vi "myRIO_BRig_RT_v0,44__PortC.vi"() -> ()   [LabVIEW 2014]
uses:
  myRIO_BRig_RT__Case_Exp_stateList.ctl
  myRIO_BRig_RT__Case_NonExp_stateList.ctl
  <vilib>/Platform/TimedLoop/XDataNode/timing_clust.ctl
  <vilib>/Platform/TimedLoop/XDataNode/nitl_modes.ctl
  <vilib>/Platform/TimedLoop/XDataNode/wakeup.ctl
  <vilib>/WebDAVClient/Advanced/SessionHandle.ctl
  <vilib>/myRIO/Common/Instrument Driver Framework/myRIO v1.0/UART/vis/myRIO v1.0 Close UART.vi
  <vilib>/FPGAPlugInAG/myRIO-1900/niLvFpga_Open_myRIO-1900.vi
  <vilib>/rvi/interface/common/dynamic/niFpgaDynamicAddResources.vi
  <vilib>/Utility/error.llb/Error Cluster From Error Code.vi
  <vilib>/rvi/errors/niLvFpgaAdjustHostInterfaceError.vi
  <vilib>/FPGAPlugInAG/Dynamic/niLvFpga_Close_Dynamic.vi
  <vilib>/myRIO/Common/Instrument Driver Framework/Utilities/vis/FPGA Ref Manager.vi
  <vilib>/myRIO/Common/Instrument Driver Framework/myRIO v1.0/myRIO v1.0 Reset FPGA.vi
  <vilib>/myRIO/Common/Instrument Driver Framework/myRIO v1.0/IRQ/vis/myRIO v1.0 IRQ Info FGV.vi
  <vilib>/myRIO/Common/Instrument Driver Framework/myRIO v1.0/IRQ/vis/myRIO v1.0 Timer IRQ Info FGV.vi
  <vilib>/myRIO/Common/Instrument Driver Framework/myRIO v1.0/IRQ/vis/myRIO v1.0 ISR Agent.vi
  <vilib>/rvi/interface/nirviOpenFPGA/nirviOpenFPGA.xnode
  myRIO_BRig_FPGA_v3,40__PortC__build.lvbitx
  myRIO_BRig_FPGA_v3,40.vi
  <vilib>/rvi/interface/nirviReadWriteControl/nirviReadWriteControl.xnode
  <vilib>/Platform/TimedLoop/XDataNode/XDataNode.xnode
  <vilib>/rvi/interface/nirviCloseFPGA/nirviCloseFPGA.xnode
  <vilib>/Platform/TimedLoop/XDataNode/XDNodeRunTimeDep.lvlib
  <vilib>/rvi/interface/Simulation/niFpgaSimulationCallBeginRW.vi
  <vilib>/myRIO/Instrument Drivers/Utilities/Utilities.lvlib
  <vilib>/WebDAVClient/NI_WebDAV.lvlib
  NiFpgaLv.dll
panel:
  in  "laser_power":dbl
  in  "f_millisec2count":dbl=109.0
  in  "laser_Tshutter":dbl=2.0
  in  "laser_Freq":dbl=10.0
  in  "laser_Tpeak":dbl=2.0
  in  "laser_duration":u16
  out "error out":errorcluster
  in  "LC_Cue1_All_Count":u16
  in  "LC_Cue1_First_Count":u16
  in  "LC_Cue1_All_delayOpt":bool
  in  "LC_ENL1_All_delayOpt":bool
  in  "LC_ENL1_All_Count":u16
  in  "LC_ENL1_First_Count":u16
  in  "LC_Cue1_First_delayOpt":bool
  in  "LC_ENL1_First_delayOpt":bool
  in  "Tcycle_Cue_max":u16=1000 caption="Max [ms]" min=5 max=5000 step=5
  in  "Tcycle_Cue_min":u16=1000 caption="Min [ms]" min=5 max=5000 step=5
  in  "SendData":bool
  out "cSpout":enum16{"Left", "Right"}(ring) caption="Left or Right Spout"
  out "A4":u32 caption="LickCounter_Right"
  out "A2":u32 caption="LickCounter_Left"
  in  "tDelay_laser_wro":u32
  in  "tCycle_laser_wro":u32=1000
  in  "tDelay_laser_rew":u32
  in  "laserResponse_wrong_LED":bool
  out "error_initTrial":errorcluster
  out "error_Selection_pre":errorcluster
  out "error_Selection":errorcluster
  in  "tCycle_laser_rew":u32=1000
  out "SelectWrong":bool
  out "SelectReward":bool
  in  "Left(F)_or_Right(T)":bool
  in  "ignoreWrong":bool
  in  "SelectionState":bool
  in  "laserResponse_wrong":bool
  in  "laserResponse_reward":bool
  in  "laserResponse_reward_LED":bool
  out "nRewards_Right":u16 caption="# Rewards Total (Right)"
  out "nRewards_Left":u16 caption="# Rewards Total (Left)"
  out "nRewards_cur":u16 caption="# Rewards in Current Block"
  out "TpB_target":u16 caption="Target Trials Per Block"
  out "cState_NonExp":T1 caption="NonExperimental State"
  out "iBlock":u16 caption="Current Block"
  out "cState":T2 caption="Experimental State"
  out "iTrial":u16 caption="Current Trial"
  in  "warmupType":bool
  in  "TestConnection":bool
  in  "warmup":bool caption="WarmUp"
  in  "Host Filename Prefix":string="Exp1_TM2"
  out "Connected To Host?":bool
  in  "Host Password":string="sabalab"
  in  "Host UserName":string="Test2"
  in  "sp_RightSpout":u16(slide)=2 max=2 step=1 scale=0.0..2.0
  in  "sp_LeftSpout":u16(slide)=2 max=2 step=1 scale=0.0..2.0
  in  "BUR_max":u16 caption="Count Reward Structure  (0 = off)"
  in  "LC_Wrong_Probability":u16
  in  "LC_Wrong_Trial":u16(slide) max=2 step=1 scale=0.0..2.0
  in  "LC_Wrong_Block":u16(slide) max=2 step=1 scale=0.0..2.0
  in  "LC_Wrong_OnOff":bool
  in  "LC_Reward_Probability":u16
  in  "LC_Reward_Trial":u16(slide) max=2 step=1 scale=0.0..2.0
  in  "LC_Reward_Block":u16(slide) max=2 step=1 scale=0.0..2.0
  in  "LC_Reward_OnOff":bool
  in  "LC_Cue1_All_Probability":u16
  in  "LC_Cue1_All_Block":u16(slide) max=2 step=1 scale=0.0..2.0
  in  "LC_Cue1_All_OnOff":bool
  in  "LC_Cue1_First_Probability":u16
  in  "LC_Cue1_First_Block":u16(slide) max=2 step=1 scale=0.0..2.0
  in  "LC_Cue1_First_OnOff":bool
  in  "LC_ENL1_All_Probability":u16 max=100 step=1
  in  "LC_ENL1_All_Block":u16(slide) max=2 step=1 scale=0.0..2.0
  in  "LC_ENL1_All_OnOff":bool
  in  "LC_ENL1_First_Probability":u16 max=100 step=1
  in  "LC_ENL1_First_Block":u16(slide) max=2 step=1 scale=0.0..2.0
  in  "A6":bool caption="Activate Recording?\n(Select Prior to\nStarting Experiment)"
  in  "Tcycle_Timeout":u16=1000 caption="Timeout Time [ms]" min=10 max=10000 step=1
  in  "Tcycle_Wrong":u16=1000 caption="Wrong Time [ms]" min=10 max=10000 step=1
  in  "Tcycle_Selection":u16=1000 caption="Answer Time [ms]" min=1 max=10000 step=1
  in  "Tcycle_RewardPost":u16=1000 caption="Consumption Time [ms]" min=250 max=10000 step=250
  in  "Tcycle_Reward_L":u16=500 caption="Reward Time [ms]" min=1 max=1000 step=1
  in  "Tcycle_Reward_R":u16=500 caption="Reward Time [ms]" min=1 max=1000 step=1
  in  "TpB_Max_R":u16=4 caption="Max TrialsPerBlock" min=1 max=12 step=1
  in  "TpB_Min_R":u16=4 caption="Min TrialsPerBlock" min=1 max=12 step=1
  in  "TpB_Max_L":u16=4 caption="Max TrialsPerBlock" min=1 max=12 step=1
  in  "TpB_Min_L":u16=4 caption="Min TrialsPerBlock" min=1 max=12 step=1
  in  "BUR_min":u16 caption="Count Reward Structure  (0 = off)"
  in  "TrialUntilReward":bool caption="Ignore Wrong \nSelection"
  in  "CueCycles":u16=1 caption="Cue Structure" min=1 max=1 step=1
  in  "MTrig_Laser_Tcycle":u16=10 caption="Time [ms]"
  in  "MTrig_Laser_trig":bool
  in  "MTrig_Audio_trig__R":bool caption="Trigger Audio"
  in  "MTrig_Audio_trig__L":bool caption="Trigger Audio"
  in  "RewCalib_Trig_R":bool caption="Calibrate_R"
  in  "RewCalib_Trig_L":bool caption="Calibrate_L"
  in  "MTrig_Solenoid_Tcycle__R":u16=300 caption="Time [ms]"
  in  "MTrig_Solenoid_Tcycle__L":u16=300 caption="Time [ms]"
  in  "MTrig_Solenoid_trig__R":bool caption="Solenoid"
  in  "MTrig_Solenoid_trig__L":bool caption="Solenoid"
  in  "STOP_abort":bool caption="Stop LabView\n(Stops myRio and FPGA)"
  in  "STOP_endBlock":bool caption="Stop Experiment\n@ End of Block"
  in  "STOP_endTrial":bool caption="Stop Experiment\n@ End of Trial"
  in  "START":bool caption="Start Experiment"
  in  "Tcycle_CuePenalty":u16=1000 caption="Penalty [ms]" min=1 max=10000 step=1
  in  "Audio_Amp__R":u16=100 caption="Amp"
  in  "Audio_Freq__R":u16=5 caption="Freq [kHz]" max=14 step=1
  in  "Audio_Amp__L":u16=100 caption="Amp"
  in  "Audio_Freq__L":u16=5 caption="Freq [kHz]" max=14 step=1
  in  "LC_Wrong_Tdelay":u16
  in  "LC_Cue1_All_Tdelay":u16
  in  "LC_ENL1_All_Tdelay":u16
  in  "LC_Reward_Tdelay":u16
  in  "LC_Cue1_First_Tdelay":u16
  in  "LC_ENL1_First_Tdelay":u16
  in  "LC_ENL1_First_OnOff":bool
  in  "Tcycle_ENLPenalty":u16=100 caption="Penalty [ms]" min=10 max=100 step=10
  in  "Tcycle_ENL_max":u16=1000 caption="Max [ms]" min=250 max=10000 step=250
  in  "Tcycle_ENL_min":u16=1000 caption="Min [ms]" min=250 max=10000 step=250
  # "Manual Control"
  # "Task Structure"
  # "Task Timing"
  # "Laser Control\n\n                                                    On/Off      Block        Probability [%]   Delay [ms]                              Count"
  # "Manual Solenoid Trigger\nLeft              Right"
  # "Master Structure"
  # "Enforced NonLick"
  # "Enforced NonLick 1"
  # "from end"
  # "Time = Cue Min"
  # "Min\n \n  \nMax"
  # "First Trial"
  # "from start"
  # "(1) = Switching\n(2) = Two Choice"
  # "from end"
  # "All Trials"
  # "Cue"
  # "from start"
  # "Cue 1"
  # "from end"
  # "from start"
  # "Cue then reward"
  # "Min"
  # "Max"
  # "from end"
  # "Cue with reward"
  # "Trial Per Block Structure\n       Left                    Right"
  # "from start"
  # "Spout Selection Control"
  # "Manual Speaker Trigger\nLeft              Right"
  # "Selection Reward"
  # "Answer Time\n         [ms]\n\n  \nWrong Choice Penalty\n         [ms]\n \n \nChoice Timeout Penalty\n         [ms]"
  # "Selection Wrong"
  # "Cue Control"
  # "Left              Right"
  # "State"
  # "Manual Laser Trigger"
  # "Freq [kHz]\n \n \nAmp\n \n\n \n\nSpeaker\nSetting"
  # "Reward Control\n                 Left              Right"
  # "Min = 1\nMax = 32k"
  # "Reward Time\n         [ms]"
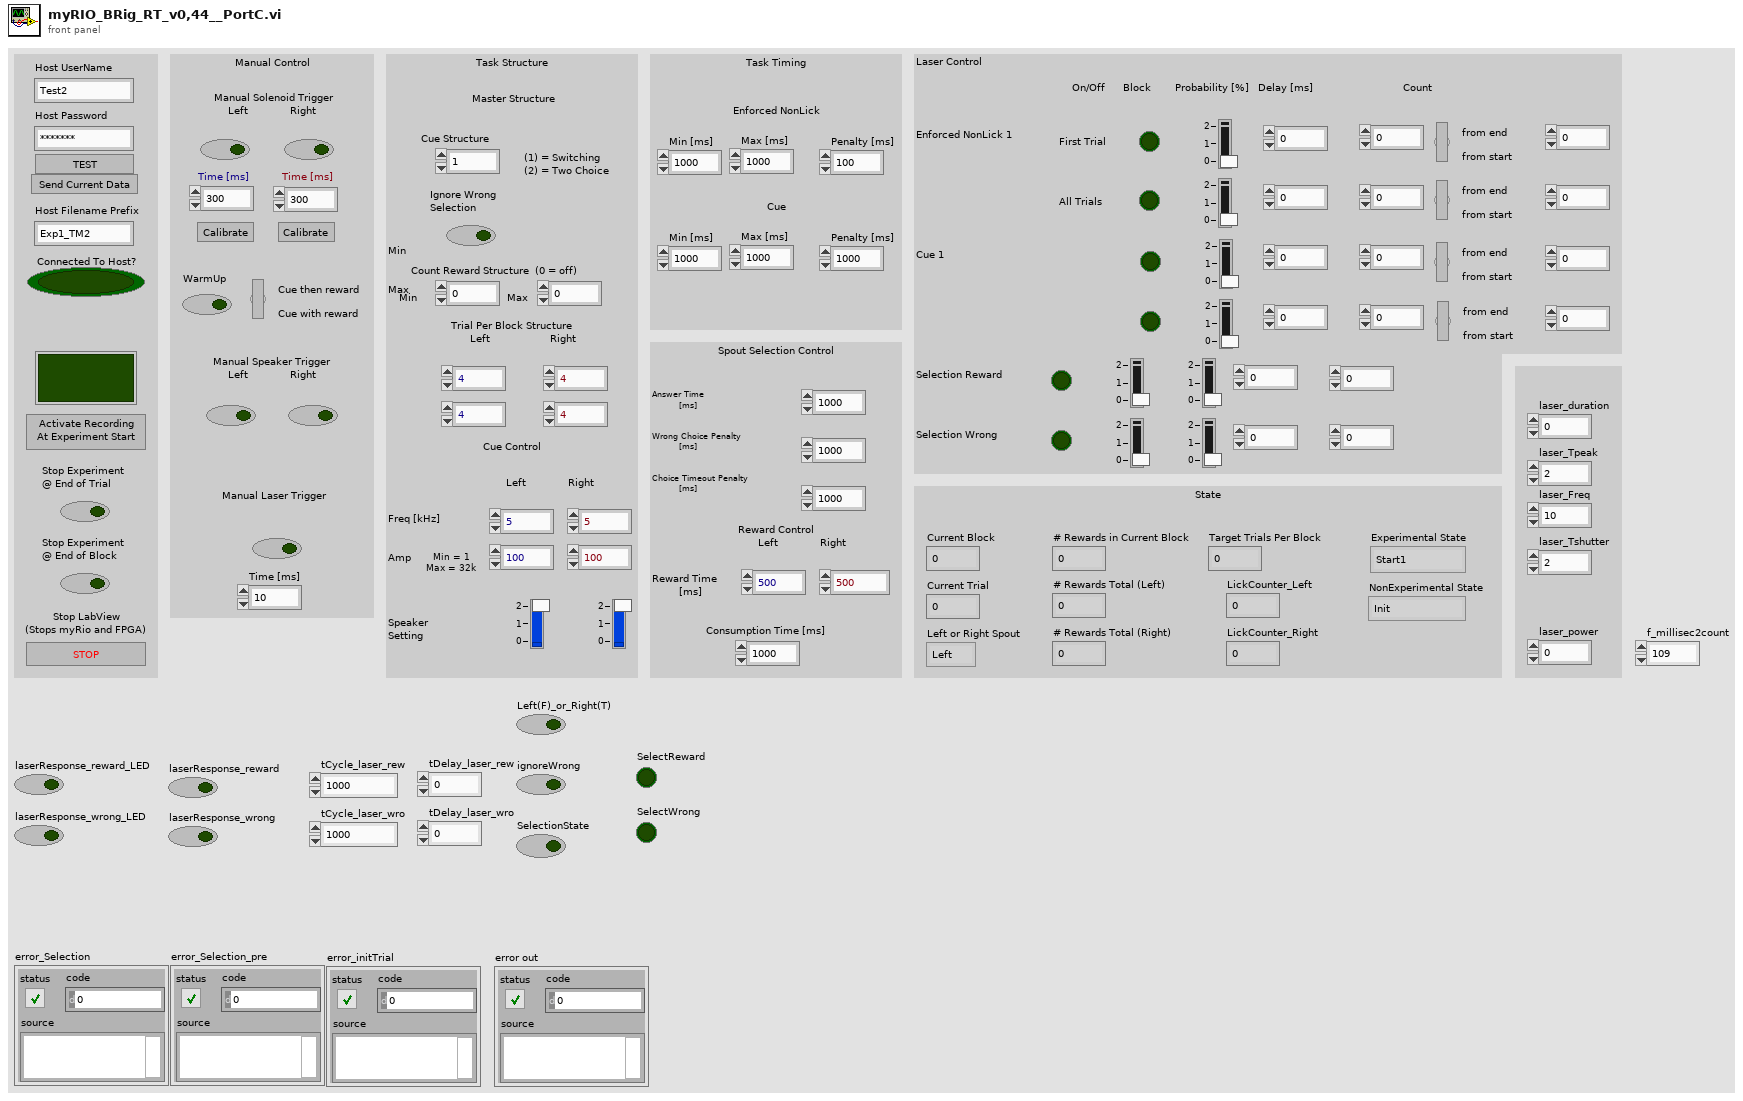
[diagram p1: front panel]
types:
  T1 = typedef "myRIO_BRig_RT__Case_NonExp_stateList.ctl" = enum16{"Init", "UploadSettings_pre", "UploadSettings_Read_dataExp", "UploadSettings_dataExp_1", "UploadSettings_Read_dataLC", "UploadSettings_dataLC_1", "UploadSettings_dataLC_2", "UploadSettings_Read_dataMTrig", "UploadSettings_dataMTrig_1", "UploadSettings_post", "Idle_pre", "IdleEmpty", "IdleEmpty2", "IdleEmpty3", "IdleEmpty4", "Idle", "Idle_2", "Idle_3", "Idle_4", "Idle_post", "Cue_pre__pre", "Cue_pre", "Cue", "Cue_post", "RewardCalibration_pre", "DispenseWater_pre__pre", "DispenseWater_pre", "DispenseWater", "DispenseWater_post", "TestConnection", "SendData", "End"}
  T2 = typedef "myRIO_BRig_RT__Case_Exp_stateList.ctl" = enum16{"Start1", "Start2", "Start3", "saveSettings1", "saveSettings2", "saveSettings3", "saveSettings4_LC_ENL", "saveSettings5_LC_Cue", "saveSettings6_LC_Other", "setSettings_Audio", "setSettings_Laser", "initBlock_pre", "initBlock", "initBlock2", "initBlock_post", "initTrial_pre", "initTrial", "initTrial2", "initTrial3", "initTrial4", "initTrial_LC_ENL1", "initTrial_LC_Cue1", "initTrial_post", "ENL1_pre", "ENL1", "ENL1_post", "ENL1Penalty_pre", "ENL1Penalty", "ENL2_pre", "ENL2", "ENL2Penalty_pre", "ENL2Penalty", "Cue1_pre", "Cue1", "Cue1_post", "Cue1Penalty_pre", "Cue1Penalty", "Cue2_pre", "Cue2", "Cue2Penalty_pre", "Cue2Penalty", "Selection_pre", "Selection", "Select_post", "SelectReward_pre", "SelectReward", "SelectRewardPost_pre", "SelectRewardPost", "SelectWrong_pre", "SelectWrong", "SelectWrong_post", "SelectTimeout_pre", "SelectTimeout", "SelectTimeout_post", "endTrial_pre", "endTrial1", "endTrial2", "endTrial3", "endTrial_post", "endBlock_pre", "endBlock", "endBlock_post", "endExp", "commConnect", "commUpload_pre", "commUpload_dataBlock", "commUpload_dataCurrent", "commUpload_dataExp", "commUpload_dataLC", "commUpload_dataTrial", "commUpload_post", "saveData_pre", "saveData_dataBlock", "saveData_dataCurrent", "saveData_dataExp", "saveData_dataLC", "saveData_dataTrial", "saveData_post"}
  T3 = typedef "XDNodeRunTimeDep.lvlib/timing_clust.ctl" = cluster{"Expected End [f-1]":u64, "Actual End [f-1]":u64, "Finished Late? [f-1]":bool, "Expected End [i-1]":u64, "Actual End [i-1]":u64, "Finished Late? [i-1]":bool, "Expected Start [i]":u64, "Actual Start [i]":u64, "Expected Start [f]":u64, "Actual Start [f]":u64, "Source Name":string, "Structure Name":string, "Period":i64, "Deadline":i64, "Offset":i64, "Start":i64, "Priority":i32, "Timeout":i32, "Mode":T4, "Wakeup Reason":T5, "Error":errorcluster, "Source Type":string, "Secondary Source Type":string, "Global End Time":u64, "Global Start Time":u64, "Frame Duration":u64, "Iteration Duration":u64, "Assigned CPU":i32, "I/O Scan Engine Mode":u32}
  T4 = typedef "XDNodeRunTimeDep.lvlib/nitl_modes.ctl" = enum32{"No Change", "Process missed periods, maintain original phase", "Discard missed periods, maintain original phase", "Process missed periods, ignore original phase", "Discard missed periods, ignore original phase"}
  T5 = typedef "XDNodeRunTimeDep.lvlib/wakeup.ctl" = enum32{"Normal", "Aborted", "Asynchronous wakeup", "Timing source error", "Timed loop error", "Timeout"}
  T6 = typedef "NI_WebDAV.lvlib/SessionHandle.ctl" = refnum<k1>
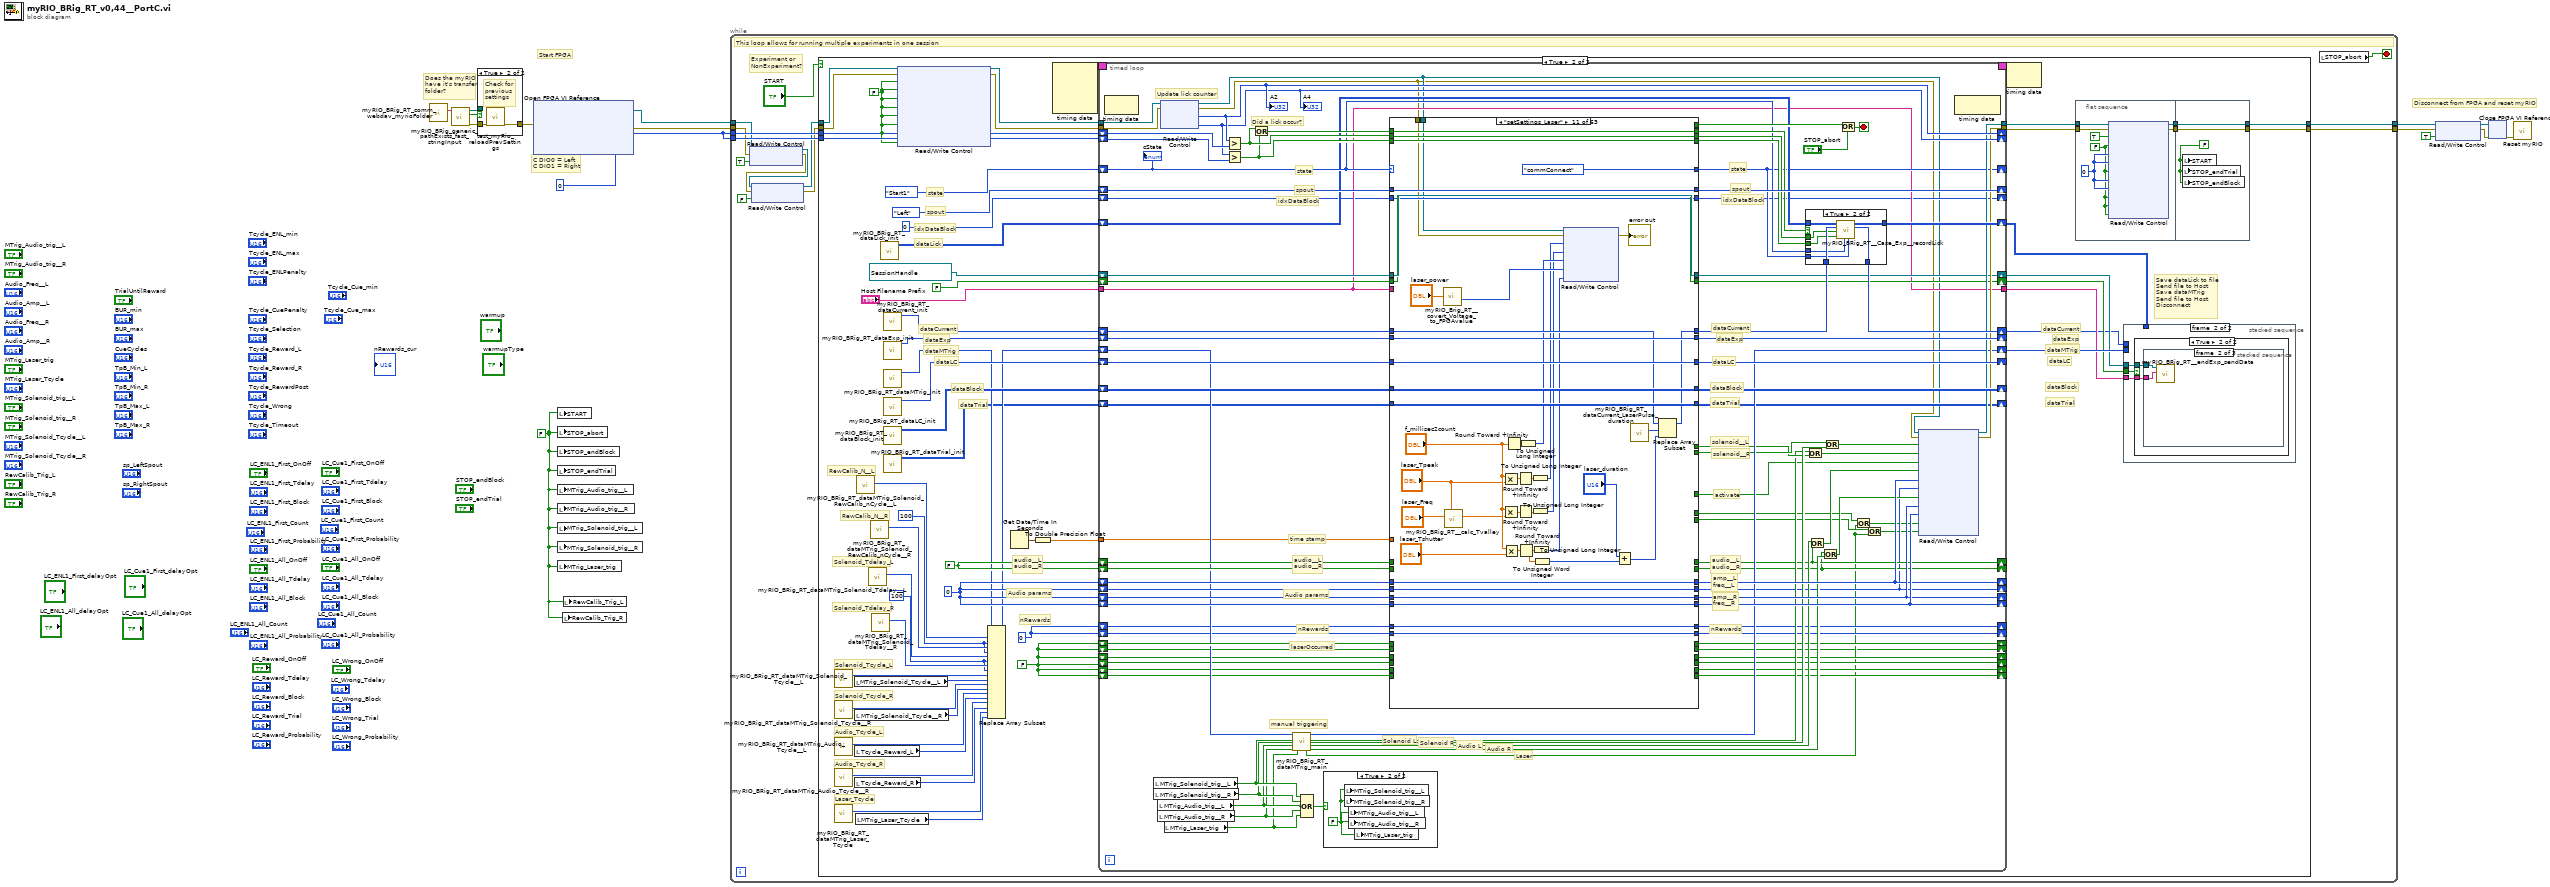
[diagram p0: block diagram]
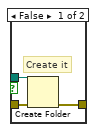
[diagram p2: hidden frame]
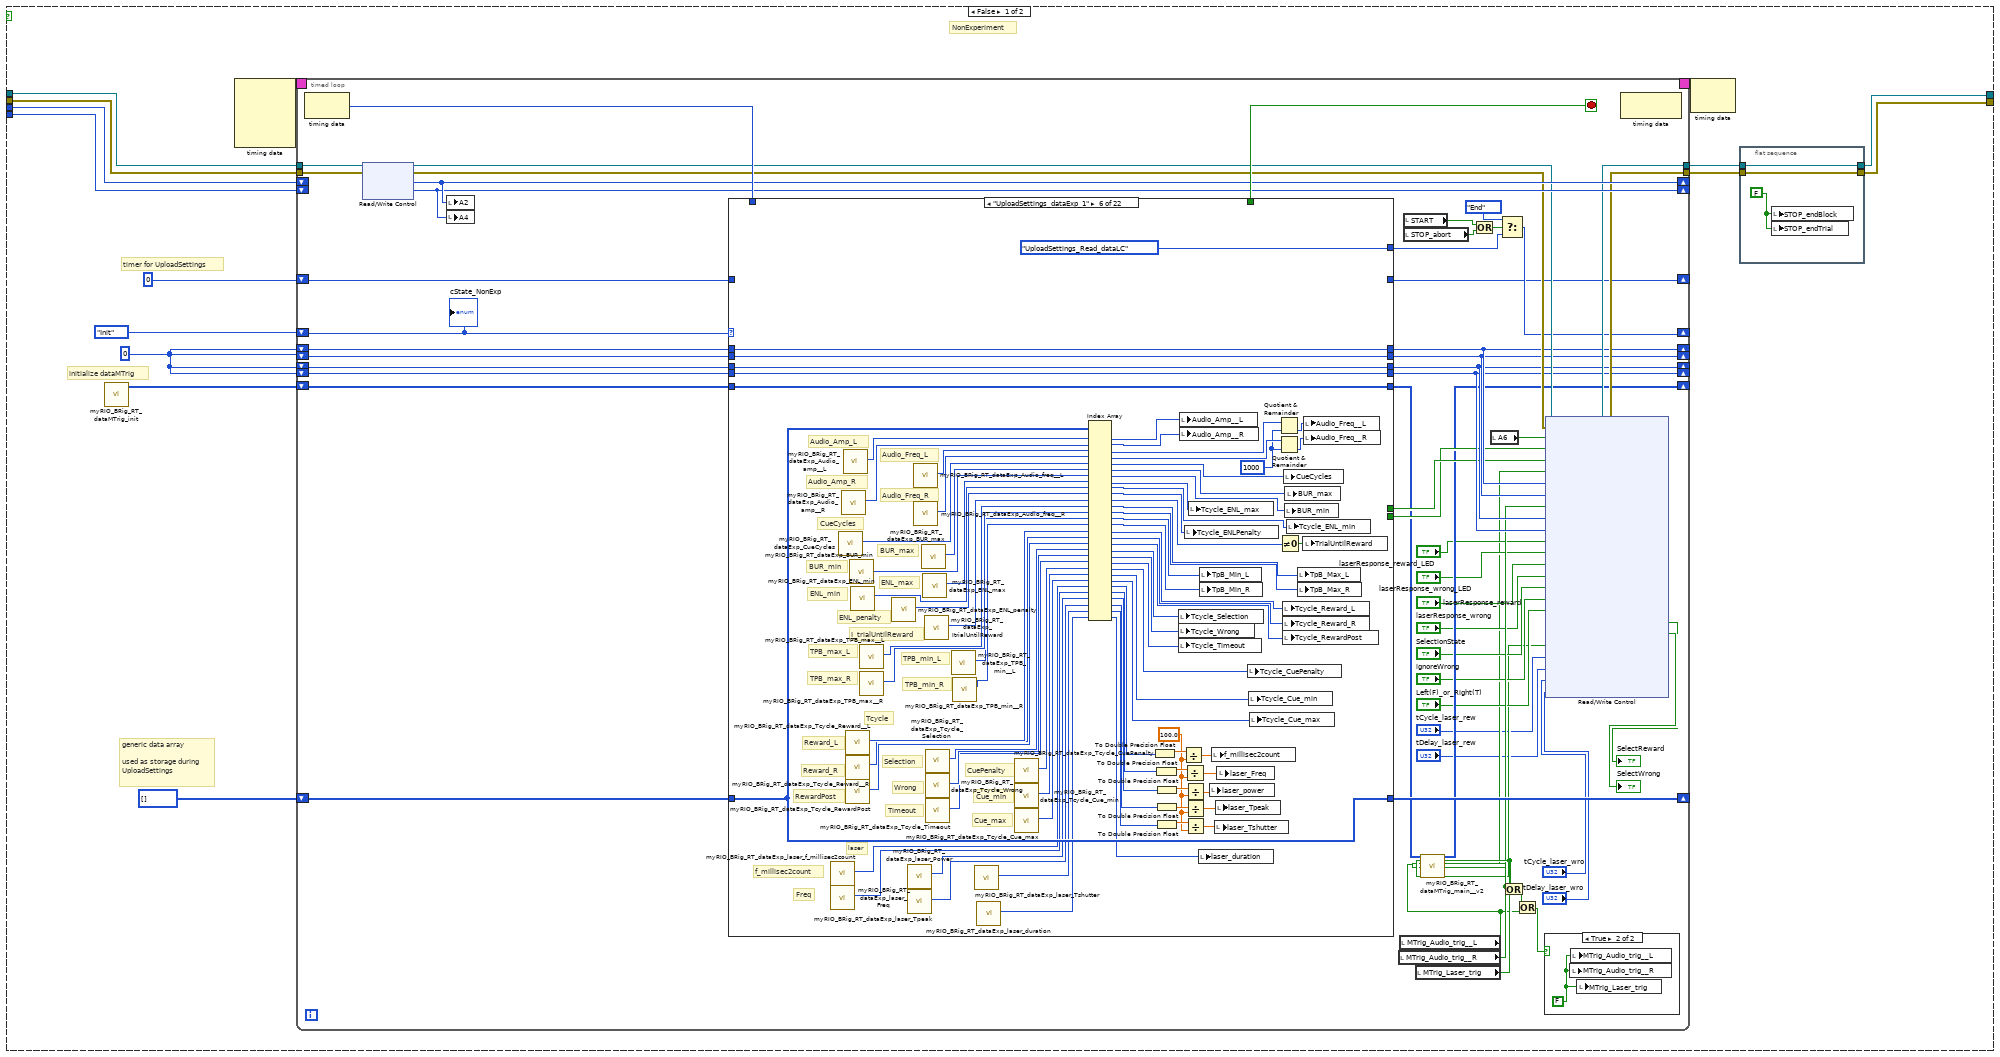
[diagram p3: hidden frame]
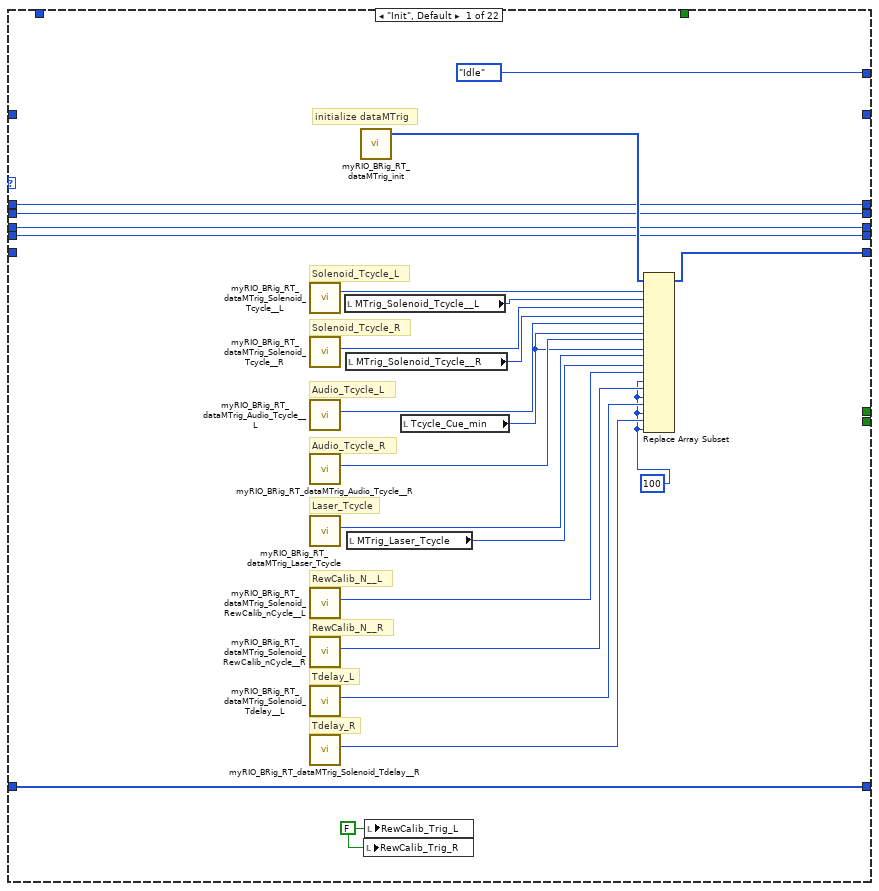
[diagram p5: hidden frame]
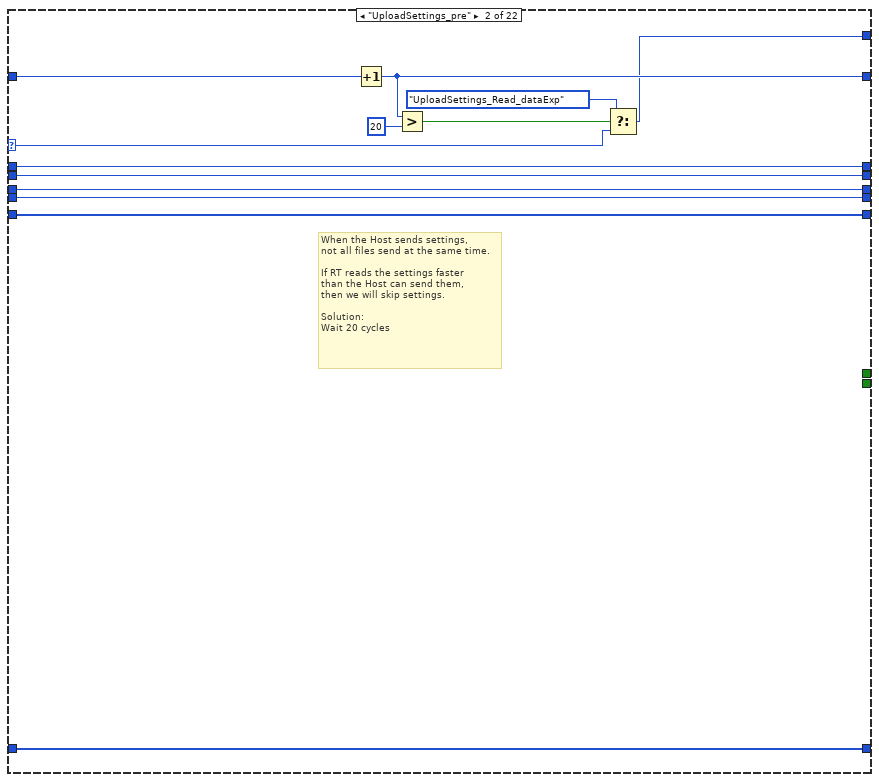
[diagram p6: hidden frame]
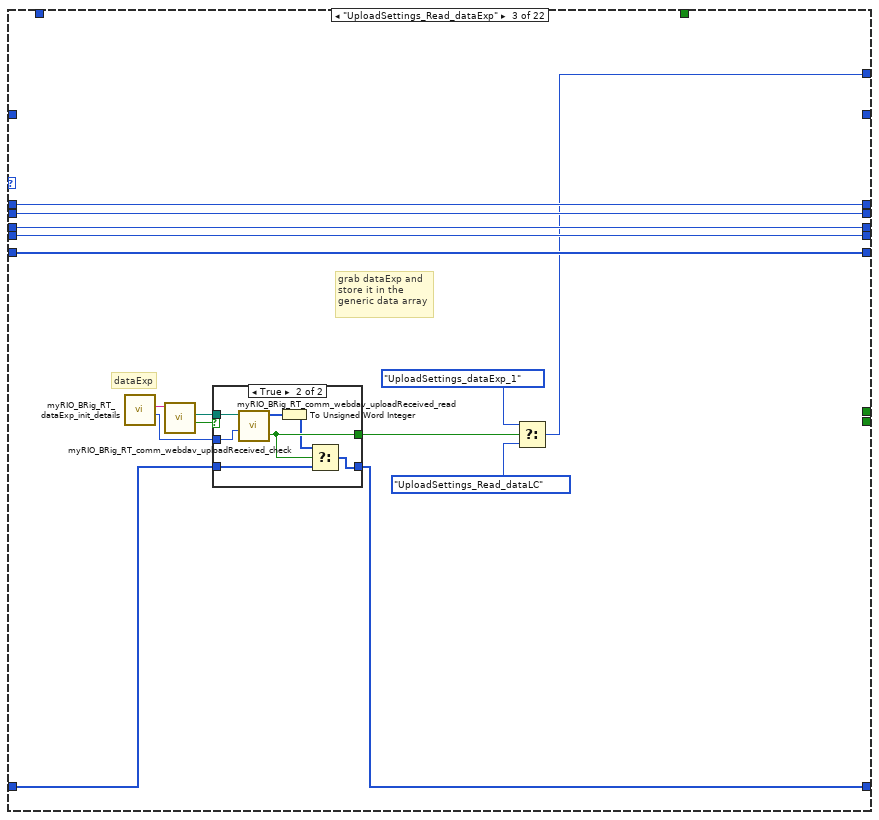
[diagram p7: hidden frame]
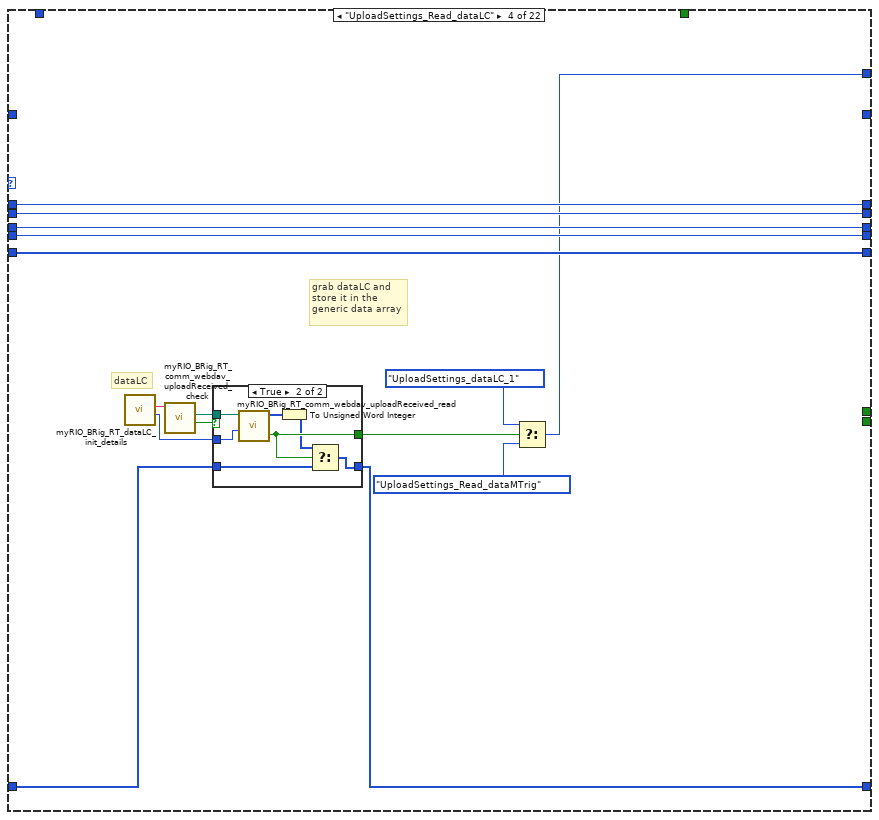
[diagram p9: hidden frame]
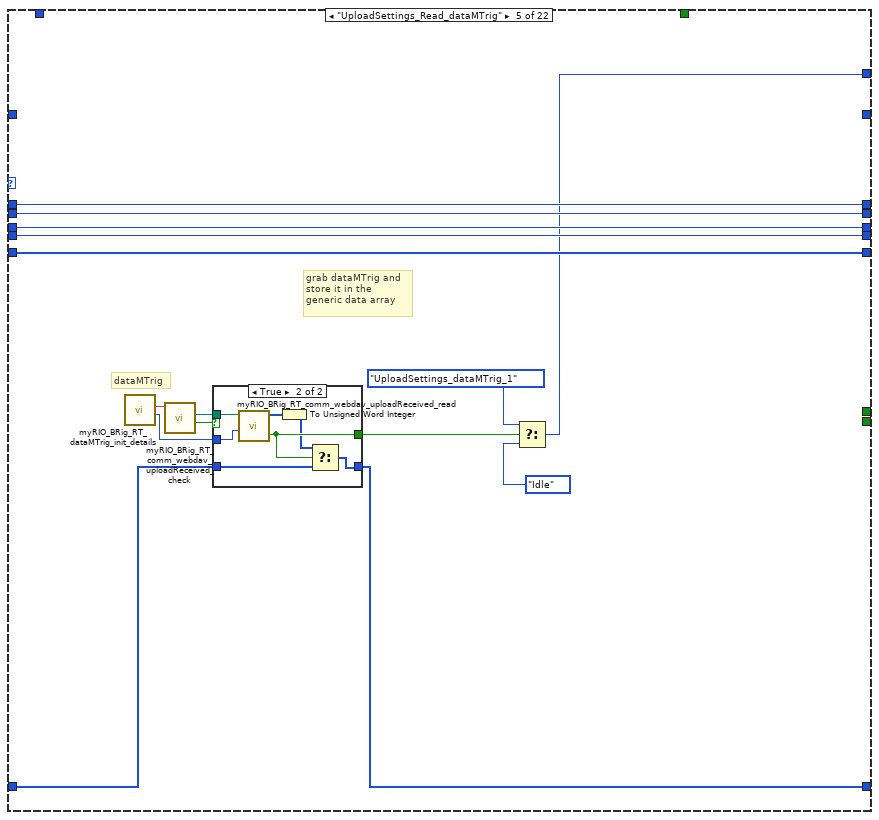
[diagram p11: hidden frame]
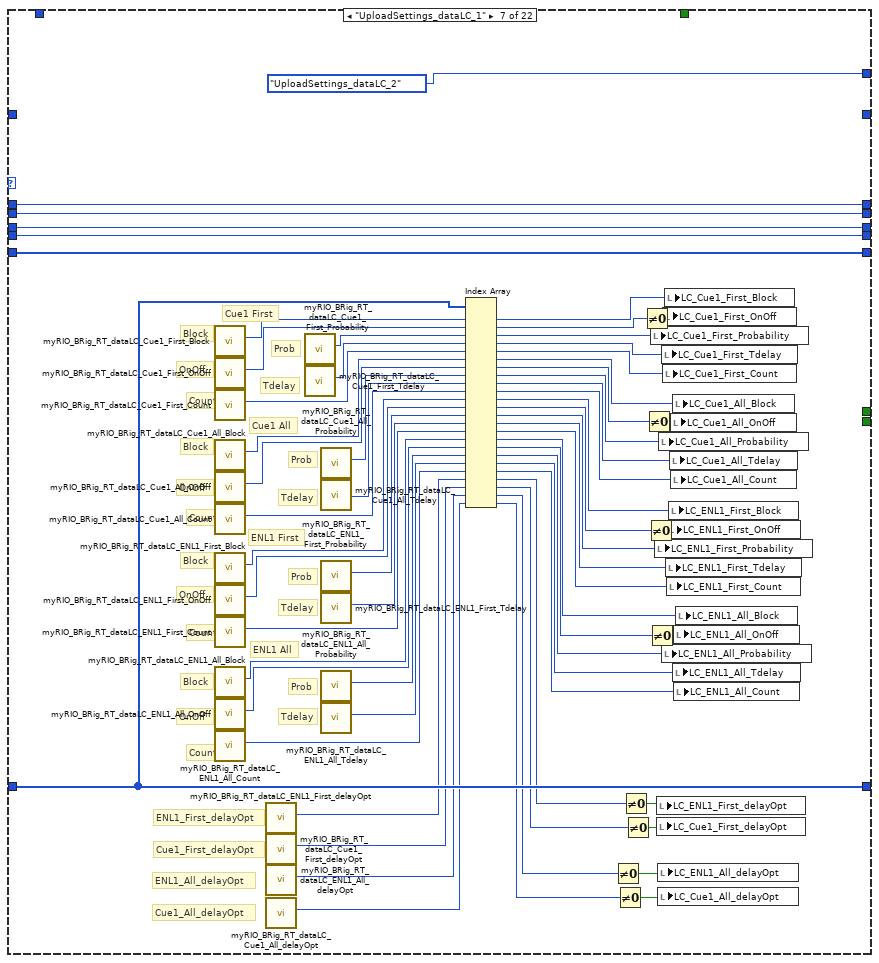
[diagram p13: hidden frame]
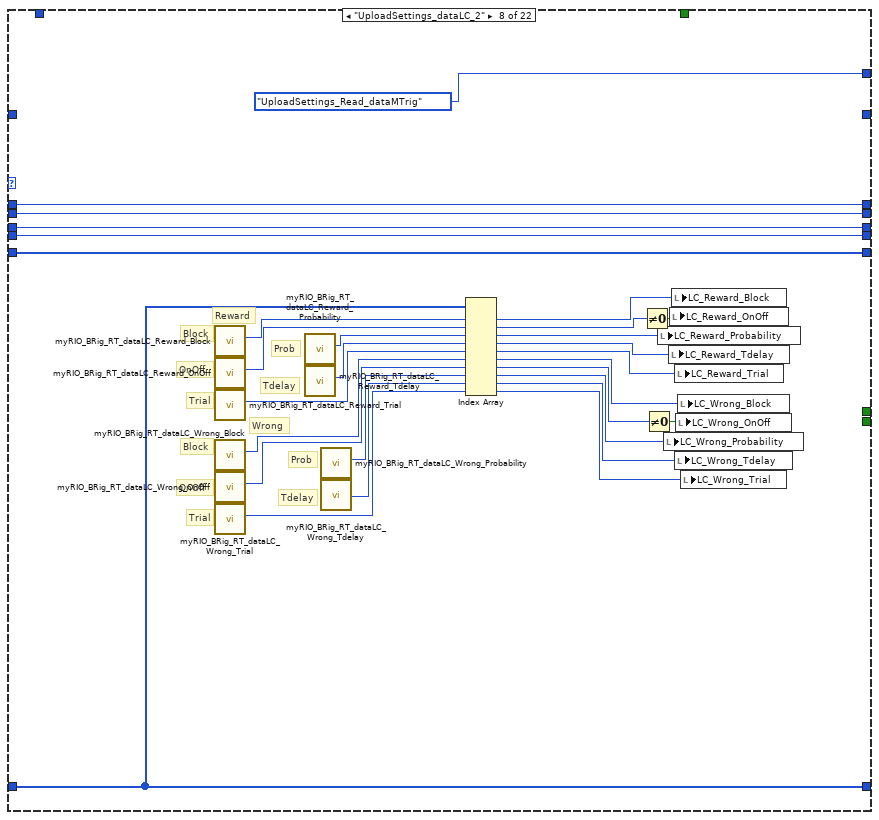
[diagram p14: hidden frame]
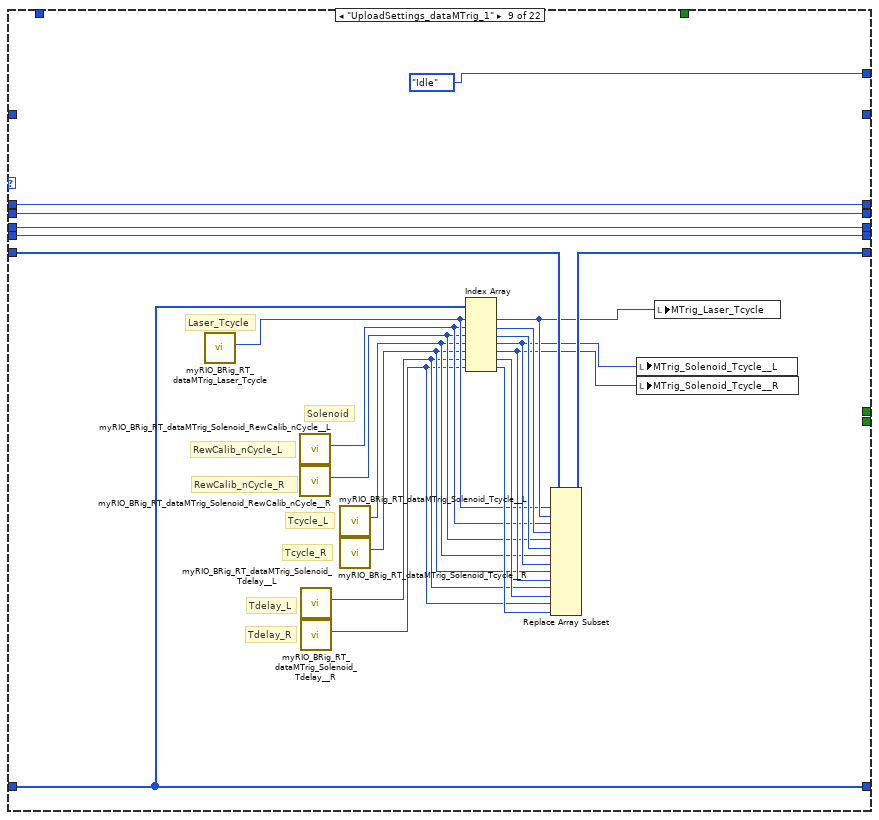
[diagram p15: hidden frame]
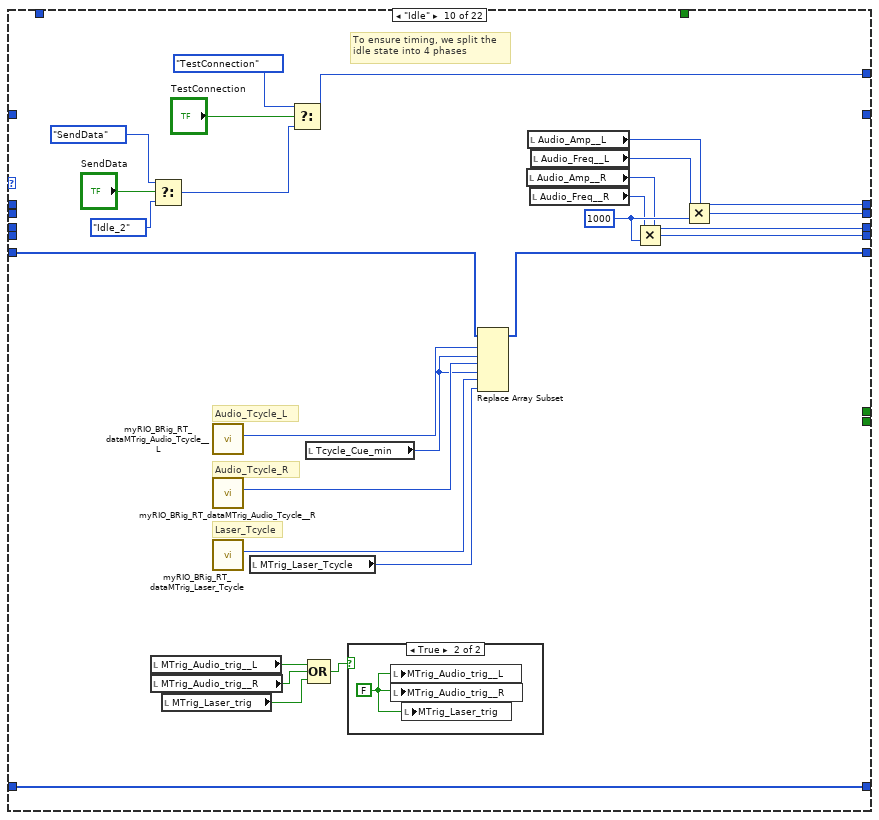
[diagram p16: hidden frame]
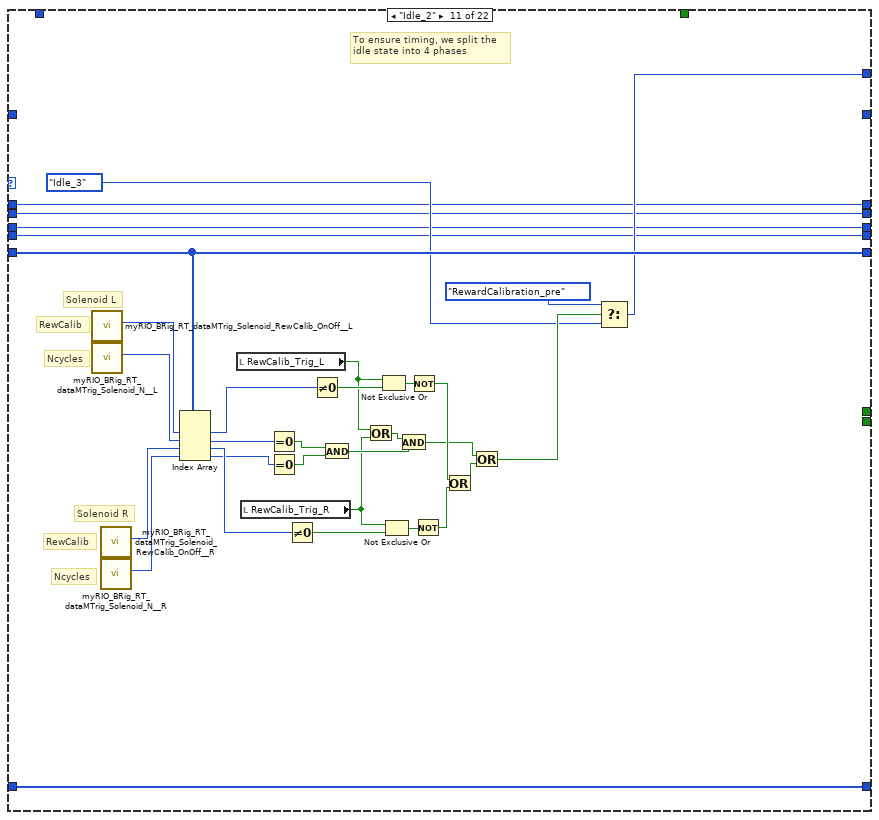
[diagram p18: hidden frame]
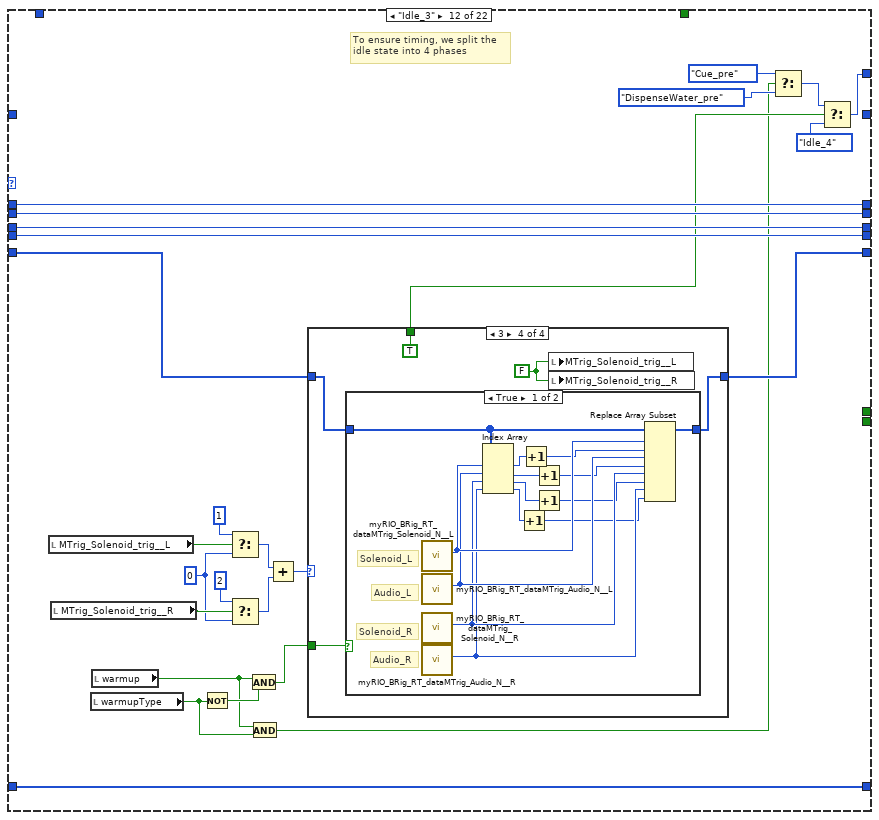
[diagram p19: hidden frame]
diagram:
  w9 = u32 0
  w6 = FALSE
  # "Does the myRIO\nhave it's transfer\nfolder?"
  # "C DIO0 = Left\nC DIO1 = Right"
  # "Start FPGA"
  # "Disconnect from FPGA and reset myRIO"
  n1 = call "myRIO_BRig_RT_comm_webdav_myrioFolder.vi"() -> ("output_myrioFolder"=w4:string)  [unwired: 11 in]
  n2 = call "myRIO_BRig_generic_pathExists_fast_stringInput.vi"("input_filePath"=w4) -> ("output_error"=w3:errorcluster, "output_Iexist"=w2:bool, "output_filePath"=w1:path)  [unwired: 8 in]
  n3 = case shown="True" w2 {
    tunnel: w1 -> [w18 _]
    tunnel: w3 -> [w17 w20]
    tunnel: [w16 w19] -> w5
    frame False {
      # "Create it"
      n4 = Create Folder(path (use dialog)=w18, error in=w17) -> (error out=w16:errorcluster)  [unwired: 1 in, 2 out]
    }
    frame True {
      # "Check for\nprevious\nsettings"
      n5 = call "test_myRio_reloadPrevSettings.vi"("input_error"=w20) -> ("output_error"=w19:errorcluster)  [unwired: 10 in]
    }
  }
  n6 = xnode "Open FPGA VI Reference"("error in"=w5) -> ("FPGA VI Reference Out"=w11:refnum<k20>, "error out"=w10:errorcluster)  [unwired: 1 in]
  n7 = local write "START"(w6) -> ()
  n8 = local write "STOP_abort"(w6) -> ()
  n9 = local write "STOP_endBlock"(w6) -> ()
  n10 = local write "STOP_endTrial"(w6) -> ()
  n11 = local write "MTrig_Audio_trig__L"(w6) -> ()
  n12 = local write "MTrig_Audio_trig__R"(w6) -> ()
  n13 = local write "MTrig_Solenoid_trig__L"(w6) -> ()
  n14 = local write "MTrig_Solenoid_trig__R"(w6) -> ()
  n15 = local write "MTrig_Laser_trig"(w6) -> ()
  n16 = local write "RewCalib_Trig_R"(w6) -> ()
  n17 = local write "RewCalib_Trig_L"(w6) -> ()
  n18 = while {
    tunnel: w11 -> [w24]
    tunnel: w10 -> [w29]
    tunnel: w9 -> [w32]
    tunnel: w9 -> [w31]
    tunnel: [w22] -> w8
    tunnel: [w21] -> w7
    stop <- w30 stop-if-true
    # "Experiment or\nNonExperiment?"
    # "This loop allows for running multiple experiments in one session"
    n19 = xnode "Read/Write Control"("FPGA VI Reference In"=w24, "error in"=w29, "Counts_Reset"=TRUE) -> ("FPGA VI Reference Out"=w26:refnum<k20>, "error out"=w27:errorcluster)
    n20 = xnode "Read/Write Control"("FPGA VI Reference In"=w26, "error in"=w27, "Counts_Reset"=FALSE) -> ("FPGA VI Reference Out"=w23:refnum<k20>, "error out"=w25:errorcluster)
    n21 = case shown="True" "START" {
      tunnel: w32 -> [w45 w937]
      tunnel: w31 -> [w44 w936]
      tunnel: w25 -> [w42 w887]
      tunnel: w23 -> [w43 w886]
      tunnel: [w40 w933] -> w22
      tunnel: [w38 w928] -> w21
      frame False {
        w37 = u16 0 ("Audio_Amp__L")
        # "generic data array\n\nused as storage during\nUploadSettings"
        # "timer for UploadSettings"
        # "initialize dataMTrig"
        # "NonExperiment"
        n22 = call "myRIO_BRig_RT_dataMTrig_init.vi"() -> ("output_dataMTrig"=w46:u16[])  [unwired: 5 in]
        n23 = node-c288() -> (w49:T3)  [unwired: 4 in]
        n24 = timed-loop {
          timing: w49 -> [_]
          timing-out: [_] -> w48
          shift-right: [w83] -> _
          shift-left: w46 -> [w107]
          shift-right: [w72] -> _
          shift-left: myRIO_BRig_RT__Case_NonExp_stateList."Init" ("Enum") -> [w97]
          shift-right: [w105] -> _
          shift-left: w45 -> [_]
          shift-right: [w104] -> _
          shift-left: w44 -> [_]
          tunnel: [w100] -> w41
          tunnel: [w98] -> w39
          tunnel: w42 -> [w103]
          tunnel: w43 -> [w102]
          shift-right: [w96] -> _
          shift-left: u16[] [] ("output_data") -> [w95]
          shift-right: [w90] -> _
          shift-left: w37 -> [w94]
          shift-right: [w89] -> _
          shift-left: w37 -> [w93]
          shift-right: [w88] -> _
          shift-left: w37 -> [w92]
          shift-right: [w87] -> _
          shift-left: w37 -> [w91]
          shift-right: [w54] -> _
          shift-left: u16 0 ("Audio_Amp__L") -> [w55]
          stop <- w108 stop-if-true
          n25 = node-c288() -> (w106:i64)  [unwired: 1 in]
          n26 = xnode "Read/Write Control"("FPGA VI Reference In"=w102, "error in"=w103) -> ("FPGA VI Reference Out"=w101:refnum<k20>, "error out"=w99:errorcluster, "A2_LickL"=w105:u32, "A4_LickR"=w104:u32)
          n27 = local write "A2"(w105) -> ()
          n28 = local write "A4"(w104) -> ()
          n29 = case shown="\"UploadSettings_dataExp_1\"" w97 {
            selector: w97 -> [_ w141 _ _ _ _ _ _ _ _ _ _ _ _ w596 _ _ w781 _ _ _ w878]
            tunnel: [myRIO_BRig_RT__Case_NonExp_stateList."Idle" ("Enum") w139 w146 w169 w192 myRIO_BRig_RT__Case_NonExp_stateList."UploadSettings_Read_dataLC" ("Enum") myRIO_BRig_RT__Case_NonExp_stateList."UploadSettings_dataLC_2" ("Enum") myRIO_BRig_RT__Case_NonExp_stateList."UploadSettings_Read_dataMTrig" ("f") myRIO_BRig_RT__Case_NonExp_stateList."Idle" ("Enum") w422 w443 w476 w567 myRIO_BRig_RT__Case_NonExp_stateList."Cue" ("t") w595 myRIO_BRig_RT__Case_NonExp_stateList."DispenseWater_pre" ("Enum") w723 w779 w806 myRIO_BRig_RT__Case_NonExp_stateList."Idle" ("Enum") myRIO_BRig_RT__Case_NonExp_stateList."Idle" ("Enum") w878] -> w73
            tunnel: [w124 w134 w156 w179 w202 w296 w359 w388 w408 w433 w458 w487 w565 w583 w609 w633 w760 w786 w817 w860 w870 w876] -> w84
            tunnel: [_ _ _ _ _ _ _ _ _ _ _ _ _ _ _ _ _ _ _ _ _ TRUE] -> w108
            tunnel: w107 -> [_ w134 w156 w179 w202 w296 w359 w388 w409 w432 w458 w488 w565 w584 w609 w619 w756 w787 w818 w860 w870 w876]
            tunnel: w106 -> [_ _ _ _ _ _ _ _ _ _ _ _ _ _ _ _ _ w791 _ _ _ _]
            tunnel: [w113 w133 w147 w170 w193 w240 w311 w360 w389 w417 w438 w470 w560 w571 w594 w610 w708 w764 w799 w848 w864 w871] -> w96
            tunnel: w95 -> [w113 w133 w148 w171 w194 w240 w311 w360 w389 w417 w438 w470 w560 w571 w594 w610 w708 w764 w799 w848 w864 w871]
            tunnel: [w117 w137 w159 w182 w205 w293 w357 w363 w406 w428 w441 w480 w562 w591 w606 w613 w762 w797 w824 w851 w867 w874] -> w89
            tunnel: [w115 w135 w157 w180 w203 w291 w355 w361 w404 w427 w439 w482 w564 w589 w608 w611 w761 w795 w822 w849 w865 w872] -> w87
            tunnel: [w118 w138 w160 w183 w206 w294 w358 w364 w407 w426 w442 w479 w561 w593 w605 w614 w763 w798 w825 w852 w868 w875] -> w90
            tunnel: [w116 w136 w158 w181 w204 w292 w356 w362 w405 w425 w440 w481 w563 w590 w607 w612 w761 w796 w823 w850 w866 w873] -> w88
            tunnel: w94 -> [w118 w138 w160 w183 w206 w294 w358 w364 w407 _ w442 w479 w561 w593 w605 w614 w763 w798 w825 w852 w868 w875]
            tunnel: w93 -> [w117 w137 w159 w182 w205 w293 w357 w363 w406 _ w441 w480 w562 w591 w606 w613 w762 w797 w824 w851 w867 w874]
            tunnel: w92 -> [w116 w136 w158 w181 w204 w292 w356 w362 w405 _ w440 w481 w563 w590 w607 w612 w761 w796 w823 w850 w866 w873]
            tunnel: w91 -> [w115 w135 w157 w180 w203 w291 w355 w361 w404 _ w439 w482 w564 w589 w608 w611 _ w795 w822 w849 w865 w872]
            tunnel: [_ _ _ _ _ _ _ _ _ _ _ _ _ _ _ _ _ w788 _ _ _ _] -> w86
            tunnel: [_ _ _ _ _ _ _ _ _ _ _ _ _ _ _ _ _ w770 _ _ _ _] -> w85
            tunnel: w55 -> [_ w145 _ _ _ _ _ _ _ _ _ _ _ _ _ _ _ _ _ _ _ _]
            tunnel: [_ w144 _ _ _ _ _ _ _ _ _ _ _ _ _ _ _ _ _ _ _ _] -> w54
            frame "Init", Default {
              w114 = FALSE ("RewCalib_Trig_L")
              w110 = u16 100 ("new element/subarray")
              # "Tdelay_R"
              # "Tdelay_L"
              # "RewCalib_N__R"
              # "RewCalib_N__L"
              # "Solenoid_Tcycle_R"
              # "Solenoid_Tcycle_L"
              # "Laser_Tcycle"
              # "Audio_Tcycle_R"
              # "Audio_Tcycle_L"
              # "initialize dataMTrig"
              n30 = call "myRIO_BRig_RT_dataMTrig_Solenoid_Tcycle__L.vi"() -> ("output_Solenoid_Tcycle__L"=w126:i32)  [unwired: 11 in]
              n31 = call "myRIO_BRig_RT_dataMTrig_Solenoid_Tcycle__R.vi"() -> ("output_Solenoid_Tcycle__R"=w127:i32)  [unwired: 11 in]
              n32 = call "myRIO_BRig_RT_dataMTrig_Audio_Tcycle__L.vi"() -> ("output_Audio_Tcycle__L"=w128:i32)  [unwired: 11 in]
              n33 = call "myRIO_BRig_RT_dataMTrig_Audio_Tcycle__R.vi"() -> ("output_Audio_Tcycle__R"=w129:i32)  [unwired: 11 in]
              n34 = call "myRIO_BRig_RT_dataMTrig_Laser_Tcycle.vi"() -> ("output_Laser_Tcycle"=w130:i32)  [unwired: 11 in]
              n35 = call "myRIO_BRig_RT_dataMTrig_Solenoid_RewCalib_nCycle__L.vi"() -> ("output_Solenoid_RewCalib_nCycle__L"=w122:i32)  [unwired: 11 in]
              n36 = call "myRIO_BRig_RT_dataMTrig_Solenoid_RewCalib_nCycle__R.vi"() -> ("output_Solenoid_RewCalib_nCycle__R"=w121:i32)  [unwired: 11 in]
              n37 = call "myRIO_BRig_RT_dataMTrig_Solenoid_Tdelay__L.vi"() -> ("output_Solenoid_Tdelay__L"=w120:i32)  [unwired: 11 in]
              n38 = call "myRIO_BRig_RT_dataMTrig_Solenoid_Tdelay__R.vi"() -> ("output_Solenoid_Tdelay__R"=w119:i32)  [unwired: 11 in]
              n39 = local read "MTrig_Solenoid_Tcycle__L"() -> (w131:u16)
              n40 = local read "MTrig_Solenoid_Tcycle__R"() -> (w132:u16)
              n41 = local read "MTrig_Laser_Tcycle"() -> (w111:u16)
              n42 = call "myRIO_BRig_RT_dataMTrig_init.vi"() -> ("output_dataMTrig"=w125:u16[])  [unwired: 5 in]
              n43 = local write "RewCalib_Trig_R"(w114) -> ()
              n44 = local write "RewCalib_Trig_L"(w114) -> ()
              n45 = local read "Tcycle_Cue_min"() -> (w112:u16)
              n46 = Replace Array Subset(array=w125, new element #1=w131, index #1=w126, new element #2=w132, index #2=w127, new element #3=w112, index #3=w128, new element #4=w112, index #4=w129, new element #5=w111, index #5=w130, new element #6=w110, index #6=w122, new element #7=w110, index #7=w121, new element #8=w110, index #8=w120, new element #9=w110, index #9=w119) -> (w124:u16[])
            }
            frame "UploadSettings_pre" {
              # "When the Host sends settings,\nnot all files send at the same time.\n\nIf RT reads the settings faster\nthan the Host can send them,\nthen we will skip settings.\n\nSolution:\nWait 20 cycles"
              n47 = Increment(x=w145) -> (x+1=w144:u16)
              n48 = Greater?(x=w144, y=u16 20) -> (0:w142:bool)
              n49 = Select(t=myRIO_BRig_RT__Case_NonExp_stateList."UploadSettings_Read_dataExp", s=w142, f=w141) -> (s? t:f=w139:T1)
            }
            frame "UploadSettings_Read_dataExp" {
              # "grab dataExp and\nstore it in the\ngeneric data array"
              # "dataExp"
              n50 = call "myRIO_BRig_RT_dataExp_init_details.vi"() -> ("output_dataSize"=w152:i32, "output_dataName"=w155:string)  [unwired: 10 in]
              n51 = call "myRIO_BRig_RT_comm_webdav_uploadReceived_check.vi"("input_dataName"=w155) -> ("output_Iexist"=w154:bool, "output_dataPath"=w153:path)  [unwired: 9 in]
              n52 = case shown="True" w154 {
                tunnel: w153 -> [_ w168]
                tunnel: w152 -> [_ w167]
                tunnel: [_ w166] -> w151
                tunnel: w148 -> [w161 w165]
                tunnel: [w161 w162] -> w147
                frame False {
                }
                frame True {
                  n53 = call "myRIO_BRig_RT_comm_webdav_uploadReceived_read.vi"("input_dataSize"=w167, "input_filePath"=w168) -> ("output_Ivalid"=w166:bool, "output_data"=w164:i64[])  [unwired: 8 in]
                  n54 = To Unsigned Word Integer(number=w164) -> (unsigned 16bit integer=w163:u16[])
                  n55 = Select(t=w163, s=w166, f=w165) -> (s? t:f=w162:u16[])
                }
              }
              n56 = Select(t=myRIO_BRig_RT__Case_NonExp_stateList."UploadSettings_dataExp_1", s=w151, f=myRIO_BRig_RT__Case_NonExp_stateList."UploadSettings_Read_dataLC" ("t")) -> (s? t:f=w146:T1)
            }
            frame "UploadSettings_Read_dataLC" {
              # "grab dataLC and\nstore it in the\ngeneric data array"
              # "dataLC"
              n57 = call "myRIO_BRig_RT_dataLC_init_details.vi"() -> ("output_dataSize"=w175:i32, "output_dataName"=w178:string)  [unwired: 10 in]
              n58 = call "myRIO_BRig_RT_comm_webdav_uploadReceived_check.vi"("input_dataName"=w178) -> ("output_Iexist"=w177:bool, "output_dataPath"=w176:path)  [unwired: 9 in]
              n59 = case shown="True" w177 {
                tunnel: w176 -> [_ w191]
                tunnel: w175 -> [_ w190]
                tunnel: [_ w189] -> w174
                tunnel: w171 -> [w184 w188]
                tunnel: [w184 w185] -> w170
                frame False {
                }
                frame True {
                  n60 = call "myRIO_BRig_RT_comm_webdav_uploadReceived_read.vi"("input_dataSize"=w190, "input_filePath"=w191) -> ("output_Ivalid"=w189:bool, "output_data"=w187:i64[])  [unwired: 8 in]
                  n61 = To Unsigned Word Integer(number=w187) -> (unsigned 16bit integer=w186:u16[])
                  n62 = Select(t=w186, s=w189, f=w188) -> (s? t:f=w185:u16[])
                }
              }
              n63 = Select(t=myRIO_BRig_RT__Case_NonExp_stateList."UploadSettings_dataLC_1", s=w174, f=myRIO_BRig_RT__Case_NonExp_stateList."UploadSettings_Read_dataMTrig" ("t")) -> (s? t:f=w169:T1)
            }
            frame "UploadSettings_Read_dataMTrig" {
              # "grab dataMTrig and\nstore it in the\ngeneric data array"
              # "dataMTrig"
              n64 = call "myRIO_BRig_RT_dataMTrig_init_details.vi"() -> ("output_dataSize"=w198:i32, "output_dataName"=w201:string)  [unwired: 10 in]
              n65 = call "myRIO_BRig_RT_comm_webdav_uploadReceived_check.vi"("input_dataName"=w201) -> ("output_Iexist"=w200:bool, "output_dataPath"=w199:path)  [unwired: 9 in]
              n66 = case shown="True" w200 {
                tunnel: w199 -> [_ w214]
                tunnel: w198 -> [_ w213]
                tunnel: [_ w212] -> w197
                tunnel: w194 -> [w207 w211]
                tunnel: [w207 w208] -> w193
                frame False {
                }
                frame True {
                  n67 = call "myRIO_BRig_RT_comm_webdav_uploadReceived_read.vi"("input_dataSize"=w213, "input_filePath"=w214) -> ("output_Ivalid"=w212:bool, "output_data"=w210:i64[])  [unwired: 8 in]
                  n68 = To Unsigned Word Integer(number=w210) -> (unsigned 16bit integer=w209:u16[])
                  n69 = Select(t=w209, s=w212, f=w211) -> (s? t:f=w208:u16[])
                }
              }
              n70 = Select(t=myRIO_BRig_RT__Case_NonExp_stateList."UploadSettings_dataMTrig_1", s=w197, f=myRIO_BRig_RT__Case_NonExp_stateList."Idle" ("t")) -> (s? t:f=w192:T1)
            }
            frame "UploadSettings_dataExp_1" {
              w223 = 100.0 ("y")
              w241 = u16 1000 ("y")
              # "Freq"
              # "f_millisec2count"
              # "laser"
              # "Cue_max"
              # "Cue_min"
              # "CuePenalty"
              # "Timeout"
              # "Wrong"
              # "Selection"
              # "RewardPost"
              # "Reward_R"
              # "Reward_L"
              # "Tcycle"
              # "TPB_min_R"
              # "TPB_min_L"
              # "TPB_max_R"
              # "TPB_max_L"
              # "I_trialUntilReward"
              # "ENL_penalty"
              # "ENL_min"
              # "ENL_max"
              # "BUR_max"
              # "BUR_min"
              # "CueCycles"
              # "Audio_Freq_R"
              # "Audio_Freq_L"
              # "Audio_Amp_R"
              # "Audio_Amp_L"
              n71 = call "myRIO_BRig_RT_dataExp_laser_f_millisec2count.vi"() -> ("output_laser_f_millisec2count"=w237:i32)  [unwired: 11 in]
              n72 = call "myRIO_BRig_RT_dataExp_laser_Freq.vi"() -> ("output_laser_Freq"=w236:i32)  [unwired: 11 in]
              n73 = call "myRIO_BRig_RT_dataExp_CueCycles.vi"() -> ("output_CueCycles"=w284:i32)  [unwired: 11 in]
              n74 = call "myRIO_BRig_RT_dataExp_Audio_amp__R.vi"() -> ("output_Audio_amp__R"=w288:i32)  [unwired: 11 in]
              n75 = call "myRIO_BRig_RT_dataExp_Audio_amp__L.vi"() -> ("output_Audio_amp__L"=w290:i32)  [unwired: 11 in]
              n76 = call "myRIO_BRig_RT_dataExp_Tcycle_Reward__L.vi"() -> ("output_Tcycle_Reward__L"=w261:i32)  [unwired: 11 in]
              n77 = call "myRIO_BRig_RT_dataExp_Tcycle_Reward__R.vi"() -> ("output_Tcycle_Reward__R"=w260:i32)  [unwired: 11 in]
              n78 = call "myRIO_BRig_RT_dataExp_Tcycle_RewardPost.vi"() -> ("output_Tcycle_RewardPost"=w259:i32)  [unwired: 11 in]
              n79 = call "myRIO_BRig_RT_dataExp_BUR_min.vi"() -> ("output_BUR_min"=w281:i32)  [unwired: 11 in]
              n80 = call "myRIO_BRig_RT_dataExp_ENL_min.vi"() -> ("output_ENL_min"=w277:i32)  [unwired: 11 in]
              n81 = call "myRIO_BRig_RT_dataExp_TPB_max__L.vi"() -> ("output_TPB_max__L"=w269:i32)  [unwired: 11 in]
              n82 = call "myRIO_BRig_RT_dataExp_TPB_max__R.vi"() -> ("output_TPB_max__R"=w268:i32)  [unwired: 11 in]
              n83 = call "myRIO_BRig_RT_dataExp_ENL_penalty.vi"() -> ("output_ENL_penalty"=w276:i32)  [unwired: 11 in]
              n84 = call "myRIO_BRig_RT_dataExp_laser_Power.vi"() -> ("output_laser_Power"=w235:i32)  [unwired: 11 in]
              n85 = call "myRIO_BRig_RT_dataExp_laser_Tpeak.vi"() -> ("output_laser_Tpeak"=w234:i32)  [unwired: 11 in]
              n86 = call "myRIO_BRig_RT_dataExp_Audio_freq__L.vi"() -> ("output_Audio_freq__L"=w286:i32)  [unwired: 11 in]
              n87 = call "myRIO_BRig_RT_dataExp_Audio_freq__R.vi"() -> ("output_Audio_freq__R"=w285:i32)  [unwired: 11 in]
              n88 = call "myRIO_BRig_RT_dataExp_BUR_max.vi"() -> ("output_BUR_max"=w282:i32)  [unwired: 11 in]
              n89 = call "myRIO_BRig_RT_dataExp_ENL_max.vi"() -> ("output_ENL_max"=w278:i32)  [unwired: 11 in]
              n90 = call "myRIO_BRig_RT_dataExp_ItrialUntilReward.vi"() -> ("output_I_trialUntilReward"=w272:i32)  [unwired: 11 in]
              n91 = call "myRIO_BRig_RT_dataExp_Tcycle_Selection.vi"() -> ("output_Tcycle_Selection"=w258:i32)  [unwired: 11 in]
              n92 = call "myRIO_BRig_RT_dataExp_Tcycle_Wrong.vi"() -> ("output_Tcycle_Wrong"=w257:i32)  [unwired: 11 in]
              n93 = call "myRIO_BRig_RT_dataExp_Tcycle_Timeout.vi"() -> ("output_Tcycle_Timeout"=w256:i32)  [unwired: 11 in]
              n94 = call "myRIO_BRig_RT_dataExp_TPB_min__L.vi"() -> ("output_TPB_min__L"=w267:i32)  [unwired: 11 in]
              n95 = call "myRIO_BRig_RT_dataExp_TPB_min__R.vi"() -> ("output_TPB_min__R"=w266:i32)  [unwired: 11 in]
              n96 = call "myRIO_BRig_RT_dataExp_laser_Tshutter.vi"() -> ("output_laser_Tshutter"=w233:i32)  [unwired: 11 in]
              n97 = call "myRIO_BRig_RT_dataExp_laser_duration.vi"() -> ("output_laser_duration"=w232:i32)  [unwired: 11 in]
              n98 = call "myRIO_BRig_RT_dataExp_Tcycle_CuePenalty.vi"() -> ("output_Tcycle_CuePenalty"=w249:i32)  [unwired: 11 in]
              n99 = call "myRIO_BRig_RT_dataExp_Tcycle_Cue_min.vi"() -> ("output_Tcycle_Cue_min"=w248:i32)  [unwired: 11 in]
              n100 = call "myRIO_BRig_RT_dataExp_Tcycle_Cue_max.vi"() -> ("output_Tcycle_Cue_max"=w247:i32)  [unwired: 11 in]
              n101 = Index Array(array=w240, index #1=w290, index #2=w288, index #3=w286, index #4=w285, index #5=w284, index #6=w282, index #7=w281, index #8=w278, index #9=w277, index #10=w276, index #11=w272, index #12=w269, index #13=w268, index #14=w267, index #15=w266, index #16=w261, index #17=w260, index #18=w259, index #19=w258, index #20=w257, index #21=w256, index #22=w249, index #23=w248, index #24=w247, index #25=w237, index #26=w236, index #27=w235, index #28=w234, index #29=w233, index #30=w232) -> (element #1=w289:u16, element #2=w287:u16, element #3=w244:u16, element #4=w243:u16, element #5=w283:u16, element #6=w280:u16, element #7=w279:u16, element #8=w275:u16, element #9=w274:u16, element #10=w273:u16, element #11=w270:u16, element #12=w265:u16, element #13=w264:u16, element #14=w263:u16, element #15=w262:u16, element #16=w255:u16, element #17=w254:u16, element #18=w253:u16, element #19=w252:u16, element #20=w251:u16, element #21=w250:u16, element #22=w246:u16, element #23=w239:u16, element #24=w238:u16, element #25=w231:u16, element #26=w222:u16, element #27=w221:u16, element #28=w220:u16, element #29=w219:u16, element #30=w215:u16)
              n102 = To Double Precision Float(number=w231) -> (double precision float=w230:dbl)
              n103 = To Double Precision Float(number=w222) -> (double precision float=w228:dbl)
              n104 = To Double Precision Float(number=w221) -> (double precision float=w226:dbl)
              n105 = To Double Precision Float(number=w220) -> (double precision float=w225:dbl)
              n106 = To Double Precision Float(number=w219) -> (double precision float=w224:dbl)
              n107 = local write "Tcycle_Selection"(w252) -> ()
              n108 = local write "Tcycle_Wrong"(w251) -> ()
              n109 = local write "Tcycle_Timeout"(w250) -> ()
              n110 = local write "Audio_Amp__L"(w289) -> ()
              n111 = local write "Audio_Amp__R"(w287) -> ()
              n112 = Divide(x=w230, y=w223) -> (x/y=w229:dbl)
              n113 = Divide(x=w228, y=w223) -> (x/y=w227:dbl)
              n114 = Divide(x=w226, y=w223) -> (x/y=w218:dbl)
              n115 = Divide(x=w225, y=w223) -> (x/y=w217:dbl)
              n116 = Divide(x=w224, y=w223) -> (x/y=w216:dbl)
              n117 = local write "Tcycle_ENLPenalty"(w273) -> ()
              n118 = local write "Tcycle_ENL_max"(w275) -> ()
              n119 = local write "laser_duration"(w215) -> ()
              n120 = local write "TpB_Min_L"(w263) -> ()
              n121 = local write "TpB_Min_R"(w262) -> ()
              n122 = local write "laser_power"(w218) -> ()
              n123 = local write "f_millisec2count"(w229) -> ()
              n124 = local write "laser_Tshutter"(w216) -> ()
              n125 = local write "laser_Tpeak"(w217) -> ()
              n126 = local write "laser_Freq"(w227) -> ()
              n127 = local write "Tcycle_CuePenalty"(w246) -> ()
              n128 = local write "Tcycle_Cue_min"(w239) -> ()
              n129 = local write "Tcycle_Cue_max"(w238) -> ()
              n130 = Quotient & Remainder(x=w244, y=w241) -> (floor(x/y)=w245:u16)  [unwired: 1 out]
              n131 = Quotient & Remainder(x=w243, y=w241) -> (floor(x/y)=w242:u16)  [unwired: 1 out]
              n132 = Not Equal To 0?(x=w270) -> (x != 0?=w271:bool)
              n133 = local write "Tcycle_Reward_L"(w255) -> ()
              n134 = local write "Tcycle_Reward_R"(w254) -> ()
              n135 = local write "Tcycle_RewardPost"(w253) -> ()
              n136 = local write "CueCycles"(w283) -> ()
              n137 = local write "BUR_min"(w279) -> ()
              n138 = local write "BUR_max"(w280) -> ()
              n139 = local write "Tcycle_ENL_min"(w274) -> ()
              n140 = local write "TpB_Max_L"(w265) -> ()
              n141 = local write "TpB_Max_R"(w264) -> ()
              n142 = local write "TrialUntilReward"(w271) -> ()
              n143 = local write "Audio_Freq__L"(w245) -> ()
              n144 = local write "Audio_Freq__R"(w242) -> ()
            }
            frame "UploadSettings_dataLC_1" {
              # "Cue1_All_delayOpt"
              # "ENL1_All_delayOpt"
              # "Cue1_First_delayOpt"
              # "ENL1_First_delayOpt"
              # "ENL1 First"
              # "Cue1 All"
              # "Cue1 First"
              # "Count"
              # "Tdelay"
              # "Prob"
              # "OnOff"
              # "Block"
              # "ENL1 All"
              # "Count"
              # "Tdelay"
              # "Prob"
              # "OnOff"
              # "Block"
              # "Count"
              # "Tdelay"
              # "Prob"
              # "Block"
              # "OnOff"
              # "Count"
              # "Tdelay"
              # "Prob"
              # "OnOff"
              # "Block"
              n145 = call "myRIO_BRig_RT_dataLC_Cue1_First_Block.vi"() -> ("output_Cue1_First_Block"=w353:i32)  [unwired: 11 in]
              n146 = call "myRIO_BRig_RT_dataLC_Cue1_First_OnOff.vi"() -> ("output_Cue1_First_OnOff"=w351:i32)  [unwired: 11 in]
              n147 = call "myRIO_BRig_RT_dataLC_Cue1_First_Count.vi"() -> ("output_Cue1_First_Count"=w348:i32)  [unwired: 11 in]
              n148 = call "myRIO_BRig_RT_dataLC_Cue1_All_Block.vi"() -> ("output_Cue1_All_Block"=w335:i32)  [unwired: 11 in]
              n149 = call "myRIO_BRig_RT_dataLC_Cue1_All_OnOff.vi"() -> ("output_Cue1_All_OnOff"=w334:i32)  [unwired: 11 in]
              n150 = call "myRIO_BRig_RT_dataLC_Cue1_All_Count.vi"() -> ("output_Cue1_All_Count"=w345:i32)  [unwired: 11 in]
              n151 = call "myRIO_BRig_RT_dataLC_ENL1_First_Block.vi"() -> ("output_ENL1_First_Block"=w333:i32)  [unwired: 11 in]
              n152 = call "myRIO_BRig_RT_dataLC_ENL1_First_OnOff.vi"() -> ("output_ENL1_First_OnOff"=w344:i32)  [unwired: 11 in]
              n153 = call "myRIO_BRig_RT_dataLC_ENL1_First_Count.vi"() -> ("output_ENL1_First_Count"=w341:i32)  [unwired: 11 in]
              n154 = call "myRIO_BRig_RT_dataLC_ENL1_All_Block.vi"() -> ("output_ENL1_All_Block"=w340:i32)  [unwired: 11 in]
              n155 = call "myRIO_BRig_RT_dataLC_ENL1_All_OnOff.vi"() -> ("output_ENL1_All_OnOff"=w339:i32)  [unwired: 11 in]
              n156 = call "myRIO_BRig_RT_dataLC_ENL1_All_Count.vi"() -> ("output_ENL1_All_Count"=w336:i32)  [unwired: 11 in]
              n157 = call "myRIO_BRig_RT_dataLC_ENL1_First_delayOpt.vi"() -> ("output_ENL1_First_delayOpt"=w310:i32)  [unwired: 11 in]
              n158 = call "myRIO_BRig_RT_dataLC_Cue1_First_delayOpt.vi"() -> ("output_Cue1_First_delayOpt"=w309:i32)  [unwired: 11 in]
              n159 = call "myRIO_BRig_RT_dataLC_ENL1_All_delayOpt.vi"() -> ("output_ENL1_All_delayOpt"=w302:i32)  [unwired: 11 in]
              n160 = call "myRIO_BRig_RT_dataLC_Cue1_All_delayOpt.vi"() -> ("output_Cue1_All_delayOpt"=w301:i32)  [unwired: 11 in]
              n161 = call "myRIO_BRig_RT_dataLC_Cue1_First_Probability.vi"() -> ("output_Cue1_First_Probability"=w350:i32)  [unwired: 11 in]
              n162 = call "myRIO_BRig_RT_dataLC_Cue1_First_Tdelay.vi"() -> ("output_Cue1_First_Tdelay"=w349:i32)  [unwired: 11 in]
              n163 = call "myRIO_BRig_RT_dataLC_Cue1_All_Probability.vi"() -> ("output_Cue1_All_Probability"=w347:i32)  [unwired: 11 in]
              n164 = call "myRIO_BRig_RT_dataLC_Cue1_All_Tdelay.vi"() -> ("output_Cue1_All_Tdelay"=w346:i32)  [unwired: 11 in]
              n165 = call "myRIO_BRig_RT_dataLC_ENL1_First_Probability.vi"() -> ("output_ENL1_First_Probability"=w343:i32)  [unwired: 11 in]
              n166 = call "myRIO_BRig_RT_dataLC_ENL1_First_Tdelay.vi"() -> ("output_ENL1_First_Tdelay"=w342:i32)  [unwired: 11 in]
              n167 = call "myRIO_BRig_RT_dataLC_ENL1_All_Probability.vi"() -> ("output_ENL1_All_Probability"=w338:i32)  [unwired: 11 in]
              n168 = call "myRIO_BRig_RT_dataLC_ENL1_All_Tdelay.vi"() -> ("output_ENL1_All_Tdelay"=w337:i32)  [unwired: 11 in]
              n169 = Index Array(array=w311, index #1=w353, index #2=w351, index #3=w350, index #4=w349, index #5=w348, index #6=w335, index #7=w334, index #8=w347, index #9=w346, index #10=w345, index #11=w333, index #12=w344, index #13=w343, index #14=w342, index #15=w341, index #16=w340, index #17=w339, index #18=w338, index #19=w337, index #20=w336, index #21=w310, index #22=w309, index #23=w302, index #24=w301) -> (element #1=w352:u16, element #2=w331:u16, element #3=w330:u16, element #4=w329:u16, element #5=w328:u16, element #6=w324:u16, element #7=w323:u16, element #8=w322:u16, element #9=w321:u16, element #10=w320:u16, element #11=w319:u16, element #12=w318:u16, element #13=w317:u16, element #14=w316:u16, element #15=w303:u16, element #16=w315:u16, element #17=w314:u16, element #18=w313:u16, element #19=w312:u16, element #20=w304:u16, element #21=w307:u16, element #22=w305:u16, element #23=w298:u16, element #24=w297:u16)
              n170 = Not Equal To 0?(x=w298) -> (x != 0?=w300:bool)
              n171 = Not Equal To 0?(x=w297) -> (x != 0?=w299:bool)
              n172 = Not Equal To 0?(x=w307) -> (x != 0?=w308:bool)
              n173 = Not Equal To 0?(x=w305) -> (x != 0?=w306:bool)
              n174 = Not Equal To 0?(x=w331) -> (x != 0?=w332:bool)
              n175 = Not Equal To 0?(x=w323) -> (x != 0?=w327:bool)
              n176 = Not Equal To 0?(x=w318) -> (x != 0?=w326:bool)
              n177 = Not Equal To 0?(x=w314) -> (x != 0?=w325:bool)
              n178 = local write "LC_Cue1_First_Probability"(w330) -> ()
              n179 = local write "LC_ENL1_First_Probability"(w317) -> ()
              n180 = local write "LC_ENL1_First_delayOpt"(w308) -> ()
              n181 = local write "LC_Cue1_First_delayOpt"(w306) -> ()
              n182 = local write "LC_ENL1_All_delayOpt"(w300) -> ()
              n183 = local write "LC_Cue1_All_delayOpt"(w299) -> ()
              n184 = local write "LC_Cue1_All_Probability"(w322) -> ()
              n185 = local write "LC_Cue1_First_Tdelay"(w329) -> ()
              n186 = local write "LC_ENL1_All_Probability"(w313) -> ()
              n187 = local write "LC_Cue1_First_OnOff"(w332) -> ()
              n188 = local write "LC_Cue1_First_Count"(w328) -> ()
              n189 = local write "LC_Cue1_First_Block"(w352) -> ()
              n190 = local write "LC_ENL1_First_Tdelay"(w316) -> ()
              n191 = local write "LC_ENL1_First_OnOff"(w326) -> ()
              n192 = local write "LC_ENL1_First_Count"(w303) -> ()
              n193 = local write "LC_ENL1_First_Block"(w319) -> ()
              n194 = local write "LC_Cue1_All_Tdelay"(w321) -> ()
              n195 = local write "LC_Cue1_All_OnOff"(w327) -> ()
              n196 = local write "LC_Cue1_All_Count"(w320) -> ()
              n197 = local write "LC_Cue1_All_Block"(w324) -> ()
              n198 = local write "LC_ENL1_All_Tdelay"(w312) -> ()
              n199 = local write "LC_ENL1_All_OnOff"(w325) -> ()
              n200 = local write "LC_ENL1_All_Count"(w304) -> ()
              n201 = local write "LC_ENL1_All_Block"(w315) -> ()
            }
            frame "UploadSettings_dataLC_2" {
              # "Wrong"
              # "Reward"
              # "Trial"
              # "Tdelay"
              # "Prob"
              # "Block"
              # "OnOff"
              # "Trial"
              # "Tdelay"
              # "Prob"
              # "OnOff"
              # "Block"
              n202 = call "myRIO_BRig_RT_dataLC_Reward_Block.vi"() -> ("output_Reward_Block"=w386:i32)  [unwired: 11 in]
              n203 = call "myRIO_BRig_RT_dataLC_Reward_OnOff.vi"() -> ("output_Reward_OnOff"=w384:i32)  [unwired: 11 in]
              n204 = call "myRIO_BRig_RT_dataLC_Reward_Trial.vi"() -> ("output_Reward_Trial"=w381:i32)  [unwired: 11 in]
              n205 = call "myRIO_BRig_RT_dataLC_Wrong_Block.vi"() -> ("output_Wrong_Block"=w377:i32)  [unwired: 11 in]
              n206 = call "myRIO_BRig_RT_dataLC_Wrong_OnOff.vi"() -> ("output_Wrong_OnOff"=w376:i32)  [unwired: 11 in]
              n207 = call "myRIO_BRig_RT_dataLC_Wrong_Trial.vi"() -> ("output_Wrong_Trial"=w378:i32)  [unwired: 11 in]
              n208 = call "myRIO_BRig_RT_dataLC_Reward_Probability.vi"() -> ("output_Reward_Probability"=w383:i32)  [unwired: 11 in]
              n209 = call "myRIO_BRig_RT_dataLC_Reward_Tdelay.vi"() -> ("output_Reward_Tdelay"=w382:i32)  [unwired: 11 in]
              n210 = call "myRIO_BRig_RT_dataLC_Wrong_Probability.vi"() -> ("output_Wrong_Probability"=w380:i32)  [unwired: 11 in]
              n211 = call "myRIO_BRig_RT_dataLC_Wrong_Tdelay.vi"() -> ("output_Wrong_Tdelay"=w379:i32)  [unwired: 11 in]
              n212 = Index Array(array=w360, index #1=w386, index #2=w384, index #3=w383, index #4=w382, index #5=w381, index #6=w377, index #7=w376, index #8=w380, index #9=w379, index #10=w378) -> (element #1=w385:u16, element #2=w374:u16, element #3=w373:u16, element #4=w372:u16, element #5=w371:u16, element #6=w369:u16, element #7=w368:u16, element #8=w367:u16, element #9=w366:u16, element #10=w365:u16)
              n213 = Not Equal To 0?(x=w374) -> (x != 0?=w375:bool)
              n214 = Not Equal To 0?(x=w368) -> (x != 0?=w370:bool)
              n215 = local write "LC_Reward_Probability"(w373) -> ()
              n216 = local write "LC_Wrong_Probability"(w367) -> ()
              n217 = local write "LC_Reward_Tdelay"(w372) -> ()
              n218 = local write "LC_Reward_OnOff"(w375) -> ()
              n219 = local write "LC_Reward_Block"(w385) -> ()
              n220 = local write "LC_Reward_Trial"(w371) -> ()
              n221 = local write "LC_Wrong_Tdelay"(w366) -> ()
              n222 = local write "LC_Wrong_OnOff"(w370) -> ()
              n223 = local write "LC_Wrong_Block"(w369) -> ()
              n224 = local write "LC_Wrong_Trial"(w365) -> ()
            }
            frame "UploadSettings_dataMTrig_1" {
              # "Tdelay_R"
              # "Tdelay_L"
              # "Tcycle_R"
              # "Tcycle_L"
              # "RewCalib_nCycle_R"
              # "RewCalib_nCycle_L"
              # "Solenoid"
              # "Laser_Tcycle"
              n225 = call "myRIO_BRig_RT_dataMTrig_Laser_Tcycle.vi"() -> ("output_Laser_Tcycle"=w396:i32)  [unwired: 11 in]
              n226 = call "myRIO_BRig_RT_dataMTrig_Solenoid_RewCalib_nCycle__L.vi"() -> ("output_Solenoid_RewCalib_nCycle__L"=w395:i32)  [unwired: 11 in]
              n227 = call "myRIO_BRig_RT_dataMTrig_Solenoid_RewCalib_nCycle__R.vi"() -> ("output_Solenoid_RewCalib_nCycle__R"=w394:i32)  [unwired: 11 in]
              n228 = call "myRIO_BRig_RT_dataMTrig_Solenoid_Tdelay__L.vi"() -> ("output_Solenoid_Tdelay__L"=w391:i32)  [unwired: 11 in]
              n229 = call "myRIO_BRig_RT_dataMTrig_Solenoid_Tdelay__R.vi"() -> ("output_Solenoid_Tdelay__R"=w390:i32)  [unwired: 11 in]
              n230 = call "myRIO_BRig_RT_dataMTrig_Solenoid_Tcycle__L.vi"() -> ("output_Solenoid_Tcycle__L"=w393:i32)  [unwired: 11 in]
              n231 = call "myRIO_BRig_RT_dataMTrig_Solenoid_Tcycle__R.vi"() -> ("output_Solenoid_Tcycle__R"=w392:i32)  [unwired: 11 in]
              n232 = Index Array(array=w389, index #1=w396, index #2=w395, index #3=w394, index #4=w393, index #5=w392, index #6=w391, index #7=w390) -> (element #1=w403:u16, element #2=w402:u16, element #3=w401:u16, element #4=w400:u16, element #5=w399:u16, element #6=w398:u16, element #7=w397:u16)
              n233 = Replace Array Subset(array=w409, new element #1=w403, index #1=w396, new element #2=w402, index #2=w395, new element #3=w401, index #3=w394, new element #4=w400, index #4=w393, new element #5=w399, index #5=w392, new element #6=w398, index #6=w391, new element #7=w397, index #7=w390) -> (w408:u16[])
              n234 = local write "MTrig_Solenoid_Tcycle__L"(w400) -> ()
              n235 = local write "MTrig_Solenoid_Tcycle__R"(w399) -> ()
              n236 = local write "MTrig_Laser_Tcycle"(w403) -> ()
            }
            frame "Idle" {
              w429 = u16 1000 ("y")
              # "To ensure timing, we split the\nidle state into 4 phases"
              # "Laser_Tcycle"
              # "Audio_Tcycle_R"
              # "Audio_Tcycle_L"
              n237 = local read "MTrig_Audio_trig__L"() -> (w418:bool)
              n238 = local read "MTrig_Audio_trig__R"() -> (w420:bool)
              n239 = Select(t=myRIO_BRig_RT__Case_NonExp_stateList."SendData" ("Enum"), s="SendData", f=myRIO_BRig_RT__Case_NonExp_stateList."Idle_2" ("Enum")) -> (s? t:f=w413:T1)
              n240 = local read "MTrig_Laser_trig"() -> (w419:bool)
              n241 = call "myRIO_BRig_RT_dataMTrig_Audio_Tcycle__L.vi"() -> ("output_Audio_Tcycle__L"=w436:i32)  [unwired: 11 in]
              n242 = call "myRIO_BRig_RT_dataMTrig_Audio_Tcycle__R.vi"() -> ("output_Audio_Tcycle__R"=w435:i32)  [unwired: 11 in]
              n243 = call "myRIO_BRig_RT_dataMTrig_Laser_Tcycle.vi"() -> ("output_Laser_Tcycle"=w434:i32)  [unwired: 11 in]
              n244 = local read "MTrig_Laser_Tcycle"() -> (w411:u16)
              n245 = Select(t=myRIO_BRig_RT__Case_NonExp_stateList."TestConnection" ("Enum"), s="TestConnection", f=w413) -> (s? t:f=w422:T1)
              n246 = local read "Tcycle_Cue_min"() -> (w412:u16)
              n247 = Compound Arithmetic op=OR(w418, w420, w419) -> (w421:bool)
              n248 = case shown="True" w421 {
                frame False {
                }
                frame True {
                  w437 = FALSE
                  n249 = local write "MTrig_Audio_trig__L"(w437) -> ()
                  n250 = local write "MTrig_Audio_trig__R"(w437) -> ()
                  n251 = local write "MTrig_Laser_trig"(w437) -> ()
                }
              }
              n252 = Replace Array Subset(array=w432, new element #1=w412, index #1=w436, new element #2=w412, index #2=w435, new element #3=w411, index #3=w434) -> (w433:u16[])
              n253 = local read "Audio_Amp__R"() -> (w425:u16)
              n254 = local read "Audio_Amp__L"() -> (w426:u16)
              n255 = local read "Audio_Freq__R"() -> (w423:u16)
              n256 = local read "Audio_Freq__L"() -> (w424:u16)
              n257 = Multiply(x=w423, y=w429) -> (x*y=w427:u16)
              n258 = Multiply(x=w424, y=w429) -> (x*y=w428:u16)
            }
            frame "Idle_2" {
              # "To ensure timing, we split the\nidle state into 4 phases"
              # "Ncycles"
              # "Ncycles"
              # "RewCalib"
              # "RewCalib"
              # "Solenoid R"
              # "Solenoid L"
              n259 = call "myRIO_BRig_RT_dataMTrig_Solenoid_RewCalib_OnOff__L.vi"() -> ("output_Solenoid_RewCalib_OnOff__L"=w467:i32)  [unwired: 11 in]
              n260 = call "myRIO_BRig_RT_dataMTrig_Solenoid_N__L.vi"() -> ("output_Solenoid_N__L"=w455:i32)  [unwired: 11 in]
              n261 = call "myRIO_BRig_RT_dataMTrig_Solenoid_RewCalib_OnOff__R.vi"() -> ("output_Solenoid_RewCalib_OnOff__R"=w452:i32)  [unwired: 11 in]
              n262 = call "myRIO_BRig_RT_dataMTrig_Solenoid_N__R.vi"() -> ("output_Solenoid_N__R"=w451:i32)  [unwired: 11 in]
              n263 = Index Array(array=w458, index #1=w467, index #2=w455, index #3=w452, index #4=w451) -> (element #1=w454:u16, element #2=w449:u16, element #3=w450:u16, element #4=w448:u16)
              n264 = local read "RewCalib_Trig_L"() -> (w447:bool)
              n265 = local read "RewCalib_Trig_R"() -> (w446:bool)
              n266 = Equal To 0?(x=w449) -> (x = 0?=w457:bool)
              n267 = Equal To 0?(x=w448) -> (x = 0?=w456:bool)
              n268 = Not Equal To 0?(x=w450) -> (x != 0?=w468:bool)
              n269 = Not Equal To 0?(x=w454) -> (x != 0?=w469:bool)
              n270 = And(x=w457, y=w456) -> (x .and. y?=w461:bool)
              n271 = Or(x=w447, y=w446) -> (x .or. y?=w462:bool)
              n272 = Not Exclusive Or(1:w469, 2:w447) -> (0:w464:bool)
              n273 = Not Exclusive Or(1:w468, 2:w446) -> (0:w466:bool)
              n274 = And(x=w462, y=w461) -> (x .and. y?=w444:bool)
              n275 = Not(x=w464) -> (.not. x?=w463:bool)
              n276 = Not(x=w466) -> (.not. x?=w465:bool)
              n277 = Or(x=w463, y=w465) -> (x .or. y?=w445:bool)
              n278 = Or(x=w444, y=w445) -> (x .or. y?=w460:bool)
              n279 = Select(t=myRIO_BRig_RT__Case_NonExp_stateList."RewardCalibration_pre" ("Enum"), s=w460, f=myRIO_BRig_RT__Case_NonExp_stateList."Idle_3" ("Enum")) -> (s? t:f=w443:T1)
            }
            frame "Idle_3" {
              w492 = u8 0 ("f")
              # "To ensure timing, we split the\nidle state into 4 phases"
              n280 = local read "MTrig_Solenoid_trig__L"() -> (w478:bool)
              n281 = local read "MTrig_Solenoid_trig__R"() -> (w493:bool)
              n282 = local read "warmupType"() -> (w484:bool)
              n283 = local read "warmup"() -> (w485:bool)
              n284 = Not(x=w484) -> (.not. x?=w486:bool)
              n285 = Select(t=u8 1, s=w478, f=w492) -> (s? t:f=w491:u8)
              n286 = Select(t=u8 2, s=w493, f=w492) -> (s? t:f=w490:u8)
              n287 = And(x=w485, y=w486) -> (x .and. y?=w483:bool)
              n288 = And(x=w485, y=w484) -> (x .and. y?=w473:bool)
              n289 = Add(x=w491, y=w490) -> (x+y=w489:u8)
              n290 = case shown="3" w489 {
                tunnel: w488 -> [w496 w500 w518 w536]
                tunnel: [w496 w499 w517 w535] -> w487
                tunnel: w483 -> [_ w498 w516 w534]
                tunnel: [_ TRUE TRUE TRUE] -> w475
                frame 0, Default {
                }
                frame 1 {
                  n291 = case shown="True" w498 {
                    tunnel: w500 -> [w509 w514]
                    tunnel: [w508 w513] -> w499
                    frame True {
                      # "Audio_L"
                      # "Solenoid_L"
                      n292 = call "myRIO_BRig_RT_dataMTrig_Solenoid_N__L.vi"() -> ("output_Solenoid_N__L"=w505:i32)  [unwired: 11 in]
                      n293 = call "myRIO_BRig_RT_dataMTrig_Audio_N__L.vi"() -> ("output_Audio_N__L"=w503:i32)  [unwired: 11 in]
                      n294 = Index Array(array=w509, index #1=w505, index #2=w503) -> (element #1=w507:u16, element #2=w506:u16)
                      n295 = Increment(x=w507) -> (x+1=w504:u16)
                      n296 = Increment(x=w506) -> (x+1=w502:u16)
                      n297 = Replace Array Subset(array=w509, new element #1=w504, index #1=w505, new element #2=w502, index #2=w503) -> (w508:u16[])
                    }
                    frame False {
                      # "Solenoid_L"
                      n298 = call "myRIO_BRig_RT_dataMTrig_Solenoid_N__L.vi"() -> ("output_Solenoid_N__L"=w511:i32)  [unwired: 11 in]
                      n299 = Index Array(array=w514, index=w511) -> (element=w512:u16)
                      n300 = Increment(x=w512) -> (x+1=w510:u16)
                      n301 = Replace Array Subset(array=w514, new element=w510, index=w511) -> (w513:u16[])
                    }
                  }
                  n302 = local write "MTrig_Solenoid_trig__L"(FALSE) -> ()
                }
                frame 2 {
                  n303 = case shown="True" w516 {
                    tunnel: w518 -> [w527 w532]
                    tunnel: [w526 w531] -> w517
                    frame True {
                      # "Audio_R"
                      # "Solenoid_R"
                      n304 = call "myRIO_BRig_RT_dataMTrig_Solenoid_N__R.vi"() -> ("output_Solenoid_N__R"=w523:i32)  [unwired: 11 in]
                      n305 = call "myRIO_BRig_RT_dataMTrig_Audio_N__R.vi"() -> ("output_Audio_N__R"=w522:i32)  [unwired: 11 in]
                      n306 = Index Array(array=w527, index #1=w523, index #2=w522) -> (element #1=w525:u16, element #2=w524:u16)
                      n307 = Increment(x=w524) -> (x+1=w520:u16)
                      n308 = Increment(x=w525) -> (x+1=w521:u16)
                      n309 = Replace Array Subset(array=w527, new element #1=w521, index #1=w523, new element #2=w520, index #2=w522) -> (w526:u16[])
                    }
                    frame False {
                      # "Solenoid_R"
                      n310 = call "myRIO_BRig_RT_dataMTrig_Solenoid_N__R.vi"() -> ("output_Solenoid_N__R"=w528:i32)  [unwired: 11 in]
                      n311 = Index Array(array=w532, index=w528) -> (element=w530:u16)
                      n312 = Increment(x=w530) -> (x+1=w529:u16)
                      n313 = Replace Array Subset(array=w532, new element=w529, index=w528) -> (w531:u16[])
                    }
                  }
                  n314 = local write "MTrig_Solenoid_trig__R"(FALSE) -> ()
                }
                frame 3 {
                  w537 = FALSE
                  n315 = case shown="True" w534 {
                    tunnel: w536 -> [w551 w559]
                    tunnel: [w550 w558] -> w535
                    frame True {
                      # "Audio_R"
                      # "Solenoid_R"
                      # "Audio_L"
                      # "Solenoid_L"
                      n316 = call "myRIO_BRig_RT_dataMTrig_Solenoid_N__L.vi"() -> ("output_Solenoid_N__L"=w545:i32)  [unwired: 11 in]
                      n317 = call "myRIO_BRig_RT_dataMTrig_Audio_N__L.vi"() -> ("output_Audio_N__L"=w543:i32)  [unwired: 11 in]
                      n318 = call "myRIO_BRig_RT_dataMTrig_Solenoid_N__R.vi"() -> ("output_Solenoid_N__R"=w541:i32)  [unwired: 11 in]
                      n319 = call "myRIO_BRig_RT_dataMTrig_Audio_N__R.vi"() -> ("output_Audio_N__R"=w540:i32)  [unwired: 11 in]
                      n320 = Index Array(array=w551, index #1=w545, index #2=w543, index #3=w541, index #4=w540) -> (element #1=w549:u16, element #2=w548:u16, element #3=w547:u16, element #4=w546:u16)
                      n321 = Increment(x=w546) -> (x+1=w538:u16)
                      n322 = Increment(x=w549) -> (x+1=w544:u16)
                      n323 = Increment(x=w548) -> (x+1=w542:u16)
                      n324 = Increment(x=w547) -> (x+1=w539:u16)
                      n325 = Replace Array Subset(array=w551, new element #1=w544, index #1=w545, new element #2=w542, index #2=w543, new element #3=w539, index #3=w541, new element #4=w538, index #4=w540) -> (w550:u16[])
                    }
                    frame False {
                      # "Solenoid_R"
                      # "Solenoid_L"
                      n326 = call "myRIO_BRig_RT_dataMTrig_Solenoid_N__L.vi"() -> ("output_Solenoid_N__L"=w555:i32)  [unwired: 11 in]
                      n327 = call "myRIO_BRig_RT_dataMTrig_Solenoid_N__R.vi"() -> ("output_Solenoid_N__R"=w552:i32)  [unwired: 11 in]
                      n328 = Index Array(array=w559, index #1=w555, index #2=w552) -> (element #1=w557:u16, element #2=w556:u16)
                      n329 = Increment(x=w557) -> (x+1=w554:u16)
                      n330 = Increment(x=w556) -> (x+1=w553:u16)
                      n331 = Replace Array Subset(array=w559, new element #1=w554, index #1=w555, new element #2=w553, index #2=w552) -> (w558:u16[])
                    }
                  }
                  n332 = local write "MTrig_Solenoid_trig__L"(w537) -> ()
                  n333 = local write "MTrig_Solenoid_trig__R"(w537) -> ()
                }
              }
              n334 = Select(t=myRIO_BRig_RT__Case_NonExp_stateList."Cue_pre", s=w473, f=myRIO_BRig_RT__Case_NonExp_stateList."DispenseWater_pre" ("Enum")) -> (s? t:f=w471:T1)
              n335 = Select(t=w471, s=w475, f=myRIO_BRig_RT__Case_NonExp_stateList."Idle_4" ("Enum")) -> (s? t:f=w476:T1)
            }
            frame "Idle_4" {
              # "use dataMTrig as it is one of the last to transfer"
              # "To ensure timing, we split the\nidle state into 4 phases"
              n336 = call "myRIO_BRig_RT_comm_webdav_uploadReceived_check_v2,0.vi"("input_dataName"="dataMTrig") -> ("output_Iexist"=w569:bool)  [unwired: 9 in, 1 out]
              n337 = Select(t=myRIO_BRig_RT__Case_NonExp_stateList."UploadSettings_pre" ("Enum"), s=w569, f=myRIO_BRig_RT__Case_NonExp_stateList."Idle") -> (s? t:f=w567:T1)
            }
            frame "Cue_pre" {
              w577 = u16 1 ("t")
              w576 = u16 0 ("new element/subarray")
              w573 = u16 0 ("new element/subarray")
              # "Ncycle"
              # "count"
              # "Audio_R"
              # "Solenoid_R"
              # "Solenoid_L"
              # "Ncycle"
              # "count"
              # "Audio_L"
              n338 = call "myRIO_BRig_RT_dataMTrig_Solenoid_N__L.vi"() -> ("output_Solenoid_N__L"=w588:i32)  [unwired: 11 in]
              n339 = call "myRIO_BRig_RT_dataMTrig_Solenoid_N__R.vi"() -> ("output_Solenoid_N__R"=w587:i32)  [unwired: 11 in]
              n340 = Index Array(array=w584, index #1=w588, index #2=w587) -> (element #1=w586:u16, element #2=w585:u16)
              n341 = Not Equal To 0?(x=w585) -> (x != 0?=w578:bool)
              n342 = Not Equal To 0?(x=w586) -> (x != 0?=w580:bool)
              n343 = Select(t=w577, s=w580, f=w576) -> (s? t:f=w579:u16)
              n344 = Select(t=w577, s=w578, f=w576) -> (s? t:f=w572:u16)
              n345 = call "myRIO_BRig_RT_dataMTrig_Audio_c__L.vi"() -> ("output_Audio_c__L"=w582:i32)  [unwired: 11 in]
              n346 = call "myRIO_BRig_RT_dataMTrig_Audio_N__L.vi"() -> ("output_Audio_N__L"=w581:i32)  [unwired: 11 in]
              n347 = call "myRIO_BRig_RT_dataMTrig_Audio_c__R.vi"() -> ("output_Audio_c__R"=w575:i32)  [unwired: 11 in]
              n348 = call "myRIO_BRig_RT_dataMTrig_Audio_N__R.vi"() -> ("output_Audio_N__R"=w574:i32)  [unwired: 11 in]
              n349 = Replace Array Subset(array=w584, new element #1=w573, index #1=w582, new element #2=w579, index #2=w581, new element #3=w573, index #3=w575, new element #4=w572, index #4=w574) -> (w583:u16[])
            }
            frame "Cue" {
              # "Ncycle"
              # "Audio_R"
              # "Ncycle"
              # "Audio_L"
              n350 = call "myRIO_BRig_RT_dataMTrig_Audio_N__L.vi"() -> ("output_Audio_N__L"=w604:i32)  [unwired: 11 in]
              n351 = call "myRIO_BRig_RT_dataMTrig_Audio_N__R.vi"() -> ("output_Audio_N__R"=w603:i32)  [unwired: 11 in]
              n352 = Index Array(array=w609, index #1=w604, index #2=w603) -> (element #1=w602:u16, element #2=w601:u16)
              n353 = Equal To 0?(x=w602) -> (x = 0?=w600:bool)
              n354 = Equal To 0?(x=w601) -> (x = 0?=w599:bool)
              n355 = And(x=w600, y=w599) -> (x .and. y?=w598:bool)
              n356 = Select(t=myRIO_BRig_RT__Case_NonExp_stateList."DispenseWater_pre", s=w598, f=w596) -> (s? t:f=w595:T1)
            }
            frame "RewardCalibration_pre" {
              (unwired) FALSE
              w615 = FALSE
              w626 = u8 0
              w642 = u8 0
              # "Are we starting a RewardCalibration?\nOr are we stopping a RewardCalibration?\nOr is a RewardCalibration over?"
              # "RewCalib\nOnOff"
              # "N"
              # "Solenoid R"
              # "RewCalib\nOnOff"
              # "N"
              # "Solenoid L"
              n357 = local read "RewCalib_Trig_L"() -> (w649:bool)
              n358 = local read "RewCalib_Trig_R"() -> (w618:bool)
              n359 = call "myRIO_BRig_RT_dataMTrig_Solenoid_N__R.vi"() -> ("output_Solenoid_N__R"=w620:i32)  [unwired: 11 in]
              n360 = call "myRIO_BRig_RT_dataMTrig_Solenoid_RewCalib_OnOff__R.vi"() -> ("output_Solenoid_RewCalib_OnOff__R"=w617:i32)  [unwired: 11 in]
              n361 = call "myRIO_BRig_RT_dataMTrig_Solenoid_N__L.vi"() -> ("output_Solenoid_N__L"=w635:i32)  [unwired: 11 in]
              n362 = call "myRIO_BRig_RT_dataMTrig_Solenoid_RewCalib_OnOff__L.vi"() -> ("output_Solenoid_RewCalib_OnOff__L"=w636:i32)  [unwired: 11 in]
              n363 = Index Array(array=w619, index #1=w620, index #2=w617) -> (element #1=w630:u16, element #2=w625:u16)
              n364 = Index Array(array=w619, index #1=w635, index #2=w636) -> (element #1=w646:u16, element #2=w641:u16)
              n365 = Equal To 0?(x=w630) -> (x = 0?=w631:bool)
              n366 = Not Equal To 0?(x=w625) -> (x != 0?=w628:bool)
              n367 = Equal To 0?(x=w646) -> (x = 0?=w647:bool)
              n368 = Not Equal To 0?(x=w641) -> (x != 0?=w644:bool)
              n369 = local write "MTrig_Solenoid_trig__L"(w615) -> ()
              n370 = local write "MTrig_Solenoid_trig__R"(w615) -> ()
              n371 = Select(t=u8 1, s=w618, f=w626) -> (s? t:f=w622:u8)
              n372 = Select(t=u8 1, s=w649, f=w642) -> (s? t:f=w638:u8)
              n373 = Select(t=u8 2, s=w631, f=w626) -> (s? t:f=w623:u8)
              n374 = Select(t=u8 4, s=w628, f=w626) -> (s? t:f=w624:u8)
              n375 = Select(t=u8 2, s=w647, f=w642) -> (s? t:f=w639:u8)
              n376 = Select(t=u8 4, s=w644, f=w642) -> (s? t:f=w640:u8)
              n377 = Compound Arithmetic op=ADD(w622, w623, w624) -> (w621:u8)
              n378 = Compound Arithmetic op=ADD(w638, w639, w640) -> (w637:u8)
              n379 = case shown="7" w637 {
                tunnel: w619 -> [w679 w684 w686 w691 w696 w698 w701 w706]
                tunnel: [w679 w685 w686 w692 w697 w698 w702 w707] -> w634
                tunnel: w636 -> [_ w682 _ w689 w694 _ w700 w705]
                tunnel: w635 -> [_ w683 _ w690 w695 _ _ _]
                frame 0, Default {
                }
                frame 1 {
                  n380 = Replace Array Subset(array=w684, new element #1=u16 100 ("new element/subarray"), index #1=w683, new element #2=u16 1 ("new element/subarray"), index #2=w682) -> (w685:u16[])
                }
                frame 2 {
                }
                frame 3 {
                  n381 = Replace Array Subset(array=w691, new element #1=u16 100 ("new element/subarray"), index #1=w690, new element #2=u16 1 ("new element/subarray"), index #2=w689) -> (w692:u16[])
                }
                frame 4 {
                  w693 = u16 0 ("new element/subarray")
                  n382 = Replace Array Subset(array=w696, new element #1=w693, index #1=w695, new element #2=w693, index #2=w694) -> (w697:u16[])
                }
                frame 5 {
                }
                frame 6 {
                  n383 = Replace Array Subset(array=w701, new element=u16 0 ("new element/subarray"), index=w700) -> (w702:u16[])
                }
                frame 7 {
                  n384 = local write "RewCalib_Trig_L"(FALSE ("RewCalib_Trig_L")) -> ()
                  n385 = Replace Array Subset(array=w706, new element=u16 0 ("new element/subarray"), index=w705) -> (w707:u16[])
                }
              }
              n386 = case shown="7" w621 {
                tunnel: w634 -> [w650 w655 w657 w662 w667 w669 w672 w677]
                tunnel: [w650 w656 w657 w663 w668 w669 w673 w678] -> w633
                tunnel: w617 -> [_ w653 _ w660 w665 _ w671 w676]
                tunnel: w620 -> [_ w654 _ w661 w666 _ _ _]
                frame 0, Default {
                }
                frame 1 {
                  n387 = Replace Array Subset(array=w655, new element #1=u16 100 ("new element/subarray"), index #1=w654, new element #2=u16 1 ("new element/subarray"), index #2=w653) -> (w656:u16[])
                }
                frame 2 {
                }
                frame 3 {
                  n388 = Replace Array Subset(array=w662, new element #1=u16 100 ("new element/subarray"), index #1=w661, new element #2=u16 1 ("new element/subarray"), index #2=w660) -> (w663:u16[])
                }
                frame 4 {
                  w664 = u16 0 ("new element/subarray")
                  n389 = Replace Array Subset(array=w667, new element #1=w664, index #1=w666, new element #2=w664, index #2=w665) -> (w668:u16[])
                }
                frame 5 {
                }
                frame 6 {
                  n390 = Replace Array Subset(array=w672, new element=u16 0 ("new element/subarray"), index=w671) -> (w673:u16[])
                }
                frame 7 {
                  n391 = local write "RewCalib_Trig_R"(FALSE ("RewCalib_Trig_L")) -> ()
                  n392 = Replace Array Subset(array=w677, new element=u16 0 ("new element/subarray"), index=w676) -> (w678:u16[])
                }
              }
            }
            frame "DispenseWater_pre" {
              w714 = u16 0 ("t")
              w757 = u16 0 ("new element/subarray")
              # "just trust me on this one"
              # "RewCalib\nOnOff"
              # "RewCalib\nOnOff"
              # "nCycle"
              # "Solenoid__R"
              # "Tdelay"
              # "delay"
              # "nCycle"
              # "Solenoid__L"
              # "Tdelay"
              # "delay"
              # "Solenoid__R"
              # "count"
              # "Solenoid_Tcycle_R"
              # "Solenoid_Tcycle_L"
              # "Solenoid__L"
              # "count"
              n393 = call "myRIO_BRig_RT_dataMTrig_Solenoid_RewCalib_OnOff__L.vi"() -> ("output_Solenoid_RewCalib_OnOff__L"=w721:i32)  [unwired: 11 in]
              n394 = call "myRIO_BRig_RT_dataMTrig_Solenoid_N__L.vi"() -> ("output_Solenoid_N__L"=w712:i32)  [unwired: 11 in]
              n395 = call "myRIO_BRig_RT_dataMTrig_Solenoid_delay__L.vi"() -> ("output_Solenoid_delay__L"=w755:i32)  [unwired: 11 in]
              n396 = call "myRIO_BRig_RT_dataMTrig_Solenoid_Tdelay__L.vi"() -> ("output_Solenoid_Tdelay__L"=w754:i32)  [unwired: 11 in]
              n397 = call "myRIO_BRig_RT_dataMTrig_Solenoid_N__R.vi"() -> ("output_Solenoid_N__R"=w710:i32)  [unwired: 11 in]
              n398 = call "myRIO_BRig_RT_dataMTrig_Solenoid_delay__R.vi"() -> ("output_Solenoid_delay__R"=w744:i32)  [unwired: 11 in]
              n399 = call "myRIO_BRig_RT_dataMTrig_Solenoid_Tdelay__R.vi"() -> ("output_Solenoid_Tdelay__R"=w743:i32)  [unwired: 11 in]
              n400 = call "myRIO_BRig_RT_dataMTrig_Solenoid_RewCalib_OnOff__R.vi"() -> ("output_Solenoid_RewCalib_OnOff__R"=w717:i32)  [unwired: 11 in]
              n401 = Index Array(array=w756, index #1=w712, index #2=w755, index #3=w754, index #4=w710, index #5=w744, index #6=w743, index #7=w721, index #8=w717) -> (element #1=w713:u16, element #2=w753:u16, element #3=w748:u16, element #4=w716:u16, element #5=w738:u16, element #6=w737:u16, element #7=w722:u16, element #8=w719:u16)
              n402 = Equal To 0?(x=w753) -> (x = 0?=w752:bool)
              n403 = Equal To 0?(x=w738) -> (x = 0?=w742:bool)
              n404 = local read "RewCalib_Trig_L"() -> (w733:bool)
              n405 = local read "RewCalib_Trig_R"() -> (w728:bool)
              n406 = Not Equal To 0?(x=w713) -> (x != 0?=w751:bool)
              n407 = Not Equal To 0?(x=w716) -> (x != 0?=w741:bool)
              n408 = local read "MTrig_Solenoid_Tcycle__L"() -> (w750:u16)
              n409 = local read "MTrig_Solenoid_Tcycle__R"() -> (w736:u16)
              n410 = Not Equal To 0?(x=w722) -> (x != 0?=w732:bool)
              n411 = Not Equal To 0?(x=w719) -> (x != 0?=w730:bool)
              n412 = Not(x=w733) -> (.not. x?=w731:bool)
              n413 = Not(x=w728) -> (.not. x?=w729:bool)
              n414 = And(x=w732, y=w731) -> (x .and. y?=w727:bool)
              n415 = And(x=w730, y=w729) -> (x .and. y?=w726:bool)
              n416 = call "myRIO_BRig_RT_dataMTrig_Solenoid_c__L.vi"() -> ("output_Solenoid_c__L"=w759:i32)  [unwired: 11 in]
              n417 = call "myRIO_BRig_RT_dataMTrig_Solenoid_c__R.vi"() -> ("output_Solenoid_c__R"=w758:i32)  [unwired: 11 in]
              n418 = Select(t=w750, s=w751, f=u16 0) -> (s? t:f=w747:u16)
              n419 = Or(x=w727, y=w726) -> (x .or. y?=w715:bool)
              n420 = Select(t=w736, s=w741, f=u16 0) -> (s? t:f=w739:u16)
              n421 = Select(t=w747, s=w752, f=w748) -> (s? t:f=w745:u16)
              n422 = Select(t=w739, s=w742, f=w737) -> (s? t:f=w734:u16)
              n423 = call "myRIO_BRig_RT_dataMTrig_Solenoid_Tcycle__L.vi"() -> ("output_Solenoid_Tcycle__L"=w746:i32)  [unwired: 11 in]
              n424 = call "myRIO_BRig_RT_dataMTrig_Solenoid_Tcycle__R.vi"() -> ("output_Solenoid_Tcycle__R"=w735:i32)  [unwired: 11 in]
              n425 = Select(t=w714, s=w715, f=w713) -> (s? t:f=w711:u16)
              n426 = Select(t=w714, s=w715, f=w716) -> (s? t:f=w709:u16)
              n427 = Select(t=myRIO_BRig_RT__Case_NonExp_stateList."Idle" ("Enum"), s=w715, f=myRIO_BRig_RT__Case_NonExp_stateList."DispenseWater" ("Enum")) -> (s? t:f=w723:T1)
              n428 = Select(t=w714, s=w715, f=w722) -> (s? t:f=w720:u16)
              n429 = Select(t=w714, s=w715, f=w719) -> (s? t:f=w718:u16)
              n430 = Replace Array Subset(array=w756, new element #1=w757, index #1=w759, new element #2=w757, index #2=w758, new element #3=w745, index #3=w746, new element #4=w734, index #4=w735, new element #5=w720, index #5=w721, new element #6=w718, index #6=w717, new element #7=w711, index #7=w712, new element #8=w709, index #8=w710) -> (w760:u16[])
            }
            frame "DispenseWater" {
              # "D"
              # "C"
              # "B"
              # "A"
              # "(A) Add COUNT and INCREMENT\n(B) Is (A) smaller than Tcycle?\n(C) Are we dispensing water or in the delay phase?\n(D) If (A) is smaller than Tcycle   AND   if we are dispensing water\n      then send TRUE to solenoid"
              # "delay"
              # "Tcycle"
              # "Solenoid__R"
              # "count"
              # "delay"
              # "Tcycle"
              # "Solenoid__L"
              # "count"
              n431 = To Unsigned Word Integer(number=w791) -> (unsigned 16bit integer=w773:u16)
              n432 = call "myRIO_BRig_RT_dataMTrig_Solenoid_delay__R.vi"() -> ("output_Solenoid_delay__R"=w777:i32)  [unwired: 11 in]
              n433 = call "myRIO_BRig_RT_dataMTrig_Solenoid_c__R.vi"() -> ("output_Solenoid_c__R"=w776:i32)  [unwired: 11 in]
              n434 = call "myRIO_BRig_RT_dataMTrig_Solenoid_Tcycle__R.vi"() -> ("output_Solenoid_Tcycle__R"=w778:i32)  [unwired: 11 in]
              n435 = call "myRIO_BRig_RT_dataMTrig_Solenoid_delay__L.vi"() -> ("output_Solenoid_delay__L"=w793:i32)  [unwired: 11 in]
              n436 = call "myRIO_BRig_RT_dataMTrig_Solenoid_c__L.vi"() -> ("output_Solenoid_c__L"=w785:i32)  [unwired: 11 in]
              n437 = call "myRIO_BRig_RT_dataMTrig_Solenoid_Tcycle__L.vi"() -> ("output_Solenoid_Tcycle__L"=w794:i32)  [unwired: 11 in]
              n438 = Index Array(array=w787, index #1=w785, index #2=w794, index #3=w793, index #4=w776, index #5=w778, index #6=w777) -> (element #1=w792:u16, element #2=w782:u16, element #3=w790:u16, element #4=w772:u16, element #5=w769:u16, element #6=w768:u16)
              n439 = Add(x=w792, y=w773) -> (x+y=w783:u16)
              n440 = Add(x=w772, y=w773) -> (x+y=w774:u16)
              n441 = Less?(x=w783, y=w782) -> (x < y?=w766:bool)
              n442 = Equal To 0?(x=w790) -> (x = 0?=w789:bool)
              n443 = Less?(x=w774, y=w769) -> (x < y?=w767:bool)
              n444 = Equal To 0?(x=w768) -> (x = 0?=w775:bool)
              n445 = And(x=w766, y=w789) -> (x .and. y?=w788:bool)
              n446 = Or(x=w766, y=w767) -> (x .or. y?=w765:bool)
              n447 = And(x=w767, y=w775) -> (x .and. y?=w770:bool)
              n448 = Select(t=w783, s=w766, f=w782) -> (s? t:f=w784:u16)
              n449 = Select(t=w774, s=w767, f=w769) -> (s? t:f=w771:u16)
              n450 = Replace Array Subset(array=w787, new element #1=w784, index #1=w785, new element #2=w771, index #2=w776) -> (w786:u16[])
              n451 = Select(t=w781, s=w765, f=myRIO_BRig_RT__Case_NonExp_stateList."DispenseWater_post" ("Enum")) -> (s? t:f=w779:T1)
            }
            frame "DispenseWater_post" {
              # "nCycle"
              # "delay"
              # "Solenoid__R"
              # "nCycle"
              # "delay"
              # "Solenoid__L"
              n452 = call "myRIO_BRig_RT_dataMTrig_Solenoid_N__L.vi"() -> ("output_Solenoid_N__L"=w816:i32)  [unwired: 11 in]
              n453 = call "myRIO_BRig_RT_dataMTrig_Solenoid_delay__L.vi"() -> ("output_Solenoid_delay__L"=w815:i32)  [unwired: 11 in]
              n454 = call "myRIO_BRig_RT_dataMTrig_Solenoid_N__R.vi"() -> ("output_Solenoid_N__R"=w812:i32)  [unwired: 11 in]
              n455 = call "myRIO_BRig_RT_dataMTrig_Solenoid_delay__R.vi"() -> ("output_Solenoid_delay__R"=w811:i32)  [unwired: 11 in]
              n456 = Index Array(array=w818, index #1=w816, index #2=w815, index #3=w812, index #4=w811) -> (element #1=w820:u16, element #2=w819:u16, element #3=w803:u16, element #4=w805:u16)
              n457 = Not Equal To 0?(x=w820) -> (x != 0?=w821:bool)
              n458 = Not Equal To 0?(x=w803) -> (x != 0?=w804:bool)
              n459 = case shown="True" w804 {
                selector: w804 -> [_ w829]
                tunnel: w803 -> [w827 w835]
                tunnel: w805 -> [_ w836]
                tunnel: [w827 w833] -> w802
                tunnel: [u16 0 w832] -> w801
                tunnel: [_ w829] -> w800
                frame False {
                }
                frame True {
                  n460 = Equal To 0?(x=w836) -> (x = 0?=w828:bool)
                  n461 = Decrement(x=w835) -> (x-1=w834:u16)
                  n462 = Select(t=w834, s=w828, f=w835) -> (s? t:f=w833:u16)
                  n463 = Select(t=u16 1, s=w828, f=u16 0) -> (s? t:f=w832:u16)
                }
              }
              n464 = case shown="True" w821 {
                selector: w821 -> [_ w840]
                tunnel: w820 -> [w838 w846]
                tunnel: w819 -> [_ w847]
                tunnel: [w838 w844] -> w814
                tunnel: [u16 0 w843] -> w813
                tunnel: [_ w840] -> w810
                frame False {
                }
                frame True {
                  n465 = Equal To 0?(x=w847) -> (x = 0?=w839:bool)
                  n466 = Decrement(x=w846) -> (x-1=w845:u16)
                  n467 = Select(t=w845, s=w839, f=w846) -> (s? t:f=w844:u16)
                  n468 = Select(t=u16 1, s=w839, f=u16 0) -> (s? t:f=w843:u16)
                }
              }
              n469 = Or(x=w810, y=w800) -> (x .or. y?=w809:bool)
              n470 = Replace Array Subset(array=w818, new element #1=w814, index #1=w816, new element #2=w813, index #2=w815, new element #3=w802, index #3=w812, new element #4=w801, index #4=w811) -> (w817:u16[])
              n471 = Select(t=myRIO_BRig_RT__Case_NonExp_stateList."DispenseWater_pre" ("Enum"), s=w809, f=myRIO_BRig_RT__Case_NonExp_stateList."Idle" ("Enum")) -> (s? t:f=w806:T1)
            }
            frame "TestConnection" {
              n472 = local read "Host Password"() -> (w858:string)
              n473 = local read "Host UserName"() -> (w859:string)
              n474 = call "myRIO_BRig_RT_comm_webdav_testConnect.vi"("input_password"=w858, "input_username"=w859) -> ("output_Iconnected"=w856:bool)  [unwired: 9 in]
              n475 = Select(t="Connection accepted!" ("message"), s=w856, f="Error!") -> (s? t:f=w854:string)
              n476 = One Button Dialog(message=w854) -> ()  [unwired: 1 in, 1 out]
            }
            frame "SendData" {
              n477 = local read "Host Filename Prefix"() -> (w861:string)
              n478 = local read "Host Password"() -> (w862:string)
              n479 = local read "Host UserName"() -> (w863:string)
              n480 = call "myRIO_BRig_RT_comm_webdav_sendData_all.vi"("Host Filename Prefix"=w861, "Host Password"=w862, "Host UserName"=w863) -> ()  [unwired: 9 in]
            }
            frame "End" {
            }
          }
          n481 = local read "MTrig_Audio_trig__R"() -> (w81:bool)
          n482 = local read "MTrig_Audio_trig__L"() -> (w80:bool)
          n483 = local read "START"() -> (w76:bool)
          n484 = local read "STOP_abort"() -> (w75:bool)
          n485 = local read "MTrig_Laser_trig"() -> (w82:bool)
          n486 = call "myRIO_BRig_RT_dataMTrig_main__v2.vi"("input_dataMTrig"=w84, "input_Audio_trig_L"=w80, "input_Audio_trig_R"=w81, "input_Laser_trig"=w82) -> ("output_dataMTrig"=w83:u16[], "output_Audio_L"=w60:bool, "output_Audio_R"=w71:bool, "output_Laser"=w63:bool)  [unwired: 12 in]
          n487 = Or(x=w76, y=w75) -> (x .or. y?=w74:bool)
          n488 = local read "A6"() -> (w53:bool)
          n489 = Select(t=myRIO_BRig_RT__Case_NonExp_stateList."End" ("Enum"), s=w74, f=w73) -> (s? t:f=w72:T1)
          n490 = Or(x=w81, y=w82) -> (x .or. y?=w79:bool)
          n491 = Or(x=w79, y=w80) -> (x .or. y?=w78:bool)
          n492 = case shown="True" w78 {
            frame False {
            }
            frame True {
              w109 = FALSE
              n493 = local write "MTrig_Audio_trig__R"(w109) -> ()
              n494 = local write "MTrig_Audio_trig__L"(w109) -> ()
              n495 = local write "MTrig_Laser_trig"(w109) -> ()
            }
          }
          n496 = xnode "Read/Write Control"("FPGA VI Reference In"=w101, "error in"=w99, "A6_Act"=w53, "A1_SR"=w85, "A3_SL"=w86, "audioTrigger_L"=w60, "audioAmp_L"=w90, "audioFreq_L_Hz"=w89, "audioTrigger_R"=w71, "audioAmp_R"=w88, "audioFreq_R_Hz"=w87, "laserResponse_reward_LED"="laserResponse_reward_LED", "laserResponse_wrong_LED"="laserResponse_wrong_LED", "laserResponse_reward"="laserResponse_reward", "laserResponse_wrong"="laserResponse_wrong", "SelectionState"="SelectionState", "ignoreWrong"="ignoreWrong", "Left(F)_or_Right(T)"="Left(F)_or_Right(T)", "laserMTrig"=w63, "tCycle_laser_rew"="tCycle_laser_rew", "tDelay_laser_rew"="tDelay_laser_rew", "tCycle_laser_wro"="tCycle_laser_wro", "tDelay_laser_wro"="tDelay_laser_wro") -> ("FPGA VI Reference Out"=w100:refnum<k20>, "error out"=w98:errorcluster, "SelectReward"=→"SelectReward":bool, "SelectWrong"=→"SelectWrong":bool)
          n497 = node-c288() -> ()  [unwired: 1 in, 1 out]
          "cState_NonExp" <- w97
        }
        n498 = node-c288(w48) -> ()  [unwired: 1 out]
        n499 = flat-sequence {
          tunnel: w41 -> [w52]
          tunnel: [w52] -> w40
          tunnel: w39 -> [w51]
          tunnel: [w51] -> w38
          frame #0 {
            w50 = FALSE
            n500 = local write "STOP_endBlock"(w50) -> ()
            n501 = local write "STOP_endTrial"(w50) -> ()
          }
        }
      }
      frame True {
        w885 = FALSE ("SelectionState")
        w890 = u16 0 ("idxDataBlock")
        w892 = u16 100 ("new element/subarray")
        w893 = u16 100 ("new element/subarray")
        w913 = T6 refnum items=["Session NI_WebDAV"] ("output_hSession")
        w922 = FALSE
        w923 = u16 0
        w884 = FALSE
        # "audio__L\naudio__R"
        # "Audio params"
        # "nRewards"
        # "idxDataBlock"
        # "Solenoid_Tdelay_R"
        # "Solenoid_Tdelay_L"
        # "RewCalib_N__R"
        # "RewCalib_N__L"
        # "Save dataLick to file\nSend file to Host\nSave dataMTrig\nSend file to Host\nDisconnect"
        # "dataTrial"
        # "dataTrial"
        # "Solenoid_Tcycle_R"
        # "Solenoid_Tcycle_L"
        # "Laser_Tcycle"
        # "Audio_Tcycle_R"
        # "Audio_Tcycle_L"
        # "dataLick"
        # "dataLC"
        # "dataLC"
        # "dataBlock"
        # "dataBlock"
        # "dataMTrig"
        # "dataMTrig"
        # "dataExp"
        # "dataCurrent"
        # "dataExp"
        # "dataCurrent"
        # "spout"
        # "state"
        n502 = call "myRIO_BRig_RT_dataMTrig_Solenoid_Tcycle__L.vi"() -> ("output_Solenoid_Tcycle__L"=w919:i32)  [unwired: 11 in]
        n503 = call "myRIO_BRig_RT_dataMTrig_Solenoid_Tcycle__R.vi"() -> ("output_Solenoid_Tcycle__R"=w918:i32)  [unwired: 11 in]
        n504 = call "myRIO_BRig_RT_dataMTrig_Audio_Tcycle__L.vi"() -> ("output_Audio_Tcycle__L"=w917:i32)  [unwired: 11 in]
        n505 = call "myRIO_BRig_RT_dataMTrig_Audio_Tcycle__R.vi"() -> ("output_Audio_Tcycle__R"=w916:i32)  [unwired: 11 in]
        n506 = call "myRIO_BRig_RT_dataMTrig_Laser_Tcycle.vi"() -> ("output_Laser_Tcycle"=w915:i32)  [unwired: 11 in]
        n507 = local read "MTrig_Solenoid_Tcycle__L"() -> (w898:u16)
        n508 = local read "MTrig_Solenoid_Tcycle__R"() -> (w897:u16)
        n509 = local read "Tcycle_Reward_L"() -> (w894:u16)
        n510 = local read "Tcycle_Reward_R"() -> (w895:u16)
        n511 = local read "MTrig_Laser_Tcycle"() -> (w896:u16)
        n512 = call "myRIO_BRig_RT_dataMTrig_Solenoid_RewCalib_nCycle__L.vi"() -> ("output_Solenoid_RewCalib_nCycle__L"=w901:i32)  [unwired: 11 in]
        n513 = call "myRIO_BRig_RT_dataMTrig_Solenoid_Tdelay__L.vi"() -> ("output_Solenoid_Tdelay__L"=w903:i32)  [unwired: 11 in]
        n514 = call "myRIO_BRig_RT_dataMTrig_Solenoid_RewCalib_nCycle__R.vi"() -> ("output_Solenoid_RewCalib_nCycle__R"=w902:i32)  [unwired: 11 in]
        n515 = call "myRIO_BRig_RT_dataMTrig_Solenoid_Tdelay__R.vi"() -> ("output_Solenoid_Tdelay__R"=w904:i32)  [unwired: 11 in]
        n516 = call "myRIO_BRig_RT_dataLick_init.vi"() -> ("output_dataLick"=w925:u16[][])  [unwired: 11 in]
        n517 = call "myRIO_BRig_RT_dataCurrent_init.vi"() -> ("output_dataCurrent"=w932:u16[])  [unwired: 11 in]
        n518 = call "myRIO_BRig_RT_dataExp_init.vi"() -> ("output_dataExp"=w931:u16[])  [unwired: 11 in]
        n519 = call "myRIO_BRig_RT_dataMTrig_init.vi"() -> ("output_dataMTrig"=w921:u16[])  [unwired: 5 in]
        n520 = call "myRIO_BRig_RT_dataLC_init.vi"() -> ("output_dataLC"=w929:u16[])  [unwired: 11 in]
        n521 = call "myRIO_BRig_RT_dataBlock_init.vi"() -> ("output_dataBlock"=w930:u16[][])  [unwired: 11 in]
        n522 = call "myRIO_BRig_RT_dataTrial_init.vi"() -> ("output_dataTrial"=w914:u16[][])  [unwired: 11 in]
        n523 = xnode "Read/Write Control"("FPGA VI Reference In"=w886, "error in"=w887, "SelectionState"=w885, "laserResponse_reward"=w885, "laserResponse_wrong"=w885, "laserResponse_reward_LED"=w885, "laserResponse_wrong_LED"=w885, "Left(F)_or_Right(T)"=w885, "ignoreWrong"=w885, "SelectionState"=w885) -> ("FPGA VI Reference Out"=w888:refnum<k20>, "error out"=w889:errorcluster)
        n524 = Replace Array Subset(array=w921, new element #1=w893, index #1=w901, new element #2=w893, index #2=w902, new element #3=w892, index #3=w903, new element #4=w892, index #4=w904, new element #5=w898, index #5=w919, new element #6=w897, index #6=w918, new element #7=w894, index #7=w917, new element #8=w895, index #8=w916, new element #9=w896, index #9=w915) -> (w920:u16[])
        n525 = Get Date/Time In Seconds() -> (seconds since 1Jan1904=w900:timestamp)
        n526 = To Double Precision Float(number=w900) -> (double precision float=w899:dbl)
        n527 = node-c288() -> (w940:T3)  [unwired: 4 in]
        n528 = timed-loop {
          timing: w940 -> [_]
          timing-out: [_] -> w939
          shift-right: [w1018] -> _
          shift-left: myRIO_BRig_RT__Case_Exp_stateList."Start1" ("Enum") -> [w1049]
          shift-right: [w1070] -> _
          shift-left: enum16{"Left", "Right"}."Left" -> [w1072]
          tunnel: w888 -> [w1069]
          tunnel: w889 -> [w1068]
          shift-right: [w1063] -> _
          shift-left: w937 -> [w1067]
          shift-right: [w1062] -> _
          shift-left: w936 -> [w1066]
          tunnel: [w1043] -> w934
          tunnel: [w1044] -> w935
          shift-right: [w1045] -> w905
          shift-left: w932 -> [w1010]
          shift-right: [w1061] -> _
          shift-left: w931 -> [w1005]
          shift-right: [w1032] -> w909
          shift-left: w920 -> [w1033]
          shift-right: [w1059] -> _
          shift-left: w930 -> [w1060]
          shift-right: [w1057] -> _
          shift-left: w929 -> [w1058]
          shift-right: [w990] -> _
          shift-left: w884 -> [w1056]
          shift-right: [w1047] -> w911
          shift-left: w925 -> [w1048]
          shift-right: [w1034] -> _
          shift-left: w923 -> [w1042]
          shift-right: [w1002] -> _
          shift-left: w923 -> [w1041]
          shift-right: [w1035] -> _
          shift-left: w923 -> [w1040]
          shift-right: [w1036] -> _
          shift-left: w923 -> [w1039]
          shift-right: [w1003] -> _
          shift-left: w922 -> [w1037]
          shift-right: [w1004] -> _
          shift-left: w922 -> [w1038]
          shift-right: [w1016] -> _
          shift-left: w914 -> [w1017]
          shift-right: [w1015] -> w907
          shift-left: w913 -> [w1013]
          shift-right: [w1014] -> w908
          shift-left: FALSE ("output_Iconnected") -> [w1012]
          tunnel: "Host Filename Prefix" -> [w1011]
          tunnel: [w1011] -> w906
          shift-right: [w985] -> _
          shift-left: w884 -> [w1009]
          tunnel: w899 -> [w1006]
          shift-right: [w1000] -> _
          shift-left: 0 ("idxDataBlock") -> [w1001]
          shift-right: [w997] -> _
          shift-left: w890 -> [w999]
          shift-right: [w996] -> _
          shift-left: w890 -> [w998]
          shift-right: [w984] -> _
          shift-left: w884 -> [w991]
          shift-right: [w987] -> _
          shift-left: w884 -> [w989]
          shift-right: [w986] -> _
          shift-left: w884 -> [w988]
          shift-right: [w977] -> _
          shift-left: w884 -> [w978]
          stop <- w1055 stop-if-true
          # "Laser"
          # "Audio R"
          # "Audio L"
          # "Solenoid R"
          # "Solenoid L"
          # "manual triggering"
          # "dataTrial"
          # "dataBlock"
          # "nRewards"
          # "laserOccurred"
          # "dataExp"
          # "dataCurrent"
          # "audio__L\naudio__R"
          # "time stamp"
          # "Audio params"
          # "nRewards"
          # "idxDataBlock"
          # "idxDataBlock"
          # "activate"
          # "audio__L\naudio__R"
          # "amp__R\nfreq__R"
          # "amp__L\nfreq__L"
          # "dataLC"
          # "solenoid__R"
          # "solenoid__L"
          # "Did a lick occur?"
          # "Update lick counter"
          # "spout"
          # "spout"
          # "state"
          # "state"
          n529 = node-c288() -> ()  [unwired: 1 in, 1 out]
          n530 = local read "MTrig_Solenoid_trig__L"() -> (w1030:bool)
          n531 = local read "MTrig_Solenoid_trig__R"() -> (w1029:bool)
          n532 = local read "MTrig_Audio_trig__L"() -> (w1028:bool)
          n533 = local read "MTrig_Audio_trig__R"() -> (w1027:bool)
          n534 = xnode "Read/Write Control"("FPGA VI Reference In"=w1069, "error in"=w1068) -> ("FPGA VI Reference Out"=w995:refnum<k20>, "error out"=w994:errorcluster, "A2_LickL"=w1063:u32, "A4_LickR"=w1062:u32)
          "A2" <- w1063
          "A4" <- w1062
          n535 = local read "MTrig_Laser_trig"() -> (w1026:bool)
          n536 = Greater?(x=w1063, y=w1067) -> (0:w1065:bool)
          n537 = Greater?(x=w1062, y=w1066) -> (0:w1064:bool)
          n538 = Or(x=w1065, y=w1064) -> (x .or. y?=w1071:bool)
          n539 = call "myRIO_BRig_RT_dataMTrig_main.vi"("input_dataMTrig"=w1033, "input_Solenoid_trig_L"=w1030, "input_Solenoid_trig_R"=w1029, "input_Audio_trig_L"=w1028, "input_Audio_trig_R"=w1027, "input_Laser_trig"=w1026) -> ("output_Laser"=w982:bool, "output_dataMTrig"=w1032:u16[], "output_Solenoid_L"=w1020:bool, "output_Solenoid_R"=w1022:bool, "output_Audio_L"=w1024:bool, "output_Audio_R"=w1025:bool)  [unwired: 8 in]
          n540 = Compound Arithmetic op=OR(w1030, w1029, w1028, w1027, w1026) -> (w1031:bool)
          n541 = case shown="True" w1031 {
            frame False {
            }
            frame True {
              w1073 = FALSE
              n542 = local write "MTrig_Solenoid_trig__L"(w1073) -> ()
              n543 = local write "MTrig_Solenoid_trig__R"(w1073) -> ()
              n544 = local write "MTrig_Audio_trig__L"(w1073) -> ()
              n545 = local write "MTrig_Audio_trig__R"(w1073) -> ()
              n546 = local write "MTrig_Laser_trig"(w1073) -> ()
            }
          }
          n547 = case shown="\"setSettings_Laser\"" w1049 {
            selector: w1049 -> [_ _ _ _ _ _ _ _ _ _ _ _ _ _ _ _ _ _ _ w1747 _ w1815 _ _ _ _ _ w1953 _ w2029 _ _ _ _ _ w2161 _ w2238 _ w2302 _ w2346 _ _ w2413 _ _ _ _ _ w2581 _ _ _ _ _ _ _ _ _ _ _ _]
            tunnel: [myRIO_BRig_RT__Case_Exp_stateList."Start2" ("Enum") myRIO_BRig_RT__Case_Exp_stateList."Start3" ("Enum") myRIO_BRig_RT__Case_Exp_stateList."saveSettings1" ("Enum") myRIO_BRig_RT__Case_Exp_stateList."saveSettings2" ("Enum") myRIO_BRig_RT__Case_Exp_stateList."saveSettings3" ("Enum") myRIO_BRig_RT__Case_Exp_stateList."saveSettings4_LC_ENL" ("Enum") myRIO_BRig_RT__Case_Exp_stateList."saveSettings5_LC_Cue" ("Enum") myRIO_BRig_RT__Case_Exp_stateList."saveSettings6_LC_Other" ("Enum") myRIO_BRig_RT__Case_Exp_stateList."setSettings_Audio" ("Enum") myRIO_BRig_RT__Case_Exp_stateList."setSettings_Laser" ("Enum") myRIO_BRig_RT__Case_Exp_stateList."commConnect" ("Enum") w1544 myRIO_BRig_RT__Case_Exp_stateList."initTrial" ("Enum") w1584 myRIO_BRig_RT__Case_Exp_stateList."initTrial3" ("Enum") myRIO_BRig_RT__Case_Exp_stateList."initTrial_LC_ENL1" ("Enum") myRIO_BRig_RT__Case_Exp_stateList."initTrial_LC_Cue1" ("Enum") myRIO_BRig_RT__Case_Exp_stateList."ENL1_pre" ("Enum") w1706 w1744 myRIO_BRig_RT__Case_Exp_stateList."ENL1Penalty" ("Enum") w1816 myRIO_BRig_RT__Case_Exp_stateList."endExp" ("Enum") myRIO_BRig_RT__Case_Exp_stateList."endExp" ("Enum") myRIO_BRig_RT__Case_Exp_stateList."endExp" ("Enum") myRIO_BRig_RT__Case_Exp_stateList."endExp" ("Enum") w1909 w1952 myRIO_BRig_RT__Case_Exp_stateList."Cue1Penalty" ("Enum") w2027 myRIO_BRig_RT__Case_Exp_stateList."endExp" ("Enum") myRIO_BRig_RT__Case_Exp_stateList."endExp" ("Enum") myRIO_BRig_RT__Case_Exp_stateList."endExp" ("Enum") myRIO_BRig_RT__Case_Exp_stateList."endExp" ("Enum") w2115 w2169 myRIO_BRig_RT__Case_Exp_stateList."SelectReward" ("Enum") w2239 myRIO_BRig_RT__Case_Exp_stateList."SelectRewardPost" ("Enum") w2303 myRIO_BRig_RT__Case_Exp_stateList."SelectWrong" ("Enum") w2342 myRIO_BRig_RT__Case_Exp_stateList."endTrial1" ("Enum") myRIO_BRig_RT__Case_Exp_stateList."SelectTimeout" ("Enum") w2415 myRIO_BRig_RT__Case_Exp_stateList."endTrial1" ("Enum") myRIO_BRig_RT__Case_Exp_stateList."endTrial2" ("Enum") myRIO_BRig_RT__Case_Exp_stateList."saveData_dataBlock" ("Enum") w2494 w2564 w2581 myRIO_BRig_RT__Case_Exp_stateList."initBlock" ("Enum") w2608 myRIO_BRig_RT__Case_Exp_stateList."commUpload_dataCurrent" ("Enum") myRIO_BRig_RT__Case_Exp_stateList."commUpload_dataExp" ("Enum") myRIO_BRig_RT__Case_Exp_stateList."commUpload_dataLC" ("Enum") myRIO_BRig_RT__Case_Exp_stateList."commUpload_dataTrial" ("Enum") myRIO_BRig_RT__Case_Exp_stateList."endTrial3" ("Enum") myRIO_BRig_RT__Case_Exp_stateList."saveData_dataCurrent" ("Enum") myRIO_BRig_RT__Case_Exp_stateList."saveData_dataExp" ("Enum") myRIO_BRig_RT__Case_Exp_stateList."saveData_dataLC" ("Enum") myRIO_BRig_RT__Case_Exp_stateList."saveData_dataTrial" ("Enum") myRIO_BRig_RT__Case_Exp_stateList."commUpload_pre" ("Enum")] -> w1018
            tunnel: [w1099 w1119 w1141 w1198 w1242 w1299 w1351 w1403 w1447 w1471 w1516 w1520 w1552 w1585 w1608 w1629 w1656 w1681 w1722 w1760 w1793 w1820 w1836 w1858 w1877 w1896 w1928 w1974 w2000 w2026 w2047 w2068 w2087 w2106 w2126 w2187 w2212 w2235 w2250 w2300 w2324 w2357 w2378 w2394 w2426 w2449 w2461 w2480 w2518 w2537 w2580 w2597 w2611 w2645 w2666 w2687 w2708 w2729 w2757 w2777 w2804 w2824 w2849] -> w1070
            tunnel: w1072 -> [w1099 w1119 w1141 w1198 w1242 w1299 w1351 w1403 w1447 w1471 w1516 w1543 w1552 w1585 w1608 w1629 w1656 w1681 w1722 w1760 w1793 w1820 w1836 w1858 w1877 w1896 w1928 w1974 w2000 w2026 w2047 w2068 w2087 w2106 w2126 w2187 w2212 w2235 w2250 w2300 w2324 w2357 w2378 w2394 w2426 w2449 w2461 w2480 w2518 w2537 w2580 w2597 w2611 w2645 w2666 w2687 w2708 w2729 w2757 w2777 w2804 w2824 w2849]
            tunnel: w1071 -> [w1102 w1122 w1138 w1201 w1245 w1302 w1354 w1406 w1450 w1474 w1519 w1537 w1563 w1586 w1626 w1646 w1669 w1694 w1709 w1741 w1796 w1823 w1842 w1861 w1880 w1899 w1908 w1951 w2008 w2033 w2052 w2071 w2090 w2109 w2124 w2185 w2222 w2246 w2281 w2308 w2335 w2360 w2377 w2406 w2431 w2446 w2469 w2479 w2529 w2563 w2584 w2594 w2620 w2648 w2669 w2690 w2711 w2732 w2760 w2780 w2807 w2827 w2852]
            tunnel: w1065 -> [w1101 w1121 w1139 w1200 w1244 w1301 w1353 w1405 w1449 w1473 w1518 w1536 w1562 w1587 w1625 w1647 w1670 w1695 w1732 w1762 w1795 w1822 w1841 w1860 w1879 w1898 w1942 w1975 w2007 w2032 w2051 w2070 w2089 w2108 w2125 w2184 w2221 w2245 w2280 w2307 w2334 w2359 w2376 w2405 w2430 w2447 w2470 w2478 w2528 w2562 w2583 w2595 w2621 w2647 w2668 w2689 w2710 w2731 w2759 w2779 w2806 w2826 w2851]
            tunnel: w1064 -> [w1100 w1120 w1140 w1199 w1243 w1300 w1352 w1404 w1448 w1472 w1517 w1535 w1561 w1588 w1624 w1648 w1671 w1696 w1731 w1761 w1794 w1821 w1840 w1859 w1878 w1897 w1941 w1976 w2006 w2031 w2050 w2069 w2088 w2107 w2144 w2188 w2220 w2244 w2279 w2306 w2333 w2358 w2375 w2404 w2429 w2448 w2471 w2477 w2527 w2561 w2582 w2596 w2622 w2646 w2667 w2688 w2709 w2730 w2758 w2778 w2805 w2825 w2850]
            tunnel: [w1102 w1122 w1138 w1201 w1245 w1302 w1354 w1406 w1450 w1474 w1519 w1537 w1563 w1586 w1626 w1646 w1669 w1694 w1709 w1741 w1796 w1823 w1842 w1861 w1880 w1899 w1908 w1951 w2008 w2033 w2052 w2071 w2090 w2109 w2124 w2185 w2222 w2246 w2281 w2308 w2335 w2360 w2377 w2406 w2431 w2446 w2469 w2479 w2529 w2563 w2584 w2594 w2620 w2648 w2669 w2690 w2711 w2732 w2760 w2780 w2807 w2827 w2852] -> w1052
            tunnel: [w1101 w1121 w1139 w1200 w1244 w1301 w1353 w1405 w1449 w1473 w1518 w1536 w1562 w1587 w1625 w1647 w1670 w1695 w1732 w1762 w1795 w1822 w1841 w1860 w1879 w1898 w1942 w1975 w2007 w2032 w2051 w2070 w2089 w2108 w2125 w2184 w2221 w2245 w2280 w2307 w2334 w2359 w2376 w2405 w2430 w2447 w2470 w2478 w2528 w2562 w2583 w2595 w2621 w2647 w2668 w2689 w2710 w2731 w2759 w2779 w2806 w2826 w2851] -> w1051
            tunnel: [w1100 w1120 w1140 w1199 w1243 w1300 w1352 w1404 w1448 w1472 w1517 w1535 w1561 w1588 w1624 w1648 w1671 w1696 w1731 w1761 w1794 w1821 w1840 w1859 w1878 w1897 w1941 w1976 w2006 w2031 w2050 w2069 w2088 w2107 w2144 w2188 w2220 w2244 w2279 w2306 w2333 w2358 w2375 w2404 w2429 w2448 w2471 w2477 w2527 w2561 w2582 w2596 w2622 w2646 w2667 w2688 w2709 w2730 w2758 w2778 w2805 w2825 w2850] -> w1050
            tunnel: w1010 -> [w1098 w1118 w1137 w1159 w1218 w1276 w1350 w1402 w1446 w1469 w1496 w1542 w1551 w1583 w1597 w1630 w1653 w1680 w1721 w1746 w1787 w1819 w1837 w1857 w1876 w1895 w1912 w1971 w1999 w2030 w2048 w2067 w2086 w2105 w2135 w2165 w2204 w2241 w2252 w2305 w2325 w2356 w2374 w2395 w2428 w2445 w2458 w2482 w2498 w2535 w2579 w2598 w2623 w2642 w2663 w2684 w2705 w2716 w2746 w2765 w2789 w2821 w2838]
            tunnel: w1005 -> [w1097 w1117 w1136 w1196 w1240 w1296 w1348 w1400 w1444 w1462 w1512 w1541 w1560 w1582 w1605 w1634 w1659 w1684 w1724 w1759 w1786 w1817 w1839 w1856 w1875 w1894 w1930 w1973 w1997 w2025 w2049 w2066 w2085 w2104 w2137 w2186 w2218 w2243 w2273 w2301 w2326 w2354 w2373 w2397 w2425 w2444 w2468 w2485 w2497 w2554 w2578 w2599 w2624 w2641 w2662 w2683 w2704 w2717 w2754 w2774 w2785 w2820 w2846]
            tunnel: [w1098 w1118 w1137 w1159 w1218 w1275 w1350 w1402 w1446 w1469 w1495 w1526 w1551 w1571 w1597 w1630 w1652 w1679 w1725 w1745 w1788 w1818 w1837 w1857 w1876 w1895 w1937 w1970 w1998 w2028 w2048 w2067 w2086 w2105 w2138 w2160 w2219 w2240 w2274 w2304 w2327 w2355 w2374 w2398 w2427 w2445 w2457 w2481 w2498 w2533 w2579 w2598 w2623 w2642 w2663 w2684 w2705 w2716 w2746 w2765 w2789 w2821 w2838] -> w1046
            tunnel: [w1097 w1117 w1136 w1195 w1239 w1291 w1348 w1400 w1444 w1462 w1512 w1540 w1560 w1581 w1605 w1634 w1659 w1684 w1724 w1759 w1786 w1817 w1839 w1856 w1875 w1894 w1930 w1973 w1997 w2025 w2049 w2066 w2085 w2104 w2137 w2186 w2218 w2243 w2273 w2301 w2326 w2354 w2373 w2397 w2425 w2444 w2468 w2485 w2497 w2554 w2578 w2599 w2624 w2641 w2662 w2683 w2704 w2717 w2754 w2774 w2788 w2820 w2846] -> w1061
            tunnel: [_ _ _ _ _ _ _ _ _ _ _ _ _ _ _ _ _ _ _ _ _ _ _ _ _ _ _ _ _ _ _ _ _ _ _ _ _ w2233 _ _ _ _ _ _ _ _ _ _ _ _ _ _ _ _ _ _ _ _ _ _ _ _ _] -> w1021
            tunnel: [_ _ _ _ _ _ _ _ _ _ _ _ _ _ _ _ _ _ _ _ _ _ _ _ _ _ _ _ _ _ _ _ _ _ _ _ _ w2234 _ _ _ _ _ _ _ _ _ _ _ _ _ _ _ _ _ _ _ _ _ _ _ _ _] -> w1023
            tunnel: w1060 -> [w1095 w1115 w1134 w1161 w1220 w1297 w1349 w1401 w1445 w1467 w1513 w1538 w1553 w1579 w1617 w1644 w1649 w1676 w1723 w1758 w1783 w1813 w1838 w1854 w1873 w1892 w1936 w1972 w1996 w2023 w2045 w2064 w2083 w2102 w2136 w2182 w2210 w2242 w2254 w2298 w2323 w2351 w2371 w2396 w2424 w2442 w2460 w2487 w2525 w2546 w2576 w2601 w2626 w2639 w2660 w2681 w2702 w2726 w2740 w2767 w2795 w2814 w2840]
            tunnel: [w1095 w1115 w1134 w1161 w1220 w1297 w1349 w1401 w1445 w1467 w1513 w1538 w1550 w1579 w1617 w1644 w1649 w1676 w1723 w1758 w1783 w1813 w1838 w1854 w1873 w1892 w1936 w1972 w1996 w2023 w2045 w2064 w2083 w2102 w2136 w2182 w2210 w2242 w2253 w2298 w2323 w2351 w2371 w2396 w2424 w2442 w2459 w2487 w2525 w2546 w2576 w2601 w2626 w2639 w2660 w2681 w2702 w2726 w2740 w2767 w2795 w2814 w2840] -> w1059
            tunnel: w1058 -> [w1096 w1116 w1135 w1160 w1219 w1298 w1346 w1398 w1442 w1468 w1514 w1539 w1559 w1580 w1594 w1645 w1657 w1682 w1720 w1740 w1784 w1814 w1835 w1855 w1874 w1893 w1935 w1950 w1995 w2024 w2046 w2065 w2084 w2103 w2134 w2183 w2211 w2237 w2271 w2299 w2322 w2353 w2372 w2393 w2422 w2443 w2467 w2486 w2526 w2553 w2577 w2600 w2625 w2640 w2661 w2682 w2703 w2727 w2753 w2773 w2801 w2812 w2845]
            tunnel: [w1096 w1116 w1135 w1160 w1219 w1298 w1347 w1399 w1443 w1468 w1514 w1539 w1559 w1580 w1594 w1645 w1657 w1682 w1720 w1740 w1784 w1814 w1835 w1855 w1874 w1893 w1935 w1950 w1995 w2024 w2046 w2065 w2084 w2103 w2134 w2183 w2211 w2237 w2271 w2299 w2322 w2353 w2372 w2393 w2422 w2443 w2467 w2486 w2526 w2553 w2577 w2600 w2625 w2640 w2661 w2682 w2703 w2727 w2753 w2773 w2801 w2812 w2845] -> w1057
            tunnel: w1056 -> [_ _ _ _ _ _ _ _ _ _ _ _ _ _ _ _ _ _ w1705 w1739 w1768 w1802 _ _ _ _ _ w1943 w1977 w2011 _ _ _ _ _ _ _ w2236 _ _ _ w2352 _ _ w2423 _ _ _ _ _ _ _ _ _ _ _ _ _ _ _ _ _ _]
            tunnel: [_ _ _ _ _ _ _ _ _ _ _ _ _ _ _ _ _ _ _ _ _ _ _ _ _ _ _ _ _ _ _ _ _ _ _ _ _ _ _ _ _ _ _ _ _ _ _ _ _ _ TRUE _ _ _ _ _ _ _ _ _ _ _ _] -> w1053
            tunnel: w1042 -> [w1093 w1113 w1132 w1151 w1213 w1286 w1333 w1385 w1414 _ w1504 w1534 w1558 w1578 w1616 w1643 w1668 w1693 w1719 w1757 w1781 w1812 w1833 w1852 w1871 w1890 w1934 w1967 w1993 w2022 w2043 w2062 w2081 w2100 w2133 w2181 w2200 w2232 w2269 w2297 w2320 w2350 w2370 w2391 w2421 w2441 w2465 w2491 w2524 w2550 w2574 w2592 w2619 w2637 w2658 w2679 w2700 w2724 w2751 w2771 w2799 w2818 w2844]
            tunnel: w1041 -> [w1092 w1112 w1131 w1150 w1212 w1285 w1332 w1384 w1415 _ w1503 w1533 w1557 w1577 w1615 w1642 w1667 w1692 w1718 w1756 w1780 w1811 w1832 w1851 w1870 w1889 w1933 w1966 w1992 w2021 w2042 w2061 w2080 w2099 w2132 w2180 w2199 w2231 w2268 w2296 w2319 w2349 w2369 w2390 w2420 w2440 w2464 w2490 w2523 w2549 w2573 w2591 w2618 w2636 w2657 w2678 w2699 w2723 w2750 w2770 w2798 w2817 w2843]
            tunnel: w1040 -> [w1091 w1111 w1130 w1149 w1211 w1284 w1331 w1383 w1416 _ w1502 w1532 w1556 w1576 w1614 w1641 w1666 w1691 w1717 w1755 w1779 w1810 w1831 w1850 w1869 w1888 w1932 w1965 w1991 w2020 w2041 w2060 w2079 w2098 w2131 w2179 w2198 w2230 w2267 w2295 w2318 w2348 w2368 w2389 w2419 w2439 w2463 w2489 w2522 w2548 w2572 w2590 w2617 w2635 w2656 w2677 w2698 w2722 w2749 w2769 w2797 w2816 w2842]
            tunnel: w1039 -> [w1090 w1110 w1129 w1148 w1210 w1283 w1330 w1382 w1417 _ w1501 w1531 w1555 w1575 w1613 w1640 w1665 w1690 w1716 w1754 w1778 w1809 w1830 w1849 w1868 w1887 w1931 w1964 w1990 w2019 w2040 w2059 w2078 w2097 w2130 w2178 w2197 w2229 w2266 w2294 w2317 w2347 w2367 w2388 w2418 w2438 w2462 w2488 w2521 w2547 w2571 w2589 w2616 w2634 w2655 w2676 w2697 w2721 w2748 w2768 w2796 w2815 w2841]
            tunnel: w1038 -> [_ _ _ _ _ _ _ _ _ _ _ _ _ _ _ _ _ _ _ _ _ _ _ _ _ _ _ w1969 _ _ _ _ _ _ _ _ _ _ _ _ _ _ _ _ _ _ _ _ _ _ _ _ _ _ _ _ _ _ _ _ _ _ _]
            tunnel: w1037 -> [_ _ _ _ _ _ _ _ _ _ _ _ _ _ _ _ _ _ _ _ _ _ _ _ _ _ _ w1968 _ _ _ _ _ _ _ _ _ _ _ _ _ _ _ _ _ _ _ _ _ _ _ _ _ _ _ _ _ _ _ _ _ _ _]
            tunnel: [w1093 w1113 w1132 w1151 w1213 w1286 w1333 w1385 w1414 w1461 w1504 w1534 w1558 w1578 w1616 w1643 w1668 w1693 w1719 w1757 w1781 w1812 w1833 w1852 w1871 w1890 w1934 w1967 w1993 w2022 w2043 w2062 w2081 w2100 w2133 w2181 w2200 w2232 w2269 w2297 w2320 w2350 w2370 w2391 w2421 w2441 w2465 w2491 w2524 w2550 w2574 w2592 w2619 w2637 w2658 w2679 w2700 w2724 w2751 w2771 w2799 w2818 w2844] -> w1034
            tunnel: [w1092 w1112 w1131 w1150 w1212 w1285 w1332 w1384 w1415 w1460 w1503 w1533 w1557 w1577 w1615 w1642 w1667 w1692 w1718 w1756 w1780 w1811 w1832 w1851 w1870 w1889 w1933 w1966 w1992 w2021 w2042 w2061 w2080 w2099 w2132 w2180 w2199 w2231 w2268 w2296 w2319 w2349 w2369 w2390 w2420 w2440 w2464 w2490 w2523 w2549 w2573 w2591 w2618 w2636 w2657 w2678 w2699 w2723 w2750 w2770 w2798 w2817 w2843] -> w1002
            tunnel: [w1091 w1111 w1130 w1149 w1211 w1284 w1331 w1383 w1416 w1459 w1502 w1532 w1556 w1576 w1614 w1641 w1666 w1691 w1717 w1755 w1779 w1810 w1831 w1850 w1869 w1888 w1932 w1965 w1991 w2020 w2041 w2060 w2079 w2098 w2131 w2179 w2198 w2230 w2267 w2295 w2318 w2348 w2368 w2389 w2419 w2439 w2463 w2489 w2522 w2548 w2572 w2590 w2617 w2635 w2656 w2677 w2698 w2722 w2749 w2769 w2797 w2816 w2842] -> w1035
            tunnel: [w1090 w1110 w1129 w1148 w1210 w1283 w1330 w1382 w1417 w1458 w1501 w1531 w1555 w1575 w1613 w1640 w1665 w1690 w1716 w1754 w1778 w1809 w1830 w1849 w1868 w1887 w1931 w1964 w1990 w2019 w2040 w2059 w2078 w2097 w2130 w2178 w2197 w2229 w2266 w2294 w2317 w2347 w2367 w2388 w2418 w2438 w2462 w2488 w2521 w2547 w2571 w2589 w2616 w2634 w2655 w2676 w2697 w2721 w2748 w2768 w2796 w2815 w2841] -> w1036
            tunnel: [_ _ _ _ _ _ _ _ _ _ _ _ _ _ _ _ _ _ _ _ _ _ _ _ _ _ w1921 w1969 _ _ _ _ _ _ _ _ _ _ _ _ _ _ _ _ _ _ _ _ _ _ _ _ _ _ _ _ _ _ _ _ _ _ _] -> w1004
            tunnel: [_ _ _ _ _ _ _ _ _ _ _ _ _ _ _ _ _ _ _ _ _ _ _ _ _ _ w1920 w1968 _ _ _ _ _ _ _ _ _ _ _ _ _ _ _ _ _ _ _ _ _ _ _ _ _ _ _ _ _ _ _ _ _ _ _] -> w1003
            tunnel: w1017 -> [w1089 w1109 w1128 w1147 w1209 w1282 w1329 w1381 w1413 w1457 w1511 w1530 w1554 w1574 w1599 w1632 w1651 w1678 w1715 w1753 w1777 w1808 w1829 w1848 w1867 w1886 w1919 w1963 w1989 w2018 w2039 w2058 w2077 w2096 w2129 w2177 w2194 w2228 w2265 w2293 w2314 w2341 w2366 w2385 w2412 w2437 w2456 w2484 w2514 w2545 w2570 w2602 w2627 w2638 w2659 w2680 w2701 w2725 w2752 w2772 w2800 w2819 w2835]
            tunnel: [w1089 w1109 w1128 w1147 w1209 w1282 w1329 w1381 w1413 w1457 w1511 w1530 w1554 w1574 w1598 w1631 w1650 w1677 w1715 w1753 w1777 w1808 w1829 w1848 w1867 w1886 w1919 w1963 w1989 w2018 w2039 w2058 w2077 w2096 w2129 w2177 w2194 w2228 w2265 w2293 w2314 w2341 w2366 w2385 w2412 w2437 w2456 w2483 w2514 w2545 w2570 w2602 w2627 w2638 w2659 w2680 w2701 w2725 w2752 w2772 w2800 w2819 w2835] -> w1016
            tunnel: [w1088 w1108 w1127 w1146 w1208 w1281 w1328 w1380 w1412 w1456 w1510 w1529 w1565 w1573 w1619 w1639 w1664 w1689 w1714 w1752 w1776 w1807 w1828 w1847 w1866 w1885 w1918 w1962 w1988 w2017 w2038 w2057 w2076 w2095 w2128 w2176 w2193 w2227 w2264 w2292 w2313 w2340 w2365 w2384 w2411 w2436 w2455 w2476 w2520 w2544 w2568 w2603 w2613 w2633 w2654 w2675 w2696 w2720 w2756 w2776 w2803 w2823 w2848] -> w1015
            tunnel: [w1087 w1107 w1126 w1145 w1207 w1280 w1327 w1379 w1411 w1455 w1509 w1528 w1564 w1572 w1618 w1638 w1663 w1688 w1713 w1751 w1775 w1806 w1827 w1846 w1865 w1884 w1917 w1961 w1987 w2016 w2037 w2056 w2075 w2094 w2127 w2175 w2192 w2226 w2263 w2291 w2312 w2339 w2364 w2383 w2410 w2435 w2454 w2475 w2519 w2543 w2569 w2585 w2610 w2643 w2664 w2685 w2706 w2728 w2755 w2775 w2802 w2822 w2847] -> w1014
            tunnel: w1013 -> [w1088 w1108 w1127 w1146 w1208 w1281 w1328 w1380 w1412 w1456 w1510 w1529 w1565 w1573 w1619 w1639 w1664 w1689 w1714 w1752 w1776 w1807 w1828 w1847 w1866 w1885 w1918 w1962 w1988 w2017 w2038 w2057 w2076 w2095 w2128 w2176 w2193 w2227 w2264 w2292 w2313 w2340 w2365 w2384 w2411 w2436 w2455 w2476 w2520 w2544 w2568 _ w2613 w2633 w2654 w2675 w2696 w2720 w2756 w2776 w2803 w2823 w2848]
            tunnel: w1012 -> [w1087 w1107 w1126 w1145 w1207 w1280 w1327 w1379 w1411 w1455 w1509 w1528 w1564 w1572 w1618 w1638 w1663 w1688 w1713 w1751 w1775 w1806 w1827 w1846 w1865 w1884 w1917 w1961 w1987 w2016 w2037 w2056 w2075 w2094 w2127 w2175 w2192 w2226 w2263 w2291 w2312 w2339 w2364 w2383 w2410 w2435 w2454 w2475 w2519 w2543 w2569 _ w2610 w2643 w2664 w2685 w2706 w2728 w2755 w2775 w2802 w2822 w2847]
            tunnel: w1011 -> [_ _ _ _ _ _ _ _ _ _ _ _ _ _ _ _ _ _ _ _ _ _ _ _ _ _ _ _ _ _ _ _ _ _ _ _ _ _ _ _ _ _ _ _ _ _ _ _ _ _ _ _ _ w2631 w2652 w2673 w2694 w2718 _ _ _ _ _]
            tunnel: w1009 -> [_ _ _ _ _ _ _ _ _ _ _ _ _ _ _ _ _ w1673 w1702 w1737 w1769 w1798 _ _ _ _ _ _ _ _ _ _ _ _ _ _ _ _ _ _ _ _ _ _ _ _ _ _ _ _ _ _ _ _ _ _ _ _ _ _ _ _ _]
            tunnel: [_ "A6" _ _ _ _ _ _ _ _ _ _ _ _ _ _ _ _ _ _ _ _ _ _ _ _ _ _ _ _ _ _ _ _ _ _ _ _ _ _ _ _ _ _ _ _ _ _ _ _ _ _ _ _ _ _ _ _ _ _ _ _ _] -> w992
            tunnel: w1006 -> [_ _ _ _ _ _ _ _ _ _ _ _ _ _ _ _ _ _ _ _ _ _ _ _ _ _ _ _ _ _ _ _ _ _ _ _ _ _ _ _ _ _ _ _ _ _ _ _ _ _ _ _ _ _ _ _ _ _ _ _ w2790 _ _]
            tunnel: [w1086 w1105 w1125 w1144 w1206 w1279 w1326 w1378 w1410 w1454 w1508 w1523 w1548 w1568 w1620 w1637 w1662 w1687 w1712 w1750 w1774 w1805 w1826 w1845 w1864 w1883 w1916 w1960 w1986 w2015 w2036 w2055 w2074 w2093 w2123 w2174 w2191 w2225 w2248 w2290 w2311 w2338 w2363 w2382 w2409 w2434 w2453 w2474 w2517 w2530 w2567 w2588 w2612 w2630 w2651 w2672 w2693 w2715 w2735 w2764 w2784 w2811 w2831] -> w1000
            tunnel: w1001 -> [w1086 w1105 w1125 w1144 w1206 w1279 w1326 w1378 w1410 w1454 w1508 w1523 _ w1568 w1620 w1637 w1662 w1687 w1712 w1750 w1774 w1805 w1826 w1845 w1864 w1883 w1916 w1960 w1986 w2015 w2036 w2055 w2074 w2093 w2123 w2174 w2191 w2225 w2248 w2290 w2311 w2338 w2363 w2382 w2409 w2434 w2453 w2474 w2517 w2531 w2567 w2588 w2612 w2630 w2651 w2672 w2693 w2715 w2735 w2764 w2784 w2811 w2831]
            tunnel: w999 -> [w1085 w1104 w1124 w1143 w1205 w1278 w1325 w1377 w1409 w1453 w1507 w1522 w1547 w1567 w1612 w1636 w1661 w1686 w1711 w1749 w1773 w1804 w1825 w1844 w1863 w1882 w1915 w1959 w1985 w2014 w2035 w2054 w2073 w2092 w2122 w2173 w2190 w2224 w2262 w2289 w2310 w2337 w2362 w2381 w2408 w2433 w2452 w2473 w2516 w2542 w2566 w2587 w2615 w2629 w2650 w2671 w2692 w2714 w2734 w2763 w2783 w2810 w2830]
            tunnel: w998 -> [w1084 w1103 w1123 w1142 w1204 w1277 w1324 w1376 w1408 w1452 w1506 w1521 w1546 w1566 w1611 w1635 w1660 w1685 w1710 w1748 w1772 w1803 w1824 w1843 w1862 w1881 w1914 w1958 w1984 w2013 w2034 w2053 w2072 w2091 w2121 w2172 w2189 w2223 w2259 w2288 w2309 w2336 w2361 w2380 w2407 w2432 w2451 w2472 w2515 w2541 w2565 w2586 w2614 w2628 w2649 w2670 w2691 w2713 w2733 w2762 w2782 w2809 w2829]
            tunnel: [w1085 w1104 w1124 w1143 w1205 w1278 w1325 w1377 w1409 w1453 w1507 w1522 w1547 w1567 w1612 w1636 w1661 w1686 w1711 w1749 w1773 w1804 w1825 w1844 w1863 w1882 w1915 w1959 w1985 w2014 w2035 w2054 w2073 w2092 w2122 w2173 w2190 w2224 w2261 w2289 w2310 w2337 w2362 w2381 w2408 w2433 w2452 w2473 w2516 w2542 w2566 w2587 w2615 w2629 w2650 w2671 w2692 w2714 w2734 w2763 w2783 w2810 w2830] -> w997
            tunnel: [w1084 w1103 w1123 w1142 w1204 w1277 w1324 w1376 w1408 w1452 w1506 w1521 w1546 w1566 w1611 w1635 w1660 w1685 w1710 w1748 w1772 w1803 w1824 w1843 w1862 w1881 w1914 w1958 w1984 w2013 w2034 w2053 w2072 w2091 w2121 w2172 w2189 w2223 w2260 w2288 w2309 w2336 w2361 w2380 w2407 w2432 w2451 w2472 w2515 w2541 w2565 w2586 w2614 w2628 w2649 w2670 w2691 w2713 w2733 w2762 w2782 w2809 w2829] -> w996
            tunnel: w995 -> [_ _ _ _ _ _ _ _ _ _ w1497 _ _ _ w1623 _ _ _ _ _ _ _ _ _ _ _ _ w1955 _ _ _ _ _ _ w2119 w2171 _ _ _ _ _ _ _ _ _ _ _ _ _ _ _ _ _ _ _ _ _ _ _ _ _ _ _]
            tunnel: w994 -> [_ _ _ _ _ _ _ _ _ _ w1498 _ _ _ w1622 _ _ _ _ _ _ _ _ _ _ _ _ w1954 _ _ _ _ _ _ w2120 w2170 _ _ _ _ _ _ _ _ _ _ _ _ _ _ _ _ _ _ _ _ _ _ _ _ _ _ _]
            tunnel: w991 -> [_ _ _ _ _ _ _ _ _ _ _ _ _ _ _ _ _ w1672 w1701 w1736 w1767 w1799 _ _ _ _ _ _ _ _ _ _ _ _ _ _ _ _ _ _ _ _ _ _ _ _ _ _ _ _ _ _ _ _ _ _ _ _ _ _ _ _ _]
            tunnel: [_ _ _ _ _ _ _ _ _ _ _ _ _ _ _ _ _ _ w1705 w1738 w1768 w1802 _ _ _ _ TRUE w1943 w1977 w2011 _ _ _ _ _ _ _ _ _ _ _ _ _ _ _ _ _ _ _ _ _ _ _ _ _ _ _ _ _ _ _ _ _] -> w990
            tunnel: w989 -> [_ _ _ _ _ _ _ _ _ _ _ _ _ _ _ _ _ _ w1704 w1743 w1771 w1800 _ _ _ _ w1906 w1949 w1982 w2010 _ _ _ _ _ _ _ _ _ _ _ _ _ _ _ _ _ _ _ _ _ _ _ _ _ _ _ _ _ _ _ _ _]
            tunnel: w988 -> [_ _ _ _ _ _ _ _ _ _ _ _ _ _ _ _ _ _ w1703 w1742 w1770 w1801 _ _ _ _ w1905 w1948 w1981 w2009 _ _ _ _ _ _ _ _ _ _ _ _ _ _ _ _ _ _ _ _ _ _ _ _ _ _ _ _ _ _ _ _ _]
            tunnel: [_ _ _ _ _ _ _ _ _ _ _ _ _ _ _ _ _ w1675 w1704 w1743 w1771 w1800 _ _ _ _ w1906 w1949 w1979 w2010 _ _ _ _ _ _ _ _ _ _ _ _ _ _ _ _ _ _ _ _ _ _ _ _ _ _ _ _ _ _ _ _ _] -> w987
            tunnel: [_ _ _ _ _ _ _ _ _ _ _ _ _ _ _ _ _ w1674 w1703 w1742 w1770 w1801 _ _ _ _ w1905 w1948 w1980 w2009 _ _ _ _ _ _ _ _ _ _ _ _ _ _ _ _ _ _ _ _ _ _ _ _ _ _ _ _ _ _ _ _ _] -> w986
            tunnel: [_ _ _ _ _ _ _ _ _ _ _ _ _ _ _ _ w1654 w1673 w1702 w1737 w1764 w1798 _ _ _ _ _ _ _ _ _ _ _ _ _ _ _ _ _ _ _ _ _ _ _ _ _ _ _ _ _ _ _ _ _ _ _ _ _ _ _ _ _] -> w985
            tunnel: [_ _ _ _ _ _ _ _ _ _ _ _ _ _ _ _ w1655 w1672 w1701 w1736 w1765 w1799 _ _ _ _ _ _ _ _ _ _ _ _ _ _ _ _ _ _ _ _ _ _ _ _ _ _ _ _ _ _ _ _ _ _ _ _ _ _ _ _ _] -> w984
            tunnel: [_ _ _ _ _ _ _ _ _ _ _ _ _ _ _ _ _ _ _ w1735 _ _ _ _ _ _ _ w1946 _ _ _ _ _ _ _ _ _ _ _ _ _ _ _ _ _ _ _ _ _ _ _ _ _ _ _ _ _ _ _ _ _ _ _] -> w981
            tunnel: [_ _ _ _ _ _ _ _ _ _ _ _ _ _ _ _ _ _ _ w1734 _ _ _ _ _ _ _ w1947 _ _ _ _ _ _ _ _ _ _ _ _ _ _ _ _ _ _ _ _ _ _ _ _ _ _ _ _ _ _ _ _ _ _ _] -> w983
            tunnel: w978 -> [_ _ _ _ _ _ _ _ _ _ _ _ _ _ _ _ _ _ w1700 w1733 w1763 w1797 _ _ _ _ w1901 w1945 w1978 w2012 _ _ _ _ _ _ _ _ _ _ _ _ _ _ _ _ _ _ _ _ _ _ _ _ _ _ _ _ _ _ _ _ _]
            tunnel: [_ _ _ _ _ _ _ _ _ _ _ _ _ _ _ _ _ _ w1700 w1733 w1763 w1797 _ _ _ _ w1901 w1944 w1978 w2012 _ _ _ _ _ _ _ _ _ _ _ _ _ _ _ _ _ _ _ _ _ _ _ _ _ _ _ _ _ _ _ _ _] -> w977
            frame "Start1", Default {
            }
            frame "Start2" {
            }
            frame "Start3" {
            }
            frame "saveSettings1" {
              n548 = call "myRIO_BRig_RT_dataExp_Audio_freq__L.vi"() -> ("output_Audio_freq__L"=w1171:i32)  [unwired: 11 in]
              n549 = call "myRIO_BRig_RT_dataExp_Audio_freq__R.vi"() -> ("output_Audio_freq__R"=w1168:i32)  [unwired: 11 in]
              n550 = call "myRIO_BRig_RT_dataExp_Audio_amp__L.vi"() -> ("output_Audio_amp__L"=w1165:i32)  [unwired: 11 in]
              n551 = call "myRIO_BRig_RT_dataExp_Audio_amp__R.vi"() -> ("output_Audio_amp__R"=w1163:i32)  [unwired: 11 in]
              n552 = call "myRIO_BRig_RT_dataExp_TPB_min__L.vi"() -> ("output_TPB_min__L"=w1181:i32)  [unwired: 11 in]
              n553 = call "myRIO_BRig_RT_dataExp_TPB_min__R.vi"() -> ("output_TPB_min__R"=w1179:i32)  [unwired: 11 in]
              n554 = call "myRIO_BRig_RT_dataExp_TPB_max__L.vi"() -> ("output_TPB_max__L"=w1177:i32)  [unwired: 11 in]
              n555 = call "myRIO_BRig_RT_dataExp_TPB_max__R.vi"() -> ("output_TPB_max__R"=w1175:i32)  [unwired: 11 in]
              n556 = call "myRIO_BRig_RT_dataExp_ItrialUntilReward.vi"() -> ("output_I_trialUntilReward"=w1194:i32)  [unwired: 11 in]
              n557 = call "myRIO_BRig_RT_dataExp_IblockUntilReward.vi"() -> ("output_I_blockUntilReward"=w1190:i32)  [unwired: 11 in]
              n558 = call "myRIO_BRig_RT_dataExp_CueCycles.vi"() -> ("output_CueCycles"=w1189:i32)  [unwired: 11 in]
              n559 = call "myRIO_BRig_RT_dataExp_ENL_min.vi"() -> ("output_ENL_min"=w1187:i32)  [unwired: 11 in]
              n560 = call "myRIO_BRig_RT_dataExp_ENL_max.vi"() -> ("output_ENL_max"=w1185:i32)  [unwired: 11 in]
              n561 = call "myRIO_BRig_RT_dataExp_ENL_penalty.vi"() -> ("output_ENL_penalty"=w1183:i32)  [unwired: 11 in]
              n562 = local read "Audio_Freq__L"() -> (w1172:u16)
              n563 = local read "Audio_Freq__R"() -> (w1167:u16)
              n564 = local read "Audio_Amp__L"() -> (w1164:u16)
              n565 = local read "TpB_Min_L"() -> (w1180:u16)
              n566 = local read "TpB_Min_R"() -> (w1178:u16)
              n567 = local read "TpB_Max_L"() -> (w1176:u16)
              n568 = local read "TpB_Max_R"() -> (w1174:u16)
              n569 = local read "Audio_Amp__R"() -> (w1162:u16)
              n570 = local read "TrialUntilReward"() -> (w1193:bool)
              n571 = local read "CueCycles"() -> (w1188:u16)
              n572 = local read "Tcycle_ENL_min"() -> (w1186:u16)
              n573 = local read "Tcycle_ENL_max"() -> (w1184:u16)
              n574 = local read "Tcycle_ENLPenalty"() -> (w1182:u16)
              n575 = Multiply(x=w1172, y=u16 1000) -> (x*y=w1170:u16)
              n576 = Multiply(x=w1167, y=u16 1000) -> (x*y=w1166:u16)
              n577 = Boolean To (0,1)(Boolean=w1193) -> (0, 1=w1192:i16)
              n578 = To Unsigned Word Integer(number=w1192) -> (unsigned 16bit integer=w1191:u16)
              n579 = local read "BUR_min"() -> (w1156:u16)
              n580 = local read "BUR_max"() -> (w1157:u16)
              n581 = Not Equal To 0?(x=w1156) -> (x != 0?=w1155:bool)
              n582 = Not Equal To 0?(x=w1157) -> (x != 0?=w1154:bool)
              n583 = And(x=w1155, y=w1154) -> (x .and. y?=w1153:bool)
              n584 = Boolean To (0,1)(Boolean=w1153) -> (0, 1=w1158:i16)
              n585 = To Unsigned Word Integer(number=w1158) -> (unsigned 16bit integer=w1152:u16)
              n586 = Replace Array Subset(array=w1196, new element #1=w1191, index #1=w1194, new element #2=w1152, index #2=w1190, new element #3=w1188, index #3=w1189, new element #4=w1186, index #4=w1187, new element #5=w1184, index #5=w1185, new element #6=w1182, index #6=w1183, new element #7=w1180, index #7=w1181, new element #8=w1178, index #8=w1179, new element #9=w1176, index #9=w1177, new element #10=w1174, index #10=w1175, new element #11=w1170, index #11=w1171, new element #12=w1166, index #12=w1168, new element #13=w1164, index #13=w1165, new element #14=w1162, index #14=w1163) -> (w1195:u16[])
            }
            frame "saveSettings2" {
              n587 = call "myRIO_BRig_RT_dataExp_Tcycle_RewardPost.vi"() -> ("output_Tcycle_RewardPost"=w1229:i32)  [unwired: 11 in]
              n588 = call "myRIO_BRig_RT_dataExp_Tcycle_Wrong.vi"() -> ("output_Tcycle_Wrong"=w1227:i32)  [unwired: 11 in]
              n589 = call "myRIO_BRig_RT_dataExp_Tcycle_Timeout.vi"() -> ("output_Tcycle_Timeout"=w1225:i32)  [unwired: 11 in]
              n590 = call "myRIO_BRig_RT_dataExp_Tcycle_Cue_min.vi"() -> ("output_Tcycle_Cue_min"=w1223:i32)  [unwired: 11 in]
              n591 = call "myRIO_BRig_RT_dataExp_Tcycle_Cue_max.vi"() -> ("output_Tcycle_Cue_max"=w1222:i32)  [unwired: 11 in]
              n592 = call "myRIO_BRig_RT_dataExp_Tcycle_CuePenalty.vi"() -> ("output_Tcycle_CuePenalty"=w1221:i32)  [unwired: 11 in]
              n593 = call "myRIO_BRig_RT_dataExp_nBlock.vi"() -> ("output_nBlock"=w1238:i32)  [unwired: 11 in]
              n594 = call "myRIO_BRig_RT_dataExp_nTrial.vi"() -> ("output_nTrial"=w1237:i32)  [unwired: 11 in]
              n595 = call "myRIO_BRig_RT_dataExp_runTime_seconds.vi"() -> ("output_RunTime_minutes"=w1236:i32)  [unwired: 11 in]
              n596 = call "myRIO_BRig_RT_dataExp_Tcycle_Selection.vi"() -> ("output_Tcycle_Selection"=w1235:i32)  [unwired: 11 in]
              n597 = call "myRIO_BRig_RT_dataExp_Tcycle_Reward__L.vi"() -> ("output_Tcycle_Reward__L"=w1233:i32)  [unwired: 11 in]
              n598 = call "myRIO_BRig_RT_dataExp_Tcycle_Reward__R.vi"() -> ("output_Tcycle_Reward__R"=w1231:i32)  [unwired: 11 in]
              n599 = local read "Tcycle_RewardPost"() -> (w1228:u16)
              n600 = local read "Tcycle_Wrong"() -> (w1226:u16)
              n601 = local read "Tcycle_Timeout"() -> (w1224:u16)
              n602 = local read "Tcycle_CuePenalty"() -> (w1214:u16)
              n603 = local read "Tcycle_Cue_max"() -> (w1202:u16)
              n604 = local read "Tcycle_Cue_min"() -> (w1203:u16)
              n605 = local read "Tcycle_Selection"() -> (w1234:u16)
              n606 = local read "Tcycle_Reward_L"() -> (w1232:u16)
              n607 = local read "Tcycle_Reward_R"() -> (w1230:u16)
              n608 = Replace Array Subset(array=w1240, new element #1=u16 0, index #1=w1238, new element #2=u16 0, index #2=w1237, new element #3=u16 0, index #3=w1236, new element #4=w1234, index #4=w1235, new element #5=w1232, index #5=w1233, new element #6=w1230, index #6=w1231, new element #7=w1228, index #7=w1229, new element #8=w1226, index #8=w1227, new element #9=w1224, index #9=w1225, new element #10=w1203, index #10=w1223, new element #11=w1202, index #11=w1222, new element #12=w1214, index #12=w1221) -> (w1239:u16[])
            }
            frame "saveSettings3" {
              w1249 = 100.0 ("y")
              n609 = call "myRIO_BRig_RT_dataExp_laser_Freq.vi"() -> ("output_laser_Freq"=w1273:i32)  [unwired: 11 in]
              n610 = call "myRIO_BRig_RT_dataExp_laser_Tpeak.vi"() -> ("output_laser_Tpeak"=w1268:i32)  [unwired: 11 in]
              n611 = call "myRIO_BRig_RT_dataExp_laser_Tshutter.vi"() -> ("output_laser_Tshutter"=w1263:i32)  [unwired: 11 in]
              n612 = call "myRIO_BRig_RT_dataExp_laser_f_millisec2count.vi"() -> ("output_laser_f_millisec2count"=w1258:i32)  [unwired: 11 in]
              n613 = call "myRIO_BRig_RT_dataExp_laser_Power.vi"() -> ("output_laser_Power"=w1253:i32)  [unwired: 11 in]
              n614 = call "myRIO_BRig_RT_dataExp_laser_duration.vi"() -> ("output_laser_duration"=w1247:i32)  [unwired: 11 in]
              n615 = call "myRIO_BRig_RT_dataExp_BUR_min.vi"() -> ("output_BUR_min"=w1295:i32)  [unwired: 11 in]
              n616 = call "myRIO_BRig_RT_dataExp_BUR_max.vi"() -> ("output_BUR_max"=w1293:i32)  [unwired: 11 in]
              n617 = call "myRIO_BRig_RT_dataExp_Audio_sp__L.vi"() -> ("output_Audio_sp__L"=w1290:i32)  [unwired: 11 in]
              n618 = call "myRIO_BRig_RT_dataExp_Audio_sp__R.vi"() -> ("output_Audio_sp__R"=w1289:i32)  [unwired: 11 in]
              n619 = local read "laser_Tshutter"() -> (w1260:dbl)
              n620 = local read "f_millisec2count"() -> (w1255:dbl)
              n621 = local read "laser_power"() -> (w1250:dbl)
              n622 = local read "laser_Tpeak"() -> (w1265:dbl)
              n623 = local read "laser_Freq"() -> (w1272:dbl)
              n624 = local read "sp_LeftSpout"() -> (w1288:u16)
              n625 = local read "BUR_max"() -> (w1292:u16)
              n626 = local read "sp_RightSpout"() -> (w1287:u16)
              n627 = local read "BUR_min"() -> (w1294:u16)
              n628 = Multiply(x=w1265, y=w1249) -> (x*y=w1267:dbl)
              n629 = Multiply(x=w1260, y=w1249) -> (x*y=w1262:dbl)
              n630 = Multiply(x=w1255, y=w1249) -> (x*y=w1257:dbl)
              n631 = Multiply(x=w1250, y=w1249) -> (x*y=w1252:dbl)
              n632 = Multiply(x=w1272, y=w1249) -> (x*y=w1271:dbl)
              n633 = Round To Nearest(number=w1267) -> (nearest integer value=w1266:dbl)
              n634 = Round To Nearest(number=w1262) -> (nearest integer value=w1261:dbl)
              n635 = Round To Nearest(number=w1257) -> (nearest integer value=w1256:dbl)
              n636 = Round To Nearest(number=w1252) -> (nearest integer value=w1251:dbl)
              n637 = Round To Nearest(number=w1271) -> (nearest integer value=w1270:dbl)
              n638 = To Unsigned Word Integer(number=w1266) -> (unsigned 16bit integer=w1264:u16)
              n639 = To Unsigned Word Integer(number=w1261) -> (unsigned 16bit integer=w1259:u16)
              n640 = To Unsigned Word Integer(number=w1256) -> (unsigned 16bit integer=w1254:u16)
              n641 = To Unsigned Word Integer(number=w1251) -> (unsigned 16bit integer=w1248:u16)
              n642 = To Unsigned Word Integer(number=w1270) -> (unsigned 16bit integer=w1269:u16)
              n643 = local read "laser_duration"() -> (w1246:u16)
              n644 = call "myRIO_BRig_RT_dataCurrent_LaserPulse_duration.vi"() -> ("output_LaserPulse_duration"=w1274:i32)  [unwired: 11 in]
              n645 = Replace Array Subset(array=w1296, new element #1=w1294, index #1=w1295, new element #2=w1292, index #2=w1293, new element #3=w1288, index #3=w1290, new element #4=w1287, index #4=w1289, new element #5=w1269, index #5=w1273, new element #6=w1264, index #6=w1268, new element #7=w1259, index #7=w1263, new element #8=w1254, index #8=w1258, new element #9=w1248, index #9=w1253, new element #10=w1246, index #10=w1247) -> (w1291:u16[])
              n646 = Replace Array Subset(array=w1276, new element=w1246, index=w1274) -> (w1275:u16[])
            }
            frame "saveSettings4_LC_ENL" {
              # "delayOpt"
              # "Count"
              # "Tdelay"
              # "Probability"
              # "OnOff"
              # "Block"
              # "ENL1 All"
              # "delayOpt"
              # "Count"
              # "Tdelay"
              # "Probability"
              # "OnOff"
              # "Block"
              # "ENL1 First"
              n647 = call "myRIO_BRig_RT_dataLC_ENL1_All_Block.vi"() -> ("output_ENL1_All_Block"=w1319:i32)  [unwired: 11 in]
              n648 = call "myRIO_BRig_RT_dataLC_ENL1_All_OnOff.vi"() -> ("output_ENL1_All_OnOff"=w1308:i32)  [unwired: 11 in]
              n649 = call "myRIO_BRig_RT_dataLC_ENL1_All_Probability.vi"() -> ("output_ENL1_All_Probability"=w1307:i32)  [unwired: 11 in]
              n650 = call "myRIO_BRig_RT_dataLC_ENL1_All_Tdelay.vi"() -> ("output_ENL1_All_Tdelay"=w1306:i32)  [unwired: 11 in]
              n651 = call "myRIO_BRig_RT_dataLC_ENL1_All_Count.vi"() -> ("output_ENL1_All_Count"=w1305:i32)  [unwired: 11 in]
              n652 = call "myRIO_BRig_RT_dataLC_ENL1_All_delayOpt.vi"() -> ("output_ENL1_All_delayOpt"=w1304:i32)  [unwired: 11 in]
              n653 = call "myRIO_BRig_RT_dataLC_ENL1_First_Block.vi"() -> ("output_ENL1_First_Block"=w1345:i32)  [unwired: 11 in]
              n654 = call "myRIO_BRig_RT_dataLC_ENL1_First_OnOff.vi"() -> ("output_ENL1_First_OnOff"=w1343:i32)  [unwired: 11 in]
              n655 = call "myRIO_BRig_RT_dataLC_ENL1_First_Probability.vi"() -> ("output_ENL1_First_Probability"=w1339:i32)  [unwired: 11 in]
              n656 = call "myRIO_BRig_RT_dataLC_ENL1_First_Tdelay.vi"() -> ("output_ENL1_First_Tdelay"=w1337:i32)  [unwired: 11 in]
              n657 = call "myRIO_BRig_RT_dataLC_ENL1_First_Count.vi"() -> ("output_ENL1_First_Count"=w1335:i32)  [unwired: 11 in]
              n658 = call "myRIO_BRig_RT_dataLC_ENL1_First_delayOpt.vi"() -> ("output_ENL1_First_delayOpt"=w1321:i32)  [unwired: 11 in]
              n659 = local read "LC_ENL1_First_delayOpt"() -> (w1322:bool)
              n660 = local read "LC_ENL1_First_Count"() -> (w1334:u16)
              n661 = local read "LC_ENL1_First_Probability"() -> (w1338:u16)
              n662 = local read "LC_ENL1_First_Block"() -> (w1344:u16)
              n663 = local read "LC_ENL1_First_Tdelay"() -> (w1336:u16)
              n664 = local read "LC_ENL1_First_OnOff"() -> (w1342:bool)
              n665 = local read "LC_ENL1_All_OnOff"() -> (w1315:bool)
              n666 = local read "LC_ENL1_All_Probability"() -> (w1313:u16)
              n667 = local read "LC_ENL1_All_delayOpt"() -> (w1310:bool)
              n668 = local read "LC_ENL1_All_Tdelay"() -> (w1312:u16)
              n669 = local read "LC_ENL1_All_Block"() -> (w1316:u16)
              n670 = local read "LC_ENL1_All_Count"() -> (w1311:u16)
              n671 = Boolean To (0,1)(Boolean=w1322) -> (0, 1=w1323:i16)
              n672 = Boolean To (0,1)(Boolean=w1342) -> (0, 1=w1341:i16)
              n673 = Boolean To (0,1)(Boolean=w1315) -> (0, 1=w1318:i16)
              n674 = To Unsigned Word Integer(number=w1323) -> (unsigned 16bit integer=w1320:u16)
              n675 = To Unsigned Word Integer(number=w1341) -> (unsigned 16bit integer=w1340:u16)
              n676 = Boolean To (0,1)(Boolean=w1310) -> (0, 1=w1317:i16)
              n677 = To Unsigned Word Integer(number=w1318) -> (unsigned 16bit integer=w1314:u16)
              n678 = To Unsigned Word Integer(number=w1317) -> (unsigned 16bit integer=w1309:u16)
              n679 = Replace Array Subset(array=w1346, new element #1=w1344, index #1=w1345, new element #2=w1340, index #2=w1343, new element #3=w1338, index #3=w1339, new element #4=w1336, index #4=w1337, new element #5=w1334, index #5=w1335, new element #6=w1320, index #6=w1321, new element #7=w1316, index #7=w1319, new element #8=w1314, index #8=w1308, new element #9=w1313, index #9=w1307, new element #10=w1312, index #10=w1306, new element #11=w1311, index #11=w1305, new element #12=w1309, index #12=w1304) -> (w1347:u16[])
            }
            frame "saveSettings5_LC_Cue" {
              # "delayOpt"
              # "Count"
              # "Tdelay"
              # "Probability"
              # "OnOff"
              # "Block"
              # "Cue1 All"
              # "delayOpt"
              # "Count"
              # "Tdelay"
              # "Probability"
              # "OnOff"
              # "Block"
              # "Cue1 First"
              n680 = call "myRIO_BRig_RT_dataLC_Cue1_First_delayOpt.vi"() -> ("output_Cue1_First_delayOpt"=w1374:i32)  [unwired: 11 in]
              n681 = call "myRIO_BRig_RT_dataLC_Cue1_First_Block.vi"() -> ("output_Cue1_First_Block"=w1397:i32)  [unwired: 11 in]
              n682 = call "myRIO_BRig_RT_dataLC_Cue1_First_OnOff.vi"() -> ("output_Cue1_First_OnOff"=w1395:i32)  [unwired: 11 in]
              n683 = call "myRIO_BRig_RT_dataLC_Cue1_First_Probability.vi"() -> ("output_Cue1_First_Probability"=w1391:i32)  [unwired: 11 in]
              n684 = call "myRIO_BRig_RT_dataLC_Cue1_First_Tdelay.vi"() -> ("output_Cue1_First_Tdelay"=w1389:i32)  [unwired: 11 in]
              n685 = call "myRIO_BRig_RT_dataLC_Cue1_First_Count.vi"() -> ("output_Cue1_First_Count"=w1387:i32)  [unwired: 11 in]
              n686 = call "myRIO_BRig_RT_dataLC_Cue1_All_Block.vi"() -> ("output_Cue1_All_Block"=w1371:i32)  [unwired: 11 in]
              n687 = call "myRIO_BRig_RT_dataLC_Cue1_All_OnOff.vi"() -> ("output_Cue1_All_OnOff"=w1370:i32)  [unwired: 11 in]
              n688 = call "myRIO_BRig_RT_dataLC_Cue1_All_Probability.vi"() -> ("output_Cue1_All_Probability"=w1369:i32)  [unwired: 11 in]
              n689 = call "myRIO_BRig_RT_dataLC_Cue1_All_Tdelay.vi"() -> ("output_Cue1_All_Tdelay"=w1368:i32)  [unwired: 11 in]
              n690 = call "myRIO_BRig_RT_dataLC_Cue1_All_Count.vi"() -> ("output_Cue1_All_Count"=w1367:i32)  [unwired: 11 in]
              n691 = call "myRIO_BRig_RT_dataLC_Cue1_All_delayOpt.vi"() -> ("output_Cue1_All_delayOpt"=w1366:i32)  [unwired: 11 in]
              n692 = local read "LC_Cue1_First_delayOpt"() -> (w1373:bool)
              n693 = local read "LC_Cue1_First_Count"() -> (w1386:u16)
              n694 = local read "LC_Cue1_First_Probability"() -> (w1390:u16)
              n695 = local read "LC_Cue1_First_Block"() -> (w1396:u16)
              n696 = local read "LC_Cue1_First_Tdelay"() -> (w1388:u16)
              n697 = local read "LC_Cue1_First_OnOff"() -> (w1394:bool)
              n698 = local read "LC_Cue1_All_OnOff"() -> (w1362:bool)
              n699 = local read "LC_Cue1_All_delayOpt"() -> (w1363:bool)
              n700 = local read "LC_Cue1_All_Probability"() -> (w1359:u16)
              n701 = local read "LC_Cue1_All_Tdelay"() -> (w1358:u16)
              n702 = local read "LC_Cue1_All_Count"() -> (w1357:u16)
              n703 = local read "LC_Cue1_All_Block"() -> (w1361:u16)
              n704 = Boolean To (0,1)(Boolean=w1373) -> (0, 1=w1375:i16)
              n705 = Boolean To (0,1)(Boolean=w1394) -> (0, 1=w1393:i16)
              n706 = Boolean To (0,1)(Boolean=w1362) -> (0, 1=w1365:i16)
              n707 = To Unsigned Word Integer(number=w1375) -> (unsigned 16bit integer=w1372:u16)
              n708 = To Unsigned Word Integer(number=w1393) -> (unsigned 16bit integer=w1392:u16)
              n709 = To Unsigned Word Integer(number=w1365) -> (unsigned 16bit integer=w1360:u16)
              n710 = Boolean To (0,1)(Boolean=w1363) -> (0, 1=w1364:i16)
              n711 = To Unsigned Word Integer(number=w1364) -> (unsigned 16bit integer=w1356:u16)
              n712 = Replace Array Subset(array=w1398, new element #1=w1396, index #1=w1397, new element #2=w1392, index #2=w1395, new element #3=w1390, index #3=w1391, new element #4=w1388, index #4=w1389, new element #5=w1386, index #5=w1387, new element #6=w1372, index #6=w1374, new element #7=w1361, index #7=w1371, new element #8=w1360, index #8=w1370, new element #9=w1359, index #9=w1369, new element #10=w1358, index #10=w1368, new element #11=w1357, index #11=w1367, new element #12=w1356, index #12=w1366) -> (w1399:u16[])
            }
            frame "saveSettings6_LC_Other" {
              # "Trial"
              # "Tdelay"
              # "Probability"
              # "OnOff"
              # "Block"
              # "Wrong"
              # "Trial"
              # "Tdelay"
              # "Probability"
              # "OnOff"
              # "Block"
              # "Reward"
              n713 = call "myRIO_BRig_RT_dataLC_Wrong_Block.vi"() -> ("output_Wrong_Block"=w1429:i32)  [unwired: 11 in]
              n714 = call "myRIO_BRig_RT_dataLC_Wrong_OnOff.vi"() -> ("output_Wrong_OnOff"=w1428:i32)  [unwired: 11 in]
              n715 = call "myRIO_BRig_RT_dataLC_Wrong_Probability.vi"() -> ("output_Wrong_Probability"=w1427:i32)  [unwired: 11 in]
              n716 = call "myRIO_BRig_RT_dataLC_Wrong_Tdelay.vi"() -> ("output_Wrong_Tdelay"=w1426:i32)  [unwired: 11 in]
              n717 = call "myRIO_BRig_RT_dataLC_Wrong_Trial.vi"() -> ("output_Wrong_Trial"=w1425:i32)  [unwired: 11 in]
              n718 = call "myRIO_BRig_RT_dataLC_Reward_Block.vi"() -> ("output_Reward_Block"=w1441:i32)  [unwired: 11 in]
              n719 = call "myRIO_BRig_RT_dataLC_Reward_OnOff.vi"() -> ("output_Reward_OnOff"=w1439:i32)  [unwired: 11 in]
              n720 = call "myRIO_BRig_RT_dataLC_Reward_Probability.vi"() -> ("output_Reward_Probability"=w1435:i32)  [unwired: 11 in]
              n721 = call "myRIO_BRig_RT_dataLC_Reward_Tdelay.vi"() -> ("output_Reward_Tdelay"=w1433:i32)  [unwired: 11 in]
              n722 = call "myRIO_BRig_RT_dataLC_Reward_Trial.vi"() -> ("output_Reward_Trial"=w1431:i32)  [unwired: 11 in]
              n723 = local read "LC_Wrong_OnOff"() -> (w1423:bool)
              n724 = local read "LC_Wrong_Probability"() -> (w1420:u16)
              n725 = local read "LC_Wrong_Block"() -> (w1422:u16)
              n726 = local read "LC_Wrong_Tdelay"() -> (w1419:u16)
              n727 = local read "LC_Wrong_Trial"() -> (w1418:u16)
              n728 = local read "LC_Reward_Probability"() -> (w1434:u16)
              n729 = local read "LC_Reward_Block"() -> (w1440:u16)
              n730 = local read "LC_Reward_Tdelay"() -> (w1432:u16)
              n731 = local read "LC_Reward_OnOff"() -> (w1438:bool)
              n732 = local read "LC_Reward_Trial"() -> (w1430:u16)
              n733 = Boolean To (0,1)(Boolean=w1423) -> (0, 1=w1424:i16)
              n734 = Boolean To (0,1)(Boolean=w1438) -> (0, 1=w1437:i16)
              n735 = To Unsigned Word Integer(number=w1424) -> (unsigned 16bit integer=w1421:u16)
              n736 = To Unsigned Word Integer(number=w1437) -> (unsigned 16bit integer=w1436:u16)
              n737 = Replace Array Subset(array=w1442, new element #1=w1440, index #1=w1441, new element #2=w1436, index #2=w1439, new element #3=w1434, index #3=w1435, new element #4=w1432, index #4=w1433, new element #5=w1430, index #5=w1431, new element #6=w1422, index #6=w1429, new element #7=w1421, index #7=w1428, new element #8=w1420, index #8=w1427, new element #9=w1419, index #9=w1426, new element #10=w1418, index #10=w1425) -> (w1443:u16[])
            }
            frame "setSettings_Audio" {
              # "amp_L"
              # "amp_R"
              # "freq_L"
              # "freq_R"
              n738 = call "myRIO_BRig_RT_dataExp_Audio_amp__L.vi"() -> ("output_Audio_amp__L"=w1466:i32)  [unwired: 11 in]
              n739 = call "myRIO_BRig_RT_dataExp_Audio_amp__R.vi"() -> ("output_Audio_amp__R"=w1465:i32)  [unwired: 11 in]
              n740 = call "myRIO_BRig_RT_dataExp_Audio_freq__L.vi"() -> ("output_Audio_freq__L"=w1464:i32)  [unwired: 11 in]
              n741 = call "myRIO_BRig_RT_dataExp_Audio_freq__R.vi"() -> ("output_Audio_freq__R"=w1463:i32)  [unwired: 11 in]
              n742 = Index Array(array=w1462, index #1=w1466, index #2=w1465, index #3=w1464, index #4=w1463) -> (element #1=w1461:u16, element #2=w1459:u16, element #3=w1460:u16, element #4=w1458:u16)
            }
            frame "setSettings_Laser" {
              n743 = call "myRIO_Brig_RT__covert_Voltage_to_FPGAvalue.vi"("input_voltage"="laser_power") -> ("output_PortC"=w1499:i16)  [unwired: 9 in, 1 out]
              n744 = call "myRIO_BRig_RT__calc_Tvalley.vi"("input_peakWidth"="laser_Tpeak", "input_freq"="laser_Freq") -> ("output_Tvalley"=w1479:dbl)  [unwired: 9 in]
              n745 = Multiply(x="f_millisec2count", y="laser_Tpeak") -> (x*y=w1490:dbl)
              n746 = Multiply(x="f_millisec2count", y=w1479) -> (x*y=w1487:dbl)
              n747 = Multiply(x="f_millisec2count", y="laser_Tshutter") -> (x*y=w1485:dbl)
              n748 = Round Toward +Infinity(x="f_millisec2count") -> (ceil(x): smallest int >= x=w1493:dbl)
              n749 = Round Toward +Infinity(x=w1490) -> (ceil(x): smallest int >= x=w1491:dbl)
              n750 = Round Toward +Infinity(x=w1487) -> (ceil(x): smallest int >= x=w1488:dbl)
              n751 = Round Toward +Infinity(x=w1485) -> (ceil(x): smallest int >= x=w1478:dbl)
              n752 = To Unsigned Long Integer(number=w1493) -> (unsigned 32bit integer=w1492:u32)
              n753 = To Unsigned Long Integer(number=w1491) -> (unsigned 32bit integer=w1489:u32)
              n754 = To Unsigned Long Integer(number=w1488) -> (unsigned 32bit integer=w1486:u32)
              n755 = To Unsigned Long Integer(number=w1478) -> (unsigned 32bit integer=w1482:u32)
              n756 = To Unsigned Word Integer(number=w1478) -> (unsigned 16bit integer=w1477:u16)
              n757 = xnode "Read/Write Control"("FPGA VI Reference In"=w1497, "error in"=w1498, "laser_Npeak"=w1489, "laser_Nvalley"=w1486, "f_time_select"=w1492, "AnaOut_0"=w1499, "laser_Nshutter"=w1482) -> ("error out"=→"error out":errorcluster)  [unwired: 1 out]
              n758 = Add(x="laser_duration", y=w1477) -> (x+y=w1475:u16)
              n759 = call "myRIO_BRig_RT_dataCurrent_LaserPulse_duration.vi"() -> ("output_LaserPulse_duration"=w1494:i32)  [unwired: 11 in]
              n760 = Replace Array Subset(array=w1496, new element=w1475, index=w1494) -> (w1495:u16[])
            }
            frame "initBlock" {
              n761 = call "myRIO_Brig_RT__Case_Exp_State_initBlock.vi"("input_spout"=w1543, "input_dataExp"=w1541, "input_dataCurrent"=w1542) -> ("output_spout"=w1520:enum16{"Left", "Right"}, "output_state"=w1544:T2, "output_dataExp"=w1540:u16[], "output_dataCurrent"=w1526:u16[], "output_TpB_target"=→"TpB_target":u16)  [unwired: 4 in]
              "cSpout" <- w1520
              n762 = call "myRIO_BRig_RT_dataCurrent_iBlock.vi"() -> ("output_iBlock"=w1525:i32)  [unwired: 11 in]
              n763 = Index Array(array=w1526, index=w1525) -> (element=→"iBlock":u16)
            }
            frame "initBlock2" {
              n764 = local write "nRewards_cur"(u16 0 ("nRewards_cur")) -> ()
              n765 = call "myRIO_BRig_RT__Case_Exp_State_initBlock2.vi"("input_spout"=w1552, "input_dataBlock"=w1553, "input_dataCurrent"=w1551) -> ("idxDataBlock"=w1548:i32, "output_dataBlock"=w1550:u16[][])  [unwired: 7 in]
            }
            frame "initTrial" {
              n766 = call "myRIO_Brig_RT__Case_Exp_State_initTrial.vi"("input_dataExp"=w1582, "input_dataCurrent"=w1583) -> ("output_state"=w1584:T2, "output_dataExp"=w1581:u16[], "output_dataCurrent"=w1571:u16[])  [unwired: 7 in]
              n767 = call "myRIO_BRig_RT_dataCurrent_iTrial.vi"() -> ("output_iTrial"=w1570:i32)  [unwired: 11 in]
              n768 = Index Array(array=w1571, index=w1570) -> (element=→"iTrial":u16)
            }
            frame "initTrial2" {
              w1589 = u32 10
              # "laser time"
              # "Wrong tDelay"
              # "Reward tDelay"
              # "trialUntilReward"
              n769 = call "myRIO_BRig_RT__Case_Exp_subState_LC__initTrial.vi"("input_dataTrial"=w1599, "input_spout"=w1608, "input_dataCurrent"=w1597, "input_dataLC"=w1594) -> ("output_LC_Wrong"=w1609:bool, "output_LC_led_Wrong"=w1601:bool, "output_LC_Reward"=w1610:bool, "output_LC_led_Reward"=w1600:bool, "output_dataTrial"=w1598:u16[][])  [unwired: 2 in]
              n770 = Equal?(x=w1608, y=enum16{"Left", "Right"}."Right") -> (x = y?=w1606:bool)
              n771 = call "myRIO_BRig_RT_dataExp_ItrialUntilReward.vi"() -> ("output_I_trialUntilReward"=w1604:i32)  [unwired: 11 in]
              n772 = Index Array(array=w1605, index=w1604) -> (element=w1603:u16)
              n773 = call "myRIO_BRig_RT_dataLC_Reward_Tdelay.vi"() -> ("output_Reward_Tdelay"=w1595:i32)  [unwired: 11 in]
              n774 = call "myRIO_BRig_RT_dataLC_Wrong_Tdelay.vi"() -> ("output_Wrong_Tdelay"=w1596:i32)  [unwired: 11 in]
              n775 = Not Equal To 0?(x=w1603) -> (x != 0?=w1602:bool)
              n776 = Index Array(array=w1594, index #1=w1595, index #2=w1596) -> (element #1=w1593:u16, element #2=w1592:u16)
              n777 = To Unsigned Long Integer(number=w1593) -> (unsigned 32bit integer=w1591:u32)
              n778 = To Unsigned Long Integer(number=w1592) -> (unsigned 32bit integer=w1590:u32)
              n779 = xnode "Read/Write Control"("FPGA VI Reference In"=w1623, "error in"=w1622, "SelectionState"=FALSE, "laserResponse_reward"=w1610, "laserResponse_wrong"=w1609, "laserResponse_reward_LED"=w1600, "laserResponse_wrong_LED"=w1601, "Left(F)_or_Right(T)"=w1606, "ignoreWrong"=w1602, "tCycle_laser_rew"=w1589, "tDelay_laser_rew"=w1591, "tCycle_laser_wro"=w1589, "tDelay_laser_wro"=w1590) -> ("error out"=→"error_initTrial":errorcluster)  [unwired: 1 out]
            }
            frame "initTrial3" {
              n780 = call "myRIO_BRig_RT__Case_Exp_State_initTrial_dataTrial.vi"("input_spout"=w1629, "input_dataCurrent"=w1630, "input_dataTrial"=w1632) -> ("output_dataTrial"=w1631:u16[][])  [unwired: 8 in]
            }
            frame "initTrial_LC_ENL1" {
              n781 = call "myRIO_BRig_RT__Case_Exp_State_initTrial_LC_ENL1.vi"("input_dataTrial"=w1651, "input_spout"=w1656, "input_dataBlock"=w1649, "input_dataLC"=w1657, "input_dataCurrent"=w1653) -> ("output_LC__ENL1"=w1655:bool, "output_LC_led__ENL1"=w1654:bool, "output_dataTrial"=w1650:u16[][], "output_dataCurrent"=w1652:u16[])  [unwired: 3 in]
            }
            frame "initTrial_LC_Cue1" {
              n782 = call "myRIO_BRig_RT__Case_Exp_State_initTrial_LC_Cue1.vi"("input_dataTrial"=w1678, "input_spout"=w1681, "input_dataBlock"=w1676, "input_dataLC"=w1682, "input_dataCurrent"=w1680) -> ("output_LC__Cue1"=w1674:bool, "output_LC_led__Cue1"=w1675:bool, "output_dataTrial"=w1677:u16[][], "output_dataCurrent"=w1679:u16[])  [unwired: 3 in]
            }
            frame "ENL1_pre" {
              # "ENL1_n"
              # "Tcycle"
              # "counter"
              n783 = call "myRIO_BRig_RT_dataCurrent_Tcycle_generic.vi"() -> ("output_Tcycle_generic"=w1728:i32)  [unwired: 11 in]
              n784 = call "myRIO_BRig_RT_dataCurrent_count_generic.vi"() -> ("output_count_generic"=w1730:i32)  [unwired: 11 in]
              n785 = call "myRIO_BRig_RT_dataCurrent_ENL.vi"() -> ("output_ENL"=w1727:i32)  [unwired: 11 in]
              n786 = call "myRIO_BRig_RT_dataCurrent_ENL1_n.vi"() -> ("output_ENL1_n"=w1699:i32)  [unwired: 11 in]
              n787 = Index Array(array=w1721, index #1=w1727, index #2=w1699) -> (element #1=w1726:u16, element #2=w1698:u16)
              n788 = Increment(x=w1698) -> (x+1=w1697:u16)
              n789 = Replace Array Subset(array=w1721, new element #1=u16 0 ("new element/subarray"), index #1=w1730, new element #2=w1726, index #2=w1728, new element #3=w1697, index #3=w1699) -> (w1725:u16[])
              n790 = Select(t=myRIO_BRig_RT__Case_Exp_stateList."ENL1Penalty_pre" ("Enum"), s=w1709, f=myRIO_BRig_RT__Case_Exp_stateList."ENL1" ("Enum")) -> (s? t:f=w1706:T2)
            }
            frame "ENL1" {
              n791 = call "myRIO_BRig_RT__Case_Exp_State_ENL1.vi"("input_LC"=w1736, "I_lick"=w1741, "input_LC_led"=w1737, "input_state"=w1747, "input_dataCurrent"=w1746) -> ("output_trigger_laser_led"=w1735:bool, "output_state"=w1744:T2, "output_dataCurrent"=w1745:u16[], "output_trigger_laser"=w1734:bool)  [unwired: 3 in]
              n792 = Or(x=w1735, y=w1739) -> (x .or. y?=w1738:bool)
            }
            frame "ENL1Penalty_pre" {
              w1766 = FALSE
              # "Tcycle"
              # "counter"
              n793 = call "myRIO_BRig_RT_dataCurrent_Tcycle_generic.vi"() -> ("output_Tcycle_generic"=w1790:i32)  [unwired: 11 in]
              n794 = call "myRIO_BRig_RT_dataCurrent_count_generic.vi"() -> ("output_count_generic"=w1792:i32)  [unwired: 11 in]
              n795 = Select(t=w1766, s=w1768, f=w1769) -> (s? t:f=w1764:bool)
              n796 = Select(t=w1766, s=w1768, f=w1767) -> (s? t:f=w1765:bool)
              n797 = call "myRIO_BRig_RT_dataExp_ENL_penalty.vi"() -> ("output_ENL_penalty"=w1785:i32)  [unwired: 11 in]
              n798 = Index Array(array=w1786, index=w1785) -> (element=w1789:u16)
              n799 = Replace Array Subset(array=w1787, new element #1=u16 0 ("new element/subarray"), index #1=w1792, new element #2=w1789, index #2=w1790) -> (w1788:u16[])
            }
            frame "ENL1Penalty" {
              n800 = call "myRIO_BRig_RT__Case_Exp_State_ENL1Penalty.vi"("input_state"=w1815, "input_dataCurrent"=w1819) -> ("output_state"=w1816:T2, "output_dataCurrent"=w1818:u16[])  [unwired: 8 in]
            }
            frame "ENL2_pre" {
            }
            frame "ENL2" {
            }
            frame "ENL2Penalty_pre" {
            }
            frame "ENL2Penalty" {
            }
            frame "Cue1_pre" {
              # "Cue1_n"
              # "Tcycle_Cue1"
              # "0 = L, 1 = R, 2 = both"
              # "sp_R"
              # "sp_L"
              # "Tcycle"
              # "counter"
              n801 = Equal?(x=w1928, y=enum16{"Left", "Right"}."Left") -> (x = y?=w1927:bool)
              n802 = call "myRIO_BRig_RT_dataExp_Audio_sp__L.vi"() -> ("output_Audio_sp__L"=w1926:i32)  [unwired: 11 in]
              n803 = call "myRIO_BRig_RT_dataExp_Audio_sp__R.vi"() -> ("output_Audio_sp__R"=w1925:i32)  [unwired: 11 in]
              n804 = call "myRIO_BRig_RT_dataCurrent_Tcycle_generic.vi"() -> ("output_Tcycle_generic"=w1938:i32)  [unwired: 11 in]
              n805 = call "myRIO_BRig_RT_dataCurrent_count_generic.vi"() -> ("output_count_generic"=w1940:i32)  [unwired: 11 in]
              n806 = Select(t=w1926, s=w1927, f=w1925) -> (s? t:f=w1924:i32)
              n807 = call "myRIO_BRig_RT_dataCurrent_Cue1_n.vi"() -> ("output_Cue1_n"=w1902:i32)  [unwired: 11 in]
              n808 = call "myRIO_BRig_RT_dataCurrent_Tcycle_cue.vi"() -> ("output_Tcycle_cue"=w1911:i32)  [unwired: 11 in]
              n809 = Index Array(array=w1930, index=w1924) -> (element=w1922:u16)
              n810 = Index Array(array=w1912, index #1=w1911, index #2=w1902) -> (element #1=w1913:u16, element #2=w1904:u16)
              n811 = Increment(x=w1904) -> (x+1=w1903:u16)
              n812 = Not Equal To 0?(x=w1922) -> (x != 0?=w1920:bool)
              n813 = Not Equal?(x=w1922, y=u16 1) -> (x != y?=w1921:bool)
              n814 = Replace Array Subset(array=w1912, new element #1=u16 0 ("new element/subarray"), index #1=w1940, new element #2=w1913, index #2=w1938, new element #3=w1903, index #3=w1902) -> (w1937:u16[])
              n815 = Select(t=myRIO_BRig_RT__Case_Exp_stateList."Cue1Penalty_pre" ("Enum"), s=w1908, f=myRIO_BRig_RT__Case_Exp_stateList."Cue1" ("Enum")) -> (s? t:f=w1909:T2)
            }
            frame "Cue1" {
              n816 = call "myRIO_BRig_RT__Case_Exp_State_Cue1.vi"("input_LC"=w1948, "I_lick"=w1951, "input_LC_led"=w1949, "input_state"=w1953, "input_dataCurrent"=w1971) -> ("output_trigger_laser_led"=w1946:bool, "output_state"=w1952:T2, "output_dataCurrent"=w1970:u16[], "output_trigger_laser"=w1947:bool)  [unwired: 3 in]
              n817 = Or(x=w1946, y=w1945) -> (x .or. y?=w1944:bool)
              n818 = Equal?(x=myRIO_BRig_RT__Case_Exp_stateList."Selection_pre", y=w1952) -> (x = y?=w1956:bool)
              n819 = xnode "Read/Write Control"("FPGA VI Reference In"=w1955, "error in"=w1954, "SelectionState"=w1956) -> ()  [unwired: 2 out]
            }
            frame "Cue1Penalty_pre" {
              w1983 = FALSE
              # "Tcycle"
              # "counter"
              n820 = call "myRIO_BRig_RT_dataCurrent_Tcycle_generic.vi"() -> ("output_Tcycle_generic"=w2003:i32)  [unwired: 11 in]
              n821 = call "myRIO_BRig_RT_dataCurrent_count_generic.vi"() -> ("output_count_generic"=w2005:i32)  [unwired: 11 in]
              n822 = call "myRIO_BRig_RT_dataExp_Tcycle_CuePenalty.vi"() -> ("output_Tcycle_CuePenalty"=w2002:i32)  [unwired: 11 in]
              n823 = Select(t=w1983, s=w1978, f=w1982) -> (s? t:f=w1979:bool)
              n824 = Select(t=w1983, s=w1978, f=w1981) -> (s? t:f=w1980:bool)
              n825 = Index Array(array=w1997, index=w2002) -> (element=w2001:u16)
              n826 = Replace Array Subset(array=w1999, new element #1=u16 0 ("new element/subarray"), index #1=w2005, new element #2=w2001, index #2=w2003) -> (w1998:u16[])
            }
            frame "Cue1Penalty" {
              n827 = call "myRIO_BRig_RT__Case_Exp_State_Cue1Penalty.vi"("input_state"=w2029, "input_dataCurrent"=w2030) -> ("output_state"=w2027:T2, "output_dataCurrent"=w2028:u16[])  [unwired: 8 in]
            }
            frame "Cue2_pre" {
              n828 = call "myRIO_BRig_RT__Case_Exp_subState_LC__Cue2.vi"("input_spout"=w2047, "input_dataCurrent"=w2048, "input_dataLC"=w2046) -> ()  [unwired: 6 in, 2 out]
            }
            frame "Cue2" {
            }
            frame "Cue2Penalty_pre" {
            }
            frame "Cue2Penalty" {
            }
            frame "Selection_pre" {
              # "Tcycle"
              # "counter"
              n829 = xnode "Read/Write Control"("FPGA VI Reference In"=w2119, "error in"=w2120) -> ("error out"=→"error_Selection_pre":errorcluster, "SelectReward"=w2112:bool, "SelectWrong"=w2114:bool)  [unwired: 1 out]
              n830 = call "myRIO_BRig_RT_dataCurrent_Tcycle_generic.vi"() -> ("output_Tcycle_generic"=w2141:i32)  [unwired: 11 in]
              n831 = call "myRIO_BRig_RT_dataCurrent_count_generic.vi"() -> ("output_count_generic"=w2143:i32)  [unwired: 11 in]
              n832 = call "myRIO_BRig_RT_dataExp_Tcycle_Selection.vi"() -> ("output_Tcycle_Selection"=w2140:i32)  [unwired: 11 in]
              n833 = Index Array(array=w2137, index=w2140) -> (element=w2139:u16)
              n834 = Replace Array Subset(array=w2135, new element #1=u16 0 ("new element/subarray"), index #1=w2143, new element #2=w2139, index #2=w2141) -> (w2138:u16[])
              n835 = Or(x=w2112, y=w2114) -> (x .or. y?=w2113:bool)
              n836 = Select(t=myRIO_BRig_RT__Case_Exp_stateList."SelectReward_pre" ("Enum"), s=w2112, f=myRIO_BRig_RT__Case_Exp_stateList."SelectWrong_pre" ("Enum")) -> (s? t:f=w2118:T2)
              n837 = Select(t=w2118, s=w2113, f=myRIO_BRig_RT__Case_Exp_stateList."Selection" ("Enum")) -> (s? t:f=w2115:T2)
            }
            frame "Selection" {
              # "counter\nSelection"
              # "increment"
              # "get Tcycle"
              # "get count"
              n838 = xnode "Read/Write Control"("FPGA VI Reference In"=w2171, "error in"=w2170) -> ("FPGA VI Reference Out"=w2146:refnum<k20>, "error out"=w2147:errorcluster, "SelectReward"=w2167:bool, "SelectWrong"=w2168:bool)
              n839 = call "myRIO_BRig_RT_dataCurrent_Tcycle_generic.vi"() -> ("output_Tcycle_generic"=w2164:i32)  [unwired: 11 in]
              n840 = call "myRIO_BRig_RT_dataCurrent_count_generic.vi"() -> ("output_count_generic"=w2156:i32)  [unwired: 11 in]
              n841 = Index Array(array=w2165, index #1=w2164, index #2=w2156) -> (element #1=w2155:u16, element #2=w2163:u16)
              n842 = call "myRIO_BRig_RT__increment_u16.vi"() -> ("output_increment__u16"=w2162:u16)  [unwired: 11 in]
              n843 = Add(x=w2163, y=w2162) -> (x+y=w2157:u16)
              n844 = Greater?(x=w2155, y=w2157) -> (0:w2158:bool)
              n845 = Select(t=w2161, s=w2158, f=myRIO_BRig_RT__Case_Exp_stateList."SelectTimeout_pre" ("Enum")) -> (s? t:f=w2150:T2)
              n846 = Select(t=w2157, s=w2158, f=w2155) -> (s? t:f=w2153:u16)
              n847 = call "myRIO_BRig_RT_dataCurrent_count_selection.vi"() -> ("output_count_generic"=w2154:i32)  [unwired: 11 in]
              n848 = Select(t=myRIO_BRig_RT__Case_Exp_stateList."SelectReward_pre" ("Enum"), s=w2167, f=myRIO_BRig_RT__Case_Exp_stateList."SelectWrong_pre" ("Enum")) -> (s? t:f=w2166:T2)
              n849 = Replace Array Subset(array=w2165, new element #1=w2153, index #1=w2156, new element #2=w2153, index #2=w2154) -> (w2160:u16[])
              n850 = Or(x=w2167, y=w2168) -> (x .or. y?=w2149:bool)
              n851 = Not(x=w2149) -> (.not. x?=w2148:bool)
              n852 = xnode "Read/Write Control"("FPGA VI Reference In"=w2146, "error in"=w2147, "SelectionState"=w2148) -> ("error out"=→"error_Selection":errorcluster)  [unwired: 1 out]
              n853 = Select(t=w2166, s=w2149, f=w2150) -> (s? t:f=w2169:T2)
            }
            frame "SelectReward_pre" {
              # "iState"
              # "Tcycle\nReward"
              # "nRewTrials"
              # "Tcycle\nGeneric"
              # "counter"
              n854 = call "myRIO_BRig_RT_dataCurrent_nRewTrials.vi"() -> ("output_nRewTrials"=w2203:i32)  [unwired: 11 in]
              n855 = Equal?(x=w2212, y=enum16{"Left", "Right"}."Left") -> (x = y?=w2213:bool)
              n856 = Index Array(array=w2204, index=w2203) -> (element=w2202:u16)
              n857 = call "myRIO_BRig_RT_dataExp_Tcycle_Reward__L.vi"() -> ("output_Tcycle_Reward__L"=w2216:i32)  [unwired: 11 in]
              n858 = call "myRIO_BRig_RT_dataExp_Tcycle_Reward__R.vi"() -> ("output_Tcycle_Reward__R"=w2217:i32)  [unwired: 11 in]
              n859 = Increment(x=w2202) -> (x+1=w2201:u16)
              n860 = Select(t=w2216, s=w2213, f=w2217) -> (s? t:f=w2215:i32)
              n861 = call "myRIO_BRig_RT__Case_Exp_subState_LC__Reward.vi"("input_spout"=w2212, "input_dataCurrent"=w2204, "input_dataLC"=w2211) -> ()  [unwired: 6 in, 2 out]
              n862 = call "myRIO_BRig_RT_dataCurrent_count_generic.vi"() -> ("output_count_generic"=w2206:i32)  [unwired: 11 in]
              n863 = call "myRIO_BRig_RT_dataCurrent_Tcycle_generic.vi"() -> ("output_Tcycle_generic"=w2207:i32)  [unwired: 11 in]
              n864 = Index Array(array=w2218, index=w2215) -> (element=w2208:u16)
              n865 = call "myRIO_BRig_RT_dataCurrent_iState.vi"() -> ("output_iState"=w2196:i32)  [unwired: 11 in]
              n866 = Replace Array Subset(array=w2204, new element #1=w2201, index #1=w2203, new element #2=u16 0 ("new element/subarray"), index #2=w2206, new element #3=w2208, index #3=w2207, new element #4=u16 1 ("new element/subarray"), index #4=w2196) -> (w2219:u16[])
            }
            frame "SelectReward" {
              n867 = call "myRIO_BRig_RT__Case_Exp_State_Reward.vi"("input_dataCurrent"=w2241, "input_state"=w2238, "input_spout"=w2235, "input_LC"=w2236, "input_dataLC"=w2237) -> ("output_dataCurrent"=w2240:u16[], "output_state"=w2239:T2, "output__L"=w2233:bool, "output__R"=w2234:bool)  [unwired: 6 in, 1 out]
            }
            frame "SelectRewardPost_pre" {
              # "nRewards"
              # "nRewTrials"
              # "Tcycle"
              # "counter"
              n868 = call "myRIO_BRig_RT_dataBlock_nRewards__L.vi"() -> ("output_nRewards__L"=w2257:i32)  [unwired: 11 in]
              n869 = call "myRIO_BRig_RT_dataBlock_nRewards__R.vi"() -> ("output_nRewards__R"=w2256:i32)  [unwired: 11 in]
              n870 = call "myRIO_BRig_RT_dataCurrent_Tcycle_generic.vi"() -> ("output_Tcycle_generic"=w2276:i32)  [unwired: 11 in]
              n871 = call "myRIO_BRig_RT_dataCurrent_count_generic.vi"() -> ("output_count_generic"=w2278:i32)  [unwired: 11 in]
              n872 = case shown="\"Left\", Default" w2250 {
                tunnel: w2262 -> [w2283 w2287]
                tunnel: [w2282 w2287] -> w2261
                tunnel: [w2284 w2285] -> w2260
                tunnel: w2259 -> [w2284 w2286]
                frame "Left", Default {
                  n873 = Increment(x=w2283) -> (x+1=w2282:u16)
                }
                frame "Right" {
                  n874 = Increment(x=w2286) -> (x+1=w2285:u16)
                }
              }
              "nRewards_Left" <- w2261
              "nRewards_Right" <- w2260
              n875 = Equal?(x=w2250, y=enum16{"Left", "Right"}."Left") -> (x = y?=w2249:bool)
              n876 = Select(t=w2257, s=w2249, f=w2256) -> (s? t:f=w2255:i32)
              n877 = call "myRIO_BRig_RT_dataExp_Tcycle_RewardPost.vi"() -> ("output_Tcycle_RewardPost"=w2272:i32)  [unwired: 11 in]
              n878 = call "myRIO_BRig_RT_dataCurrent_nRewTrials.vi"() -> ("output_nRewTrials"=w2258:i32)  [unwired: 11 in]
              n879 = Index Array(array=w2273, index=w2272) -> (element=w2275:u16)
              n880 = Index Array(array=w2252, index=w2258) -> (element=w2247:u16)
              n881 = Replace Array Subset(array=w2252, new element #1=u16 0 ("new element/subarray"), index #1=w2278, new element #2=w2275, index #2=w2276) -> (w2274:u16[])
              n882 = Replace Array Subset(array=w2254, new element=w2247, index (row)=w2248, index (col)=w2255) -> (w2253:u16[][])
              n883 = local write "nRewards_cur"(w2247) -> ()
            }
            frame "SelectRewardPost" {
              n884 = call "myRIO_BRig_RT__Case_Exp_State_RewardPost.vi"("input_state"=w2302, "input_dataCurrent"=w2305) -> ("output_state"=w2303:T2, "output_dataCurrent"=w2304:u16[])  [unwired: 8 in]
            }
            frame "SelectWrong_pre" {
              # "iState"
              # "Tcycle"
              # "counter"
              n885 = call "myRIO_BRig_RT_dataCurrent_Tcycle_generic.vi"() -> ("output_Tcycle_generic"=w2330:i32)  [unwired: 11 in]
              n886 = call "myRIO_BRig_RT_dataCurrent_count_generic.vi"() -> ("output_count_generic"=w2332:i32)  [unwired: 11 in]
              n887 = call "myRIO_BRig_RT_dataExp_Tcycle_Wrong.vi"() -> ("output_Tcycle_Wrong"=w2328:i32)  [unwired: 11 in]
              n888 = call "myRIO_BRig_RT__Case_Exp_subState_LC__Wrong.vi"("input_spout"=w2324, "input_dataCurrent"=w2325, "input_dataLC"=w2322) -> ()  [unwired: 6 in, 2 out]
              n889 = Index Array(array=w2326, index=w2328) -> (element=w2329:u16)
              n890 = call "myRIO_BRig_RT_dataCurrent_iState.vi"() -> ("output_iState"=w2316:i32)  [unwired: 11 in]
              n891 = Replace Array Subset(array=w2325, new element #1=u16 0 ("new element/subarray"), index #1=w2332, new element #2=w2329, index #2=w2330, new element #3=u16 2 ("new element/subarray"), index #3=w2316) -> (w2327:u16[])
            }
            frame "SelectWrong" {
              n892 = call "myRIO_BRig_RT__Case_Exp_State_Wrong.vi"("input_dataLC"=w2353, "input_LC"=w2352, "input_state"=w2346, "input_dataCurrent"=w2356) -> ("output_state"=w2343:T2, "output_dataCurrent"=w2355:u16[])  [unwired: 5 in, 1 out]
              n893 = Not Equal?(x=w2346, y=w2343) -> (x != y?=w2345:bool)
              n894 = Select(t=myRIO_BRig_RT__Case_Exp_stateList."SelectWrong_post" ("Enum"), s=w2345, f=w2343) -> (s? t:f=w2342:T2)
            }
            frame "SelectWrong_post" {
            }
            frame "SelectTimeout_pre" {
              # "iState"
              # "Tcycle"
              # "counter"
              n895 = call "myRIO_BRig_RT_dataCurrent_Tcycle_generic.vi"() -> ("output_Tcycle_generic"=w2401:i32)  [unwired: 11 in]
              n896 = call "myRIO_BRig_RT_dataCurrent_count_generic.vi"() -> ("output_count_generic"=w2399:i32)  [unwired: 11 in]
              n897 = call "myRIO_BRig_RT_dataExp_Tcycle_Timeout.vi"() -> ("output_Tcycle_Timeout"=w2403:i32)  [unwired: 11 in]
              n898 = call "myRIO_BRig_RT__Case_Exp_subState_LC__Timeout.vi"("input_spout"=w2394, "input_dataCurrent"=w2395, "input_dataLC"=w2393) -> ()  [unwired: 6 in, 2 out]
              n899 = Index Array(array=w2397, index=w2403) -> (element=w2402:u16)
              n900 = call "myRIO_BRig_RT_dataCurrent_iState.vi"() -> ("output_iState"=w2387:i32)  [unwired: 11 in]
              n901 = Replace Array Subset(array=w2395, new element #1=u16 0 ("new element/subarray"), index #1=w2399, new element #2=w2402, index #2=w2401, new element #3=u16 3 ("new element/subarray"), index #3=w2387) -> (w2398:u16[])
            }
            frame "SelectTimeout" {
              n902 = call "myRIO_BRig_RT__Case_Exp_State_Timeout.vi"("input_dataLC"=w2422, "input_LC"=w2423, "input_state"=w2413, "input_dataCurrent"=w2428) -> ("output_state"=w2414:T2, "output_dataCurrent"=w2427:u16[])  [unwired: 5 in, 1 out]
              n903 = Not Equal?(x=w2413, y=w2414) -> (x != y?=w2417:bool)
              n904 = Select(t=myRIO_BRig_RT__Case_Exp_stateList."SelectTimeout_post" ("Enum"), s=w2417, f=w2414) -> (s? t:f=w2415:T2)
            }
            frame "SelectTimeout_post" {
            }
            frame "endTrial1" {
              # "Update dataBlock"
              n905 = call "myRIO_BRig_RT__Case_Exp_State_endTrial1.vi"("input_spout"=w2461, "input_dataBlock"=w2460, "input_dataCurrent"=w2458) -> ("output_dataBlock"=w2459:u16[][], "output_dataCurrent"=w2457:u16[])  [unwired: 7 in]
            }
            frame "endTrial2" {
              # "update dataTrial"
              n906 = call "myRIO_BRig_RT__Case_Exp_State_endTrial2.vi"("input_spout"=w2480, "input_dataTrial"=w2484, "input_dataCurrent"=w2482) -> ("output_dataTrial"=w2483:u16[][], "output_dataCurrent"=w2481:u16[])  [unwired: 7 in]
            }
            frame "endTrial3" {
              w2506 = myRIO_BRig_RT__Case_Exp_stateList."endBlock" ("Enum")
              # "nRewTrials"
              # "iTrial"
              # "I_blockUntilReward"
              # "TPB"
              # "end block?"
              n907 = local read "STOP_endTrial"() -> (w2504:bool)
              n908 = local read "STOP_abort"() -> (w2503:bool)
              n909 = local read "START"() -> (w2501:bool)
              n910 = call "myRIO_BRig_RT_dataExp_IblockUntilReward.vi"() -> ("output_I_blockUntilReward"=w2513:i32)  [unwired: 11 in]
              n911 = Index Array(array=w2497, index=w2513) -> (element=w2493:u16)
              n912 = Not(x=w2501) -> (.not. x?=w2502:bool)
              n913 = Not Equal To 0?(x=w2493) -> (x != 0?=w2511:bool)
              n914 = Compound Arithmetic op=OR(w2504, w2502, w2503) -> (w2505:bool)
              n915 = call "myRIO_BRig_RT_dataCurrent_nRewTrials.vi"() -> ("output_nRewTrials"=w2509:i32)  [unwired: 11 in]
              n916 = call "myRIO_BRig_RT_dataCurrent_iTrial.vi"() -> ("output_iTrial"=w2510:i32)  [unwired: 11 in]
              n917 = Select(t=w2509, s=w2511, f=w2510) -> (s? t:f=w2508:i32)
              n918 = call "myRIO_BRig_RT_dataCurrent_TpB.vi"() -> ("output_TpB"=w2512:i32)  [unwired: 11 in]
              n919 = Index Array(array=w2498, index #1=w2512, index #2=w2508) -> (element #1=w2499:u16, element #2=w2500:u16)
              n920 = Less Or Equal?(x=w2499, y=w2500) -> (x <= y?=w2496:bool)
              n921 = Select(t=w2506, s=w2496, f=myRIO_BRig_RT__Case_Exp_stateList."initTrial" ("Enum")) -> (s? t:f=w2507:T2)
              n922 = Select(t=w2506, s=w2505, f=w2507) -> (s? t:f=w2494:T2)
            }
            frame "endBlock" {
              # "R"
              # "L"
              # "idxDataBlock"
              n923 = Equal?(x=w2537, y=enum16{"Left", "Right"}."Left") -> (x = y?=w2536:bool)
              n924 = call "myRIO_BRig_RT_dataCurrent_idxDataBlockL.vi"() -> ("output_idxDataBlock__L"=w2540:i32)  [unwired: 11 in]
              n925 = call "myRIO_BRig_RT_dataCurrent_idxDataBlockR.vi"() -> ("output_idxDataBlock__R"=w2539:i32)  [unwired: 11 in]
              n926 = Increment(x=w2531) -> (x+1=w2530:i32)
              n927 = Select(t=w2540, s=w2536, f=w2539) -> (s? t:f=w2534:i32)
              n928 = To Unsigned Word Integer(number=w2530) -> (unsigned 16bit integer=w2532:u16)
              n929 = local read "START"() -> (w2560:bool)
              n930 = local read "STOP_endBlock"() -> (w2555:bool)
              n931 = local read "STOP_endTrial"() -> (w2558:bool)
              n932 = local read "STOP_abort"() -> (w2557:bool)
              n933 = Replace Array Subset(array=w2535, new element=w2532, index=w2534) -> (w2533:u16[])
              n934 = Not(x=w2560) -> (.not. x?=w2559:bool)
              n935 = Compound Arithmetic op=OR(w2559, w2555, w2558, w2557) -> (w2556:bool)
              n936 = Select(t=myRIO_BRig_RT__Case_Exp_stateList."endExp" ("Enum"), s=w2556, f=myRIO_BRig_RT__Case_Exp_stateList."initBlock" ("Enum")) -> (s? t:f=w2564:T2)
            }
            frame "endExp" {
            }
            frame "commConnect" {
              n937 = call "myRIO_BRig_RT_comm_webdav_connect.vi"("input_password"="Host Password", "input_username"="Host UserName") -> ("output_Iconnected"=w2585:bool, "output_hSession"=w2603:T6)  [unwired: 7 in, 1 out]
              "Connected To Host?" <- w2585
              n938 = case shown="False" w2585 {
                frame False {
                  n939 = One Button Dialog(message="Connection Failed!\nData not being saved!") -> ()  [unwired: 1 in, 1 out]
                }
                frame True {
                }
              }
            }
            frame "commUpload_pre" {
              n940 = Select(t=myRIO_BRig_RT__Case_Exp_stateList."commUpload_dataBlock" ("Enum"), s=w2610, f=myRIO_BRig_RT__Case_Exp_stateList."endTrial3") -> (s? t:f=w2608:T2)
            }
            frame "commUpload_dataBlock" {
              n941 = call "myRIO_BRig_RT_comm_webdav_uploadFile__data.vi"("input_fileName_prefix"=w2631, "input_fileName"="dataBlock" ("input_filename"), "input_hSession"=w2633) -> ()  [unwired: 8 in, 1 out]
            }
            frame "commUpload_dataCurrent" {
              n942 = call "myRIO_BRig_RT_comm_webdav_uploadFile__data.vi"("input_fileName_prefix"=w2652, "input_fileName"="dataCurrent" ("input_filename"), "input_hSession"=w2654) -> ()  [unwired: 8 in, 1 out]
            }
            frame "commUpload_dataExp" {
              n943 = call "myRIO_BRig_RT_comm_webdav_uploadFile__data.vi"("input_fileName_prefix"=w2673, "input_fileName"="dataExp" ("input_filename"), "input_hSession"=w2675) -> ()  [unwired: 8 in, 1 out]
            }
            frame "commUpload_dataLC" {
              n944 = call "myRIO_BRig_RT_comm_webdav_uploadFile__data.vi"("input_fileName_prefix"=w2694, "input_fileName"="dataLC" ("input_filename"), "input_hSession"=w2696) -> ()  [unwired: 8 in, 1 out]
            }
            frame "commUpload_dataTrial" {
              n945 = call "myRIO_BRig_RT_comm_webdav_uploadFile__data.vi"("input_fileName_prefix"=w2718, "input_fileName"="dataTrial" ("input_filename"), "input_hSession"=w2720) -> ()  [unwired: 8 in, 1 out]
            }
            frame "saveData_dataBlock" {
              # "idxDataBlockR"
              # "idxDataBlockL"
              n946 = call "myRIO_BRig_RT_dataCurrent_idxDataBlockL.vi"() -> ("output_idxDataBlock__L"=w2744:i32)  [unwired: 11 in]
              n947 = call "myRIO_BRig_RT_dataCurrent_idxDataBlockR.vi"() -> ("output_idxDataBlock__R"=w2745:i32)  [unwired: 11 in]
              n948 = Index Array(array=w2746, index #1=w2744, index #2=w2745) -> (element #1=w2743:u16, element #2=w2742:u16)
              n949 = Greater?(x=w2743, y=w2742) -> (0:w2741:bool)
              n950 = Select(t=w2743, s=w2741, f=w2742) -> (s? t:f=w2739:u16)
              n951 = Increment(x=w2739) -> (x+1=w2738:u16)
              n952 = To Long Integer(number=w2738) -> (32bit integer=w2737:i32)
              n953 = Array Subset(array=w2740, length (row)=w2737) -> (w2736:u16[][])  [unwired: 3 in]
              n954 = call "myRIO_BRig_RT_comm_webdav_saveArrayToFile__2D_u16.vi"("Array"=w2736, "input_filename"="dataBlock") -> ()  [unwired: 10 in]
            }
            frame "saveData_dataCurrent" {
              n955 = call "myRIO_BRig_RT_comm_webdav_saveArrayToFile__1D_u16.vi"("Array"=w2765, "input_filename"="dataCurrent") -> ()  [unwired: 10 in]
            }
            frame "saveData_dataExp" {
              # "runTime"
              n956 = Get Date/Time In Seconds() -> (seconds since 1Jan1904=w2793:timestamp)
              n957 = To Double Precision Float(number=w2793) -> (double precision float=w2792:dbl)
              n958 = call "myRIO_BRig_RT_dataExp_runTime_seconds.vi"() -> ("output_RunTime_minutes"=w2791:i32)  [unwired: 11 in]
              n959 = Subtract(x=w2792, y=w2790) -> (x-y=w2787:dbl)
              n960 = To Unsigned Word Integer(number=w2787) -> (unsigned 16bit integer=w2786:u16)
              n961 = Replace Array Subset(array=w2785, new element=w2786, index=w2791) -> (w2788:u16[])
              n962 = call "myRIO_BRig_RT_comm_webdav_saveArrayToFile__1D_u16.vi"("Array"=w2788, "input_filename"="dataExp") -> ()  [unwired: 10 in]
            }
            frame "saveData_dataLC" {
              n963 = call "myRIO_BRig_RT_comm_webdav_saveArrayToFile__1D_u16.vi"("Array"=w2812, "input_filename"="dataLC") -> ()  [unwired: 10 in]
            }
            frame "saveData_dataTrial" {
              # "idxTrial"
              n964 = call "myRIO_BRig_RT_dataCurrent_idxDataTrial.vi"() -> ("output_idxDataTrial"=w2837:i32)  [unwired: 11 in]
              n965 = Index Array(array=w2838, index=w2837) -> (element=w2834:u16)
              n966 = Increment(x=w2834) -> (x+1=w2833:u16)
              n967 = To Long Integer(number=w2833) -> (32bit integer=w2832:i32)
              n968 = Array Subset(array=w2835, length (row)=w2832) -> (w2836:u16[][])  [unwired: 3 in]
              n969 = call "myRIO_BRig_RT_comm_webdav_saveArrayToFile__2D_u16.vi"("Array"=w2836, "input_filename"="dataTrial") -> ()  [unwired: 10 in]
            }
          }
          n970 = case shown="True" w1052 {
            tunnel: w1048 -> [w1075 w1083]
            tunnel: w1051 -> [_ w1079]
            tunnel: w1050 -> [_ w1078]
            tunnel: w1049 -> [_ w1077]
            tunnel: w1018 -> [_ w1076]
            tunnel: [w1075 w1082] -> w1047
            tunnel: w1046 -> [w1074 w1081]
            tunnel: [w1074 w1080] -> w1045
            frame False {
            }
            frame True {
              n971 = call "myRIO_BRig_RT__Case_Exp__recordLick.vi"("intput_state__trialEnd"=w1076, "intput_state__trialStart"=w1077, "input_lick__R"=w1078, "input_lick__L"=w1079, "input_dataCurrent"=w1081, "input_dataLick"=w1083) -> ("output_dataCurrent"=w1080:u16[], "output_dataLick"=w1082:u16[][])  [unwired: 4 in]
            }
          }
          n972 = Or(x=w1020, y=w1021) -> (x .or. y?=w1007:bool)
          n973 = Or(x=w1024, y=w1004) -> (x .or. y?=w993:bool)
          n974 = Or(x=w1003, y=w1025) -> (x .or. y?=w1019:bool)
          n975 = Or(x=w1023, y=w1022) -> (x .or. y?=w1008:bool)
          n976 = Or(x=w1053, y="STOP_abort") -> (x .or. y?=w1055:bool)
          n977 = Or(x=w981, y=w982) -> (x .or. y?=w979:bool)
          n978 = Or(x=w983, y=w982) -> (x .or. y?=w980:bool)
          n979 = xnode "Read/Write Control"("FPGA VI Reference In"=w995, "error in"=w994, "A1_SR"=w1008, "A3_SL"=w1007, "A6_Act"=w992, "audioTrigger_L"=w993, "audioAmp_L"=w1034, "audioFreq_L_Hz"=w1002, "audioTrigger_R"=w1019, "audioAmp_R"=w1035, "audioFreq_R_Hz"=w1036, "laserledMTrig"=w979, "laserMTrig"=w980) -> ("FPGA VI Reference Out"=w1044:refnum<k20>, "error out"=w1043:errorcluster)
          n980 = node-c288() -> ()  [unwired: 1 in, 1 out]
          "cState" <- w1049
        }
        n981 = node-c288(w939) -> ()  [unwired: 1 out]
        n982 = flat-sequence {
          tunnel: w935 -> [w971]
          tunnel: w934 -> [w970]
          tunnel: [w969] -> w927
          tunnel: [w968] -> w926
          tunnel: [w975] -> w928
          tunnel: [w976] -> w933
          tunnel: w927 -> [w976]
          tunnel: w926 -> [w975]
          frame #0 {
            w972 = u16 0 ("AudioLeft_phase_inc")
            w967 = FALSE
            n983 = xnode "Read/Write Control"("FPGA VI Reference In"=w971, "error in"=w970, "Counts_Reset"=TRUE, "audioTrigger_L"=w967, "audioFreq_L_Hz"=w972, "audioAmp_L"=w972, "audioTrigger_R"=w967, "audioFreq_R_Hz"=w972, "audioAmp_R"=w972, "A3_SL"=w967, "A1_SR"=w967, "A6_Act"=w967) -> ("FPGA VI Reference Out"=w969:refnum<k20>, "error out"=w968:errorcluster)
          }
          frame #1 {
            w974 = FALSE ("START")
            n984 = local write "START"(w974) -> ()
            n985 = local write "STOP_endTrial"(w974) -> ()
            n986 = local write "STOP_endBlock"(w974) -> ()
          }
        }
        n987 = stacked-sequence {
          tunnel: w911 -> [w947 _]
          tunnel: w909 -> [w948 _]
          tunnel: w908 -> [_ w953]
          tunnel: w907 -> [_ w952]
          tunnel: w906 -> [_ w951]
          tunnel: w905 -> [w941 _]
          frame #0 {
            n988 = call "myRIO_BRig_RT_dataCurrent_idxDataLick.vi"() -> ("output_idxDataLick"=w942:i32)  [unwired: 11 in]
            n989 = Index Array(array=w941, index=w942) -> (element=w944:u16)
            n990 = Increment(x=w944) -> (x+1=w945:u16)
            n991 = call "myRIO_BRig_RT_comm_webdav_saveArrayToFile__1D_u16.vi"("Array"=w948, "input_filename"="dataMTrig") -> ()  [unwired: 10 in]
            n992 = To Long Integer(number=w945) -> (32bit integer=w943:i32)
            n993 = Array Subset(array=w947, length (row)=w943) -> (w946:u16[][])  [unwired: 3 in]
            n994 = call "myRIO_BRig_RT_comm_webdav_saveArrayToFile__2D_u16.vi"("Array"=w946, "input_filename"="dataLick") -> ()  [unwired: 10 in]
          }
          frame #1 {
            n995 = case shown="True" w953 {
              tunnel: w952 -> [_ w955]
              tunnel: w951 -> [_ w954]
              frame False {
              }
              frame True {
                n996 = stacked-sequence {
                  tunnel: w955 -> [w957 w964 w966]
                  tunnel: w954 -> [w958 w963 _]
                  frame #0 {
                    n997 = call "myRIO_BRig_RT_comm_webdav_uploadFile__announce.vi"("input_addText"=TRUE, "input_fileName_prefix"=w958, "intput_fileName"="curExp_end", "intput_hSession"=w957) -> ("output_Isuccess"=w956:bool)  [unwired: 6 in, 1 out]
                    n998 = case shown="True" w956 {
                      frame False {
                        n999 = One Button Dialog(message="!!! Warning !!! Your data is located at C:\\BehaviorRig\\commTransfer") -> ()  [unwired: 1 in, 1 out]
                      }
                      frame True {
                        n1000 = Wait (ms)(milliseconds to wait=u32 20) -> ()  [unwired: 1 out]
                      }
                    }
                  }
                  frame #1 {
                    n1001 = call "myRIO_BRig_RT__endExp_sendData.vi"("input_fileName_prefix"=w963, "input_hSession"=w964) -> ()  [unwired: 8 in, 2 out]
                  }
                  frame #2 {
                    n1002 = local write "Connected To Host?"(FALSE ("Connected To Host?")) -> ()
                    n1003 = call <vilib>:"Close Session.vi"("session handle"=w966) -> ()  [unwired: 14 in, 1 out]
                  }
                }
              }
            }
          }
        }
      }
    }
    n1004 = local read "STOP_abort"() -> (w30:bool)
  }
  n1005 = xnode "Read/Write Control"("FPGA VI Reference In"=w8, "error in"=w7, "FPGA_Stop"=TRUE) -> ("FPGA VI Reference Out"=w13:refnum<k20>, "error out"=w14:errorcluster)
  n1006 = xnode "Close FPGA VI Reference"("FPGA VI Reference In"=w13, "error in"=w14) -> ("error out"=w12:errorcluster)
  n1007 = call <vilib>:"Reset myRIO.vi"("error in (no error)"=w12) -> ()  [unwired: 10 in, 1 out]
